vi "main（新）.vi"(8 "停止 2":bool) -> ()   [LabVIEW 2016]
uses:
  <vilib>/Averna/Notify Icon/NotifyIcon.llb/BalloonIcon.ctl
  <vilib>/Utility/miscctls.llb/LVPointTypeDef.ctl
  <vilib>/Utility/config.llb/Read Key (String).vi
  <vilib>/Utility/config.llb/Read Key (I32).vi
  <vilib>/Utility/config.llb/Read Key (Boolean).vi
  <vilib>/Utility/config.llb/Write Key (String).vi
  <vilib>/Utility/config.llb/Write Key (U32).vi
  <vilib>/Utility/config.llb/Write Key (I32).vi
  <vilib>/Utility/config.llb/Write Key (Boolean).vi
  <vilib>/Averna/Notify Icon/NotifyIcon.llb/GetSelectedItemEvent.vi
  <vilib>/Averna/Notify Icon/NotifyIcon.llb/SetVisible.vi
  <vilib>/Averna/Notify Icon/NotifyIcon.llb/SetMenuDefaultItem.vi
  <vilib>/Averna/Notify Icon/NotifyIcon.llb/SetTipText.vi
  <vilib>/Averna/Notify Icon/NotifyIcon.llb/NotifyIcon.lvclass
  <vilib>/Utility/config.llb/NI_LVConfig.lvlib
  data/FreeMem.dll
  <vilib>/ptbypt/NI_PtbyPt.lvlib
panel:
  in  "数据发送协议":enum16{"2005-212协议", "2017-212协议"}(ring)=enum."2017-212协议"
  in  "数据发送通道":enum16{"TCP", "VISA"}(ring)
  in  "baud rate":u32=9600 caption="波特率"
  in  "VISA resource name":refnum<visa-resource-name> caption="VISA资源名称"
  in  "查询质控数据起始时间":bool
  in  "返回主界面":bool
  out "零点核查索引起始时间":string
  out "跨度核查索引起始时间":string
  out "加标回收索引起始时间":string
  out "标样核查索引起始时间":string
  out "数据接收超时指示灯":bool
  in  "重发时间":T1(ring)
  in  "重发日期":T2(ring)
  in  "锁":bool
  in  "开机启动":bool
  in  "确定更改起始时间":bool
  in  "更改起始时间":bool
  in  "数据发送起始时间":timestamp format="%<%.3X\n%Y/%m/%d>T"
  in  "每周自动重发":bool=TRUE
  in  "确定":bool
  in  "返回":bool
  in  "PW":string
  in  "MN":string
  in  "PORT":string
  in  "IP":string
  in  "站点设备":string
  in  "站点名称":string
  out "设置超时时间/min":i32=1
  in  "实时数据发送时间间隔/min":u32=1
  out "空闲时间/s":string
  out "状态信息":T3={"1st Error to Convert "=63, "步骤 "=enum."打开连接", "元素"="实时数据", "TCP服务端掉线计数"=4, "TCP掉线时间节点"="2019/05/08 15:24:17"} {"1st Error to Convert" items=["无错误", "参数错误", "内存已满", "超出区域", "文件结束", "文件已打开", "一般文件IO错误", "未找到文件", "文件权限错误", "磁盘已满", "路径副本", "打开过多文件", "未启用", "未找到资源文件", "无法添加资源", "未找到资源", "未找到图像", "图像内存错误", "画笔不存在", "配置错误类型", "配置未找到解析段", "配置解析错误", "配置内存错误", "错误外部代码格式", "错误外部代码偏移量", "外部代码不存在", "空窗口", "销毁窗口错误", "空菜单", "打印已中止", "错误打印记录", "打印驱动程序错误", "打印时窗口错误", "打印时内存错误", "打印对话框错误", "一般打印错误", "无效设备引用句柄", "设备未找到", "设备参数错误", "设备单位错误", "无法打开设备", "设备调用已中止", "一般错误", "用户已取消", "对象ID过低", "对象ID过高", "对象不在堆中", "未知的堆", "错误DefProc ID", "DefProc不在表格中", "范围外信息", "空方法", "未知信息", "不支持管理器调用", "错误地址", "连接过程中", "连接超时", "连接过程中", "不支持网络属性", "网络错误", "正在使用的地址", "系统缺少内存", "连接已中止", "连接已拒绝", "连接未建立", "连接已建立", "连接已关闭", "初始化错误（交互应用程序管理器）", "错误事件发生", "等待无约束事件发生处理程序", "事件发生队列溢出", "错误路径", "未发出信号量", "未识别类型（交互应用程序管理器）"]}
  out "系统时间":string
  out "实时小时数据上传":bool
  out "系统状态改变":bool
  out "软件版本":string
  out "掉线指示":bool
  out "核查数据上传":bool
  out "通信状态":bool
  out "重发数据":bool
  out "配置信息":T4
  in  "参数配置":bool
  out "查询数据发送":bool
  out "读取报文显示":string
  out "发送报文显示":string
  out "心跳包":bool
  in  "参数数值":T5={"CODMn"=TRUE, "CODCr"=TRUE, "DO"=TRUE, "DOperNULL"=TRUE, "PH"=TRUE, "氨氮"=TRUE, "比电导率"=TRUE, "水温"=TRUE, "盐度(海水)"=TRUE, "浊度"=TRUE, "总氮"=TRUE, "总磷"=TRUE, "叶绿素a"=TRUE, "藻密度"=TRUE, "水位"=TRUE, "流速"=TRUE, "瞬时流量"=TRUE, "累积流量"=TRUE}
  in  "系统编码选择框":string(combo)="地表水质量监测"
  out "主队列输出":refnum<queue>
  in  "TCP掉线时间节点":string
  out "TCP服务端掉线计数":i32
  out "元素":string
  out "步骤":T6(ring)
  out "1st Error to Convert":i32(ring)=56 items=["无错误", "参数错误", "内存已满", "超出区域", "文件结束", "文件已打开", "一般文件IO错误", "未找到文件", "文件权限错误", "磁盘已满", "路径副本", "打开过多文件", "未启用", "未找到资源文件", "无法添加资源", "未找到资源", "未找到图像", "图像内存错误", "画笔不存在", "配置错误类型", "配置未找到解析段", "配置解析错误", "配置内存错误", "错误外部代码格式", "错误外部代码偏移量", "外部代码不存在", "空窗口", "销毁窗口错误", "空菜单", "打印已中止", "错误打印记录", "打印驱动程序错误", "打印时窗口错误", "打印时内存错误", "打印对话框错误", "一般打印错误", "无效设备引用句柄", "设备未找到", "设备参数错误", "设备单位错误", "无法打开设备", "设备调用已中止", "一般错误", "用户已取消", "对象ID过低", "对象ID过高", "对象不在堆中", "未知的堆", "错误DefProc ID", "DefProc不在表格中", "范围外信息", "空方法", "未知信息", "不支持管理器调用", "错误地址", "连接过程中", "连接超时", "连接过程中", "不支持网络属性", "网络错误", "正在使用的地址", "系统缺少内存", "连接已中止", "连接已拒绝", "连接未建立", "连接已建立", "连接已关闭", "初始化错误（交互应用程序管理器）", "错误事件发生", "等待无约束事件发生处理程序", "事件发生队列溢出", "错误路径", "未发出信号量", "未识别类型（交互应用程序管理器）"]
  out "QN":string
  out "时间QN":string
  out "系统编码ST":string
  out "命令编码CN":string
  out "密码PW":string
  out "设备编码MN":string
  out "拆分包及应答Flag":string
  out "数据":string
  in  "实时数据参数选择框":T7={"水样测量数据"=FALSE, "零点核查数据"=TRUE, "跨度核查数据"=TRUE, "加标回收数据"=TRUE, "平行样数据"=FALSE, "标样核查"=TRUE}
  out "数据输出":string
  in  "table元素":string
  out "数组":string[](array[string])
  out "数组 2":string[](array[string])
  out "空闲时间":dbl
  out "错误输出":errorcluster
  out "error out":errorcluster
  # "读取的参数区"
  # "水样测量数据"
  # "零点核查数据"
  # "跨度核查数据"
  # "加标回收数据"
  # "平行样数据"
  # "标样核查"
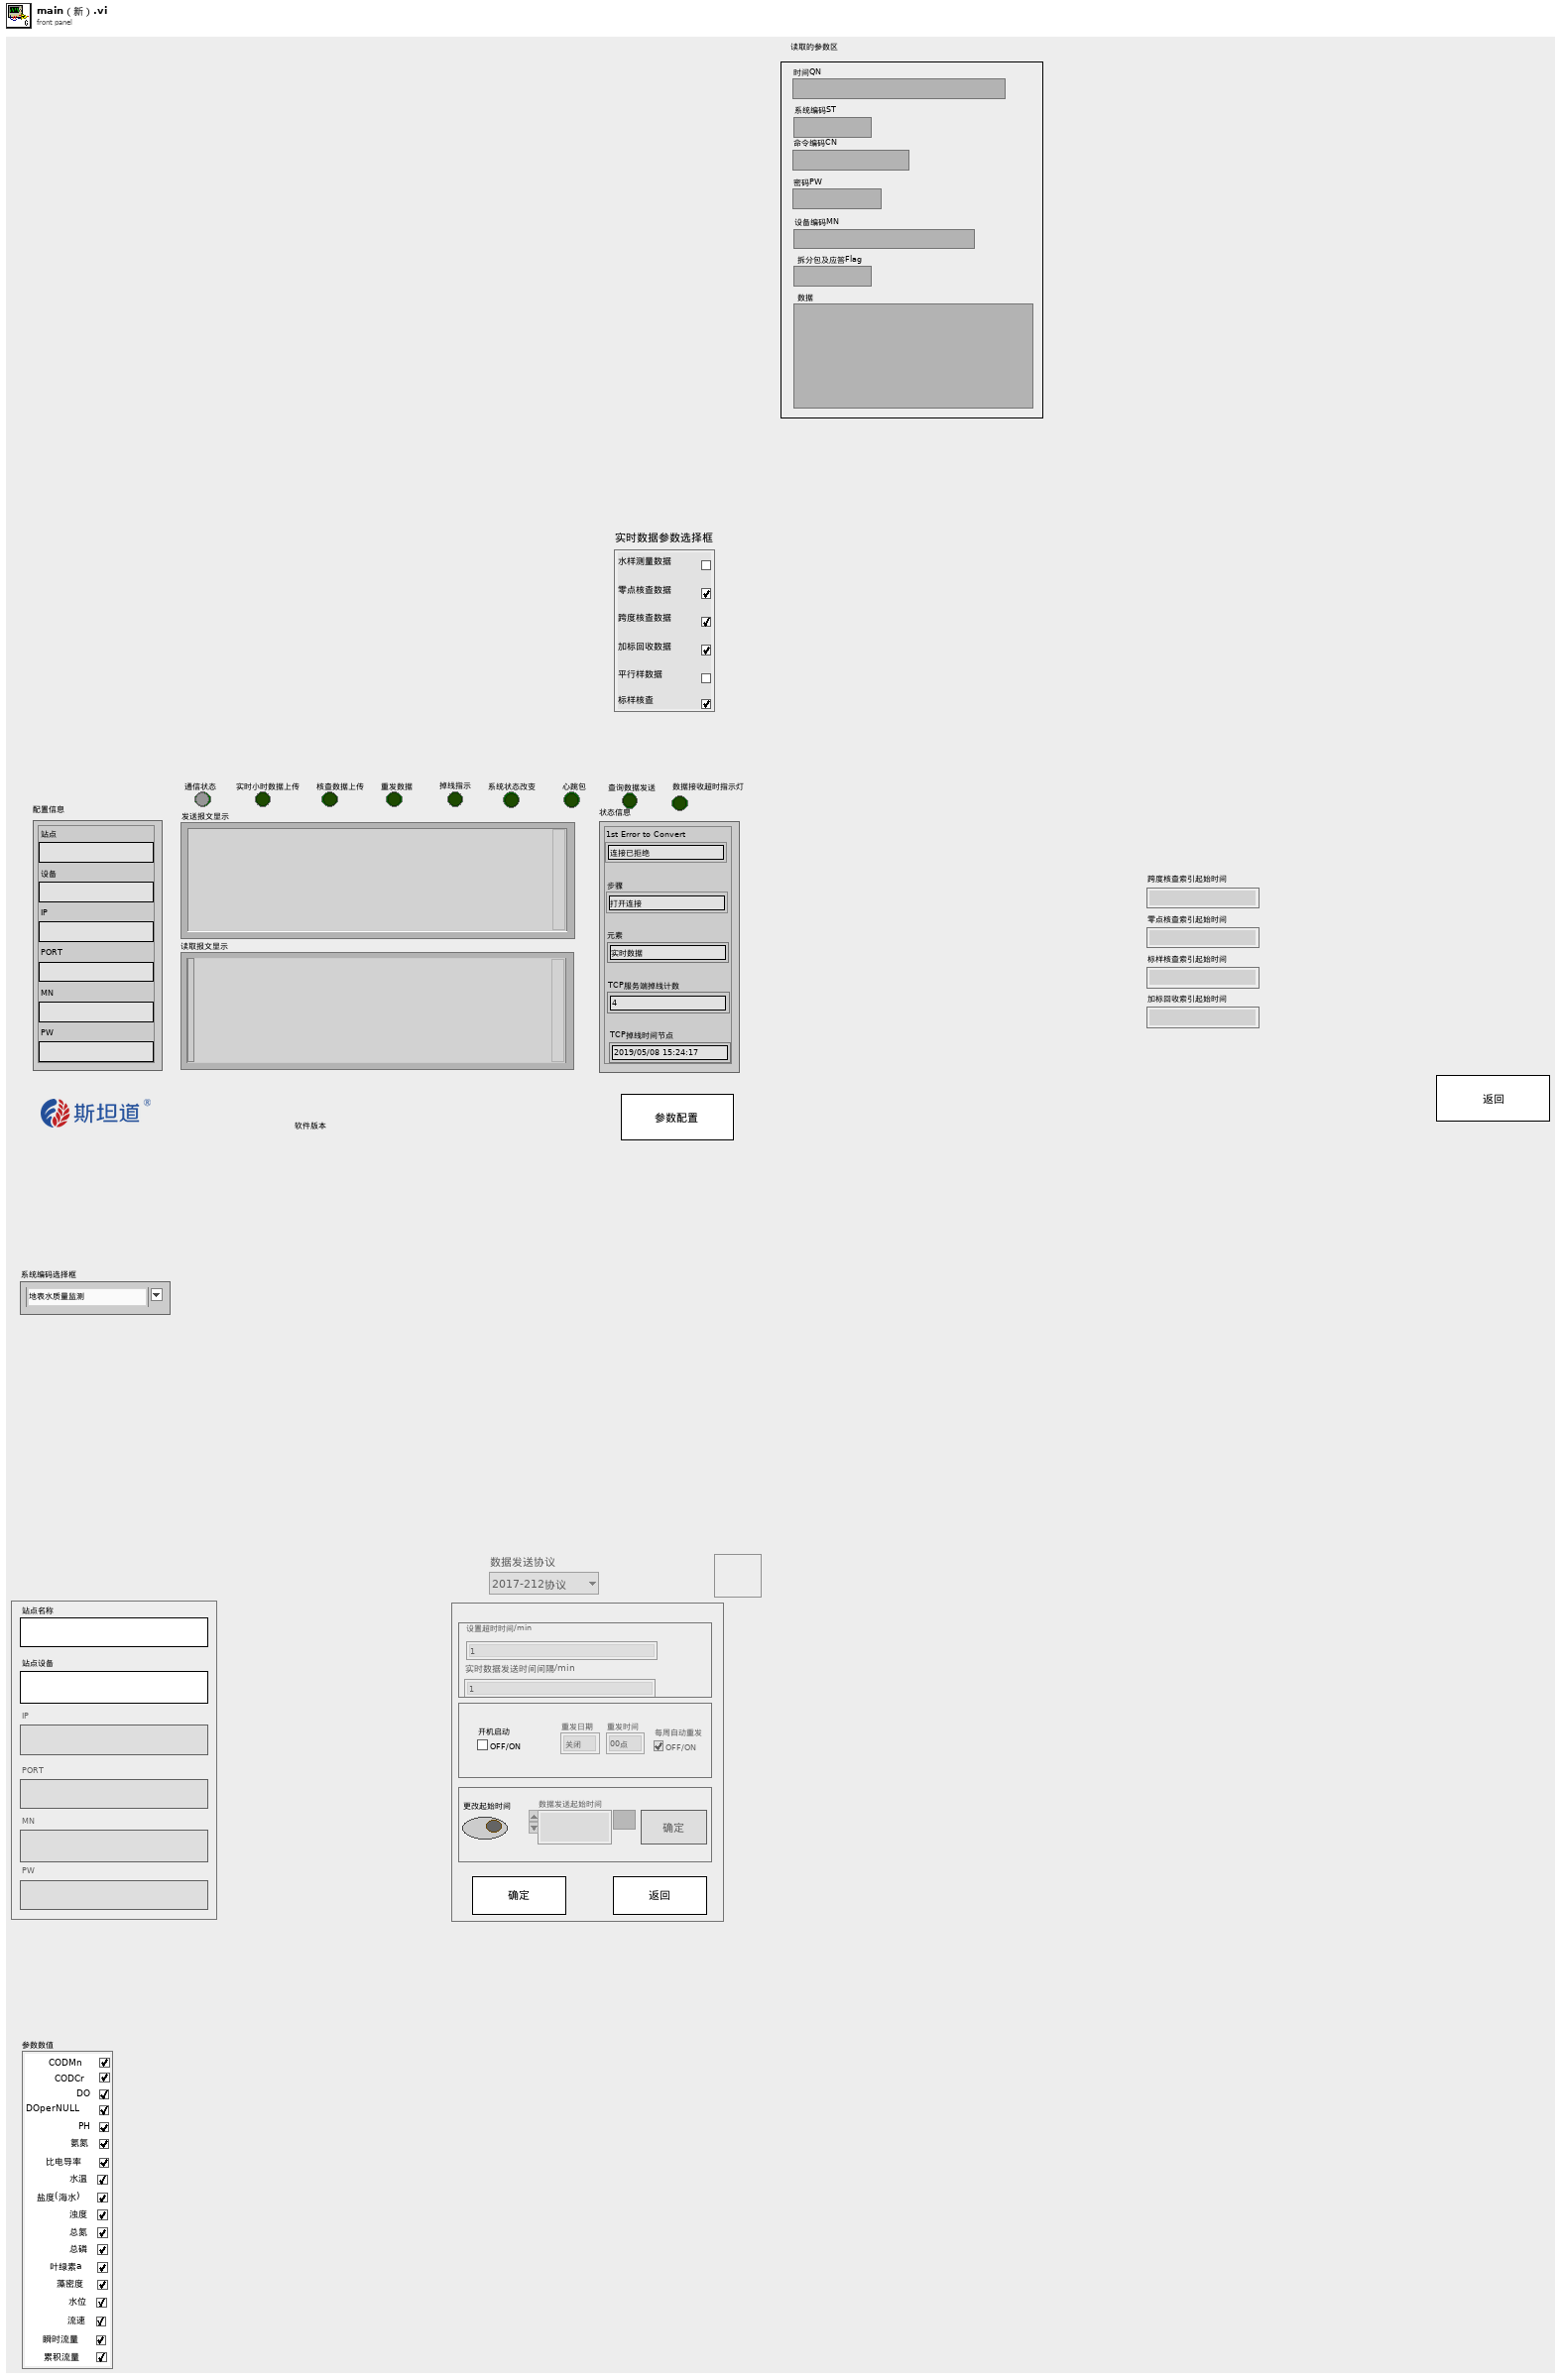
[diagram p1: front panel]
types:
  T1 = enum16{"00点", "01点", "02点", "03点", "04点", "05点", "06点", "07点", "08点", "09点", "10点", "11点", "12点", "13点", "14点", "15点", "16点", "17点", "18点", "19点", "20点", "21点", "22点", "23点"}
  T2 = enum16{"关闭", "星期日", "星期一", "星期二", "星期三", "星期四", "星期五", "星期六"}
  T3 = cluster{"1st Error to Convert ":i32, "步骤 ":enum16{"初始化", "打开连接", "表格比对", "发送数据", "读取数据", "数据处理"}, "元素":string, "TCP服务端掉线计数":i32, "TCP掉线时间节点":string}
  T4 = cluster{"站点":string, "设备":string, "IP":string, "PORT":string, "MN":string, "PW":string}
  T5 = cluster{"CODMn":bool, "CODCr":bool, "DO":bool, "DOperNULL":bool, "PH":bool, "氨氮":bool, "比电导率":bool, "水温":bool, "盐度(海水)":bool, "浊度":bool, "总氮":bool, "总磷":bool, "叶绿素a":bool, "藻密度":bool, "水位":bool, "流速":bool, "瞬时流量":bool, "累积流量":bool}
  T6 = enum16{"初始化", "打开连接", "表格比对", "发送数据", "读取数据", "数据处理"}
  T7 = cluster{"水样测量数据":bool, "零点核查数据":bool, "跨度核查数据":bool, "加标回收数据":bool, "平行样数据":bool, "标样核查":bool}
  T8 = typedef "NI_LVConfig.lvlib/Config Data RefNum.ctl" = refnum<k1>
  T9 = typedef "LVDateTimeRec.ctl" = cluster{"秒数的小数部分":dbl, "秒":i32, "分":i32, "时":i32, "日":i32, "月":i32, "年":i32, "天数（周）":i32, "天数（年）":i32, "DST":i32}
  T10 = cluster{"PH":string[][], "CODCr":string[][], "氨氮":string[][], "CODMn":string[][], "总氮":string[][], "总磷":string[][], "电导率":string[][], "水温":string[][], "DO":string[][], "浊度":string[][], "叶绿素":string[][], "藻密度":string[][], "DOper":string[][], "盐度":string[][], "水位":string[][], "流速":string[][], "瞬时流量":string[][], "累积流量":string[][]}
  T11 = typedef "LVPointTypeDef.ctl" = cluster{"Horizontal":i16, "Vertical":i16}
  T12 = enum8{"Enabled", "Disabled", "Disabled and Grayed Out"}
  T13 = typedef "imagedata.ctl" = cluster{"image type":i32, "image depth":i32, "image":u8[], "mask":u8[], "colors":u32[], "Rectangle":cluster{"left":i16, "top":i16, "right":i16, "bottom":i16}}
  T14 = enum32{"invalid app kind", "Development System", "Run Time System", "Student Edition", "Embedded LabVIEW", "Evaluation", "Custom"}
  T15 = enum32{"Invalid", "Standard", "Closed", "Hidden", "Minimized", "Maximized"}
  T16 = enum16{"水样测试", "小时数据", "日志信息", "报警信息", "零点核查", "标样核查", "平行样", "加标回收"}
  T17 = enum16{"CODMn", "CODCr", "氨氮", "总磷", "总氮", "数采仪"}
  T18 = cluster{"高锰酸盐":string, "化学需氧量":string, "氨氮":string, "总磷":string, "总氮":string, "数采仪":string, "高锰酸盐":bool, "化学需氧量":bool, "氨氮":bool, "总磷":bool, "总氮":bool, "数采仪":bool}
  T19 = typedef "NotifyIcon.lvlib/NotifyIcon.lvclass/BalloonIcon.ctl" = enum32{"None", "Information", "Warning", "Error"}
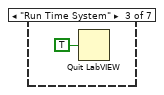
[diagram p5: hidden frame]
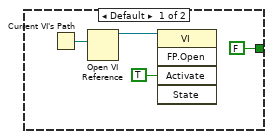
[diagram p10: hidden frame]
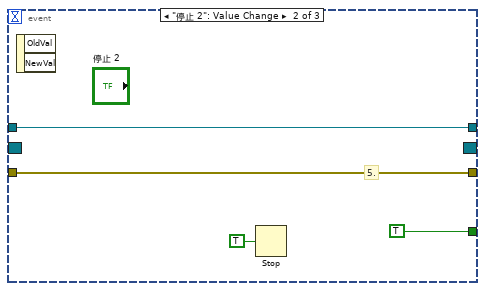
[diagram p11: hidden frame]
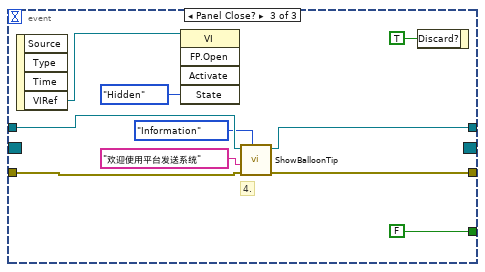
[diagram p12: hidden frame]
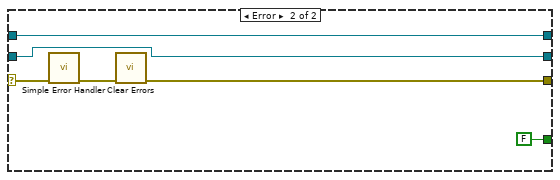
[diagram p13: hidden frame]
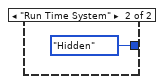
[diagram p14: hidden frame]
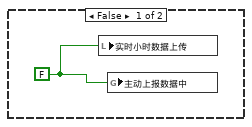
[diagram p15: hidden frame]
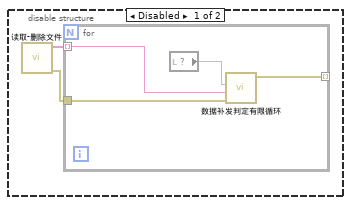
[diagram p16: hidden frame]
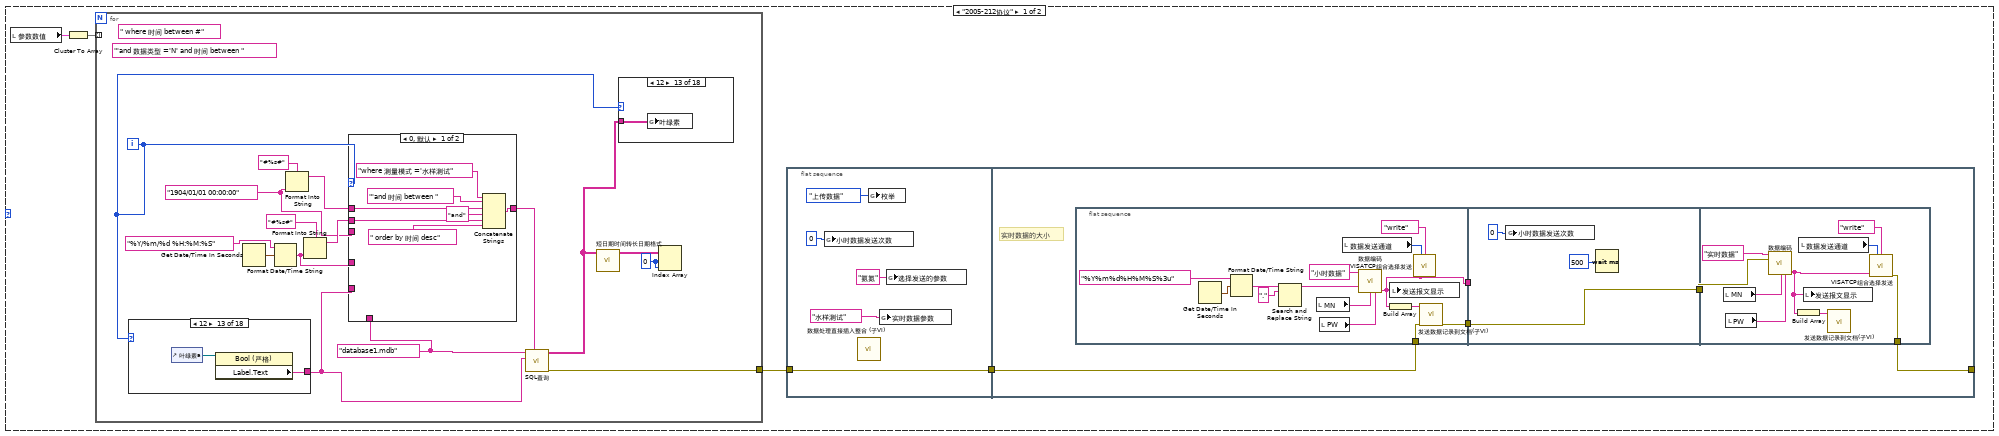
[diagram p17: hidden frame]
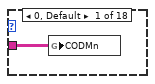
[diagram p18: hidden frame]
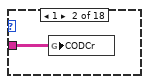
[diagram p19: hidden frame]
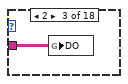
[diagram p20: hidden frame]
diagram:
  w23 = string[] ["OPEN线程一", "APP_SEPARATOR", "EXIT线程一"]
  (unwired) string[] ["CODMn", "CODCr", "DO", "DOper", "PH", "氨氮", "电导率", "水温", "盐度", "浊度", "总氮", "总磷", "叶绿素a", "藻密度", "水位", "流速", "瞬时流量", "累积流量"] ("查询参数数组")
  (unwired) 0 items=["无错误", "参数错误", "内存已满", "超出区域", "文件结束", "文件已打开", "一般文件IO错误", "未找到文件", "文件权限错误", "磁盘已满", "路径副本", "打开过多文件", "未启用", "未找到资源文件", "无法添加资源", "未找到资源", "未找到图像", "图像内存错误", "画笔不存在", "配置错误类型", "配置未找到解析段", "配置解析错误", "配置内存错误", "错误外部代码格式", "错误外部代码偏移量", "外部代码不存在", "空窗口", "销毁窗口错误", "空菜单", "打印已中止", "错误打印记录", "打印驱动程序错误", "打印时窗口错误", "打印时内存错误", "打印对话框错误", "一般打印错误", "无效设备引用句柄", "设备未找到", "设备参数错误", "设备单位错误", "无法打开设备", "设备调用已中止", "一般错误", "用户已取消", "对象ID过低", "对象ID过高", "对象不在堆中", "未知的堆", "错误DefProc ID", "DefProc不在表格中", "范围外信息", "空方法", "未知信息", "不支持管理器调用", "错误地址", "连接过程中", "连接超时", "连接过程中", "不支持网络属性", "网络错误", "正在使用的地址", "系统缺少内存", "连接已中止", "连接已拒绝", "连接未建立", "连接已建立", "连接已关闭", "初始化错误（交互应用程序管理器）", "错误事件发生", "等待无约束事件发生处理程序", "事件发生队列溢出", "错误路径", "未发出信号量", "未识别类型（交互应用程序管理器）"] ("1st Error to Convert")
  # "6."
  # "3."
  # "1."
  # "判定当数据没有传送完毕并掉线，将数据存储入临时表格"
  # "上传本地时间点的实时数据"
  # "目前时间太短，如果掉线了，数据存不了临时表格"
  # "3.表格中数据较多的情况下，数据补发送需要分批发送"
  # "1.发送数据过程中突然掉线（如果是查询之后的服务端掉线，不作处理；如果是整点主动上传时掉线，标记数据接收中断，然后数据存入表格）\n2.在查询过程中到了整点要发数据怎么处理（判定查询数据发送完全再进行出列队读取数据）\n3.一般情况掉线，数据存储入临时表格，上线了重发"
  # "获取需要发送的数据表"
  n1 = Cluster To Array(cluster="参数数值") -> (array=w33:bool[])
  n2 = for {
    tunnel: w33 -> [_] mode=indexing
    tunnel: [w73] -> w32
    i -> [w73]
    w62 = "线程一数据重发功能" ("section")
    n3 = case shown="8" w73 {
      tunnel: [w104 w106 w108 w110 w112 w114 w116 w118 w120 w122 w124 w126 w128 w130 w132 w134 w136 w138] -> w77
      frame 0, Default {
        n4 = control-ref of="CODMn"() -> (w105:refnum<vi>)
        n5 = property class="Bool (严格)"(reference=w105) -> ("Label.Text"=w104:string)  [unwired: 1 in, 2 out]
      }
      frame 1 {
        n6 = control-ref of="CODCr"() -> (w107:refnum<vi>)
        n7 = property class="Bool (严格)"(reference=w107) -> ("Label.Text"=w106:string)  [unwired: 1 in, 2 out]
      }
      frame 2 {
        n8 = control-ref of="DO"() -> (w109:refnum<vi>)
        n9 = property class="Bool (严格)"(reference=w109) -> ("Label.Text"=w108:string)  [unwired: 1 in, 2 out]
      }
      frame 3 {
        n10 = control-ref of="DOperNULL"() -> (w111:refnum<vi>)
        n11 = property class="Bool (严格)"(reference=w111) -> ("Label.Text"=w110:string)  [unwired: 1 in, 2 out]
      }
      frame 4 {
        n12 = control-ref of="PH"() -> (w113:refnum<vi>)
        n13 = property class="Bool (严格)"(reference=w113) -> ("Label.Text"=w112:string)  [unwired: 1 in, 2 out]
      }
      frame 5 {
        n14 = control-ref of="氨氮"() -> (w115:refnum<vi>)
        n15 = property class="Bool (严格)"(reference=w115) -> ("Label.Text"=w114:string)  [unwired: 1 in, 2 out]
      }
      frame 6 {
        n16 = control-ref of="比电导率"() -> (w117:refnum<vi>)
        n17 = property class="Bool (严格)"(reference=w117) -> ("Label.Text"=w116:string)  [unwired: 1 in, 2 out]
      }
      frame 7 {
        n18 = control-ref of="水温"() -> (w119:refnum<vi>)
        n19 = property class="Bool (严格)"(reference=w119) -> ("Label.Text"=w118:string)  [unwired: 1 in, 2 out]
      }
      frame 8 {
        n20 = control-ref of="盐度(海水)"() -> (w121:refnum<vi>)
        n21 = property class="Bool (严格)"(reference=w121) -> ("Label.Text"=w120:string)  [unwired: 1 in, 2 out]
      }
      frame 9 {
        n22 = control-ref of="浊度"() -> (w123:refnum<vi>)
        n23 = property class="Bool (严格)"(reference=w123) -> ("Label.Text"=w122:string)  [unwired: 1 in, 2 out]
      }
      frame 10 {
        n24 = control-ref of="总氮"() -> (w125:refnum<vi>)
        n25 = property class="Bool (严格)"(reference=w125) -> ("Label.Text"=w124:string)  [unwired: 1 in, 2 out]
      }
      frame 11 {
        n26 = control-ref of="总磷"() -> (w127:refnum<vi>)
        n27 = property class="Bool (严格)"(reference=w127) -> ("Label.Text"=w126:string)  [unwired: 1 in, 2 out]
      }
      frame 12 {
        n28 = control-ref of="叶绿素a"() -> (w129:refnum<vi>)
        n29 = property class="Bool (严格)"(reference=w129) -> ("Label.Text"=w128:string)  [unwired: 1 in, 2 out]
      }
      frame 13 {
        n30 = control-ref of="藻密度"() -> (w131:refnum<vi>)
        n31 = property class="Bool (严格)"(reference=w131) -> ("Label.Text"=w130:string)  [unwired: 1 in, 2 out]
      }
      frame 14 {
        n32 = control-ref of="水位"() -> (w133:refnum<vi>)
        n33 = property class="Bool (严格)"(reference=w133) -> ("Label.Text"=w132:string)  [unwired: 1 in, 2 out]
      }
      frame 15 {
        n34 = control-ref of="流速"() -> (w135:refnum<vi>)
        n35 = property class="Bool (严格)"(reference=w135) -> ("Label.Text"=w134:string)  [unwired: 1 in, 2 out]
      }
      frame 16 {
        n36 = control-ref of="瞬时流量"() -> (w137:refnum<vi>)
        n37 = property class="Bool (严格)"(reference=w137) -> ("Label.Text"=w136:string)  [unwired: 1 in, 2 out]
      }
      frame 17 {
        n38 = control-ref of="累积流量"() -> (w139:refnum<vi>)
        n39 = property class="Bool (严格)"(reference=w139) -> ("Label.Text"=w138:string)  [unwired: 1 in, 2 out]
      }
    }
    n40 = call <vilib>:"Application Directory.vi"() -> ("Application Directory"=w83:path)
    n41 = Build Path(base path=w83, name or relative path="data\\Set.ini" ("名称或相对路径")) -> (appended path=w81:path)
    n42 = call <vilib>:"Open Config Data.vi"("configuration file path"=w81) -> ("error out"=w79:errorcluster, "refnum"=w80:T8)  [unwired: 8 in, 1 out]
    n43 = call-poly <vilib>:"Read Key.vi"("section"="线程一数据搜索起始时间", "error in (no error)"=w79, "key"=w77, "refnum"=w80) -> ("error out"=w71:errorcluster, "value"=w74:string, "refnum out"=w72:T8)  [unwired: 4 in, 1 out]
    n44 = Empty String/Path?(string/path=w74) -> (empty?=w76:bool)
    n45 = case shown="真" w76 {
      tunnel: [w84 "1904/01/01 00:00:00"] -> w75
      tunnel: w74 -> [w84 _]
      frame False {
      }
      frame True {
      }
    }
    n46 = call-poly <vilib>:"Read Key.vi"("section"=w62, "error in (no error)"=w71, "key"="重发功能", "refnum"=w72) -> ("error out"=w65:errorcluster, "value"=w69:bool, "refnum out"=w66:T8)  [unwired: 4 in, 1 out]
    n47 = local write "每周自动重发"(w69) -> ()
    n48 = call-poly <vilib>:"Read Key.vi"("section"=w62, "error in (no error)"=w65, "key"="重发日期", "refnum"=w66) -> ("error out"=w63:errorcluster, "value"=w59:i32, "refnum out"=w64:T8)  [unwired: 4 in, 1 out]
    n49 = local write "重发日期"(w59) -> ()
    n50 = case shown="0, 默认" w73 {
      tunnel: w75 -> [w86 w87 w88 w89 w90 w91 w92 w93 w94 w95 w96 w97 w98 w99 w100 w101 w102 w103]
      frame 0, Default {
        n51 = global write "全局 水样时间.vi" "time1"(w86) -> ()
      }
      frame 1 {
        n52 = global write "全局 水样时间.vi" "time2"(w87) -> ()
      }
      frame 2 {
        n53 = global write "全局 水样时间.vi" "time3"(w88) -> ()
      }
      frame 3 {
        n54 = global write "全局 水样时间.vi" "time4"(w89) -> ()
      }
      frame 4 {
        n55 = global write "全局 水样时间.vi" "time5"(w90) -> ()
      }
      frame 5 {
        n56 = global write "全局 水样时间.vi" "time6"(w91) -> ()
      }
      frame 6 {
        n57 = global write "全局 水样时间.vi" "time7"(w92) -> ()
      }
      frame 7 {
        n58 = global write "全局 水样时间.vi" "time8"(w93) -> ()
      }
      frame 8 {
        n59 = global write "全局 水样时间.vi" "time9"(w94) -> ()
      }
      frame 9 {
        n60 = global write "全局 水样时间.vi" "time10"(w95) -> ()
      }
      frame 10 {
        n61 = global write "全局 水样时间.vi" "time11"(w96) -> ()
      }
      frame 11 {
        n62 = global write "全局 水样时间.vi" "time12"(w97) -> ()
      }
      frame 12 {
        n63 = global write "全局 水样时间.vi" "time13"(w98) -> ()
      }
      frame 13 {
        n64 = global write "全局 水样时间.vi" "time14"(w99) -> ()
      }
      frame 14 {
        n65 = global write "全局 水样时间.vi" "time15"(w100) -> ()
      }
      frame 15 {
        n66 = global write "全局 水样时间.vi" "time16"(w101) -> ()
      }
      frame 16 {
        n67 = global write "全局 水样时间.vi" "time17"(w102) -> ()
      }
      frame 17 {
        n68 = global write "全局 水样时间.vi" "time18"(w103) -> ()
      }
    }
    n69 = call-poly <vilib>:"Read Key.vi"("section"=w62, "error in (no error)"=w63, "key"="重发时间", "refnum"=w64) -> ("error out"=w60:errorcluster, "value"=w58:i32, "refnum out"=w61:T8)  [unwired: 4 in, 1 out]
    n70 = local write "重发时间"(w58) -> ()
    n71 = call <vilib>:"Close Config Data.vi"("error in (no error)"=w60, "refnum"=w61) -> ()  [unwired: 8 in, 2 out]
  }
  n72 = Obtain Queue(name (unnamed)="数据发送" ("名称（未命名）"), element data type="") -> (queue out=w38:refnum<queue>, error out=w37:errorcluster)  [unwired: 3 in, 1 out]
  n73 = Obtain Queue(name (unnamed)="实时数据参数选择" ("名称（未命名）"), element data type="") -> (queue out=w39:refnum<queue>, error out=w36:errorcluster)  [unwired: 3 in, 1 out]
  n74 = while {
    tunnel: w38 -> [w142]
    stop <- FALSE stop-if-true
    # "和工控机通讯系统状态改变主动上传"
    # "整点发送小时数据(禁用）"
    n75 = Multiply(x=u32 1, y=u32 1000 ("等待时间（毫秒）")) -> (x*y=w148:u32)
    n76 = case shown="真" "每周自动重发" {
      frame False {
      }
      frame True {
        (unwired) T1."00点"
        (unwired) T2."关闭"
        n77 = Get Date/Time In Seconds() -> (seconds since 1Jan1904=w211:timestamp)
        n78 = Seconds To Date/Time(time stamp (now)=w211) -> (date time rec=w205:T9)  [unwired: 1 in]
        n79 = Unbundle By Name(w205) -> ("天数（周）"=w210:i32, "时"=w200:i32, "分"=w209:i32)
        n80 = Equal To 0?(x=w209) -> (x = 0?=w206:bool)
        n81 = Equal?(x=w210, y="重发日期") -> (x = y?=w208:bool)
        n82 = Equal?(x=w200, y="重发时间") -> (x = y?=w207:bool)
        n83 = Compound Arithmetic op=AND ("复合运算")(w208, w207, w206) -> (w204:bool)
        n84 = call <vilib>:"Boolean Crossing PtByPt.vi"("direction"=enum16{"either", "false-true", "true-false"}."false-true", "input"=w204) -> ("crossing"=w203:bool)  [unwired: 1 in]
        n85 = case shown="真" w203 {
          tunnel: w205 -> [_ w213]
          frame False {
          }
          frame True {
            n86 = local read "参数数值"() -> (w218:T5)
            n87 = Unbundle By Name(w213) -> ("日"=w216:i32)
            n88 = Cluster To Array(cluster=w218) -> (array=w219:bool[])
            n89 = Subtract(x=w216, y=7) -> (x-y=w214:i32)
            n90 = Bundle By Name(cluster=w213, "日"=w214) -> (w217:T9)
            n91 = Date/Time To Seconds(2:w217) -> (0:w212:timestamp)  [unwired: 1 in]
            n92 = for {
              tunnel: w219 -> [_] mode=indexing
              tunnel: w212 -> [w220]
              i -> [w221]
              n93 = Format Date/Time String(time format string (%c)="%Y/%m/%d %H:%M:%S" ("时间格式字符串(%c)"), seconds (now)=w220) -> (date/time string=w222:string)  [unwired: 1 in]
              n94 = case shown="16" w221 {
                tunnel: w222 -> [w224 w225 w226 w227 w228 w229 w230 w231 w232 w233 w234 w235 w236 w237 w238 w239 w240 w241]
                frame 0, Default {
                  n95 = global write "全局 水样时间.vi" "time1"(w224) -> ()
                }
                frame 1 {
                  n96 = global write "全局 水样时间.vi" "time2"(w225) -> ()
                }
                frame 2 {
                  n97 = global write "全局 水样时间.vi" "time3"(w226) -> ()
                }
                frame 3 {
                  n98 = global write "全局 水样时间.vi" "time4"(w227) -> ()
                }
                frame 4 {
                  n99 = global write "全局 水样时间.vi" "time5"(w228) -> ()
                }
                frame 5 {
                  n100 = global write "全局 水样时间.vi" "time6"(w229) -> ()
                }
                frame 6 {
                  n101 = global write "全局 水样时间.vi" "time7"(w230) -> ()
                }
                frame 7 {
                  n102 = global write "全局 水样时间.vi" "time8"(w231) -> ()
                }
                frame 8 {
                  n103 = global write "全局 水样时间.vi" "time9"(w232) -> ()
                }
                frame 9 {
                  n104 = global write "全局 水样时间.vi" "time10"(w233) -> ()
                }
                frame 10 {
                  n105 = global write "全局 水样时间.vi" "time11"(w234) -> ()
                }
                frame 11 {
                  n106 = global write "全局 水样时间.vi" "time12"(w235) -> ()
                }
                frame 12 {
                  n107 = global write "全局 水样时间.vi" "time13"(w236) -> ()
                }
                frame 13 {
                  n108 = global write "全局 水样时间.vi" "time14"(w237) -> ()
                }
                frame 14 {
                  n109 = global write "全局 水样时间.vi" "time15"(w238) -> ()
                }
                frame 15 {
                  n110 = global write "全局 水样时间.vi" "time16"(w239) -> ()
                }
                frame 16 {
                  n111 = global write "全局 水样时间.vi" "time17"(w240) -> ()
                }
                frame 17 {
                  n112 = global write "全局 水样时间.vi" "time18"(w241) -> ()
                }
              }
            }
          }
        }
      }
    }
    n113 = Wait (ms)(milliseconds to wait=w148) -> ()  [unwired: 1 out]
    n114 = call "Modbus Master.vi"("Unit ID"=u8 1, "读取写入选择"="读取") -> ("register values"=w143:u16[], "error out"=w140:errorcluster)  [unwired: 8 in]
    n115 = case shown="无错误" w140 {
      tunnel: w143 -> [w152 _]
      tunnel: w142 -> [w150 _]
      frame No Error {
        # "防止由于MBtcp错误导致状态为0发送至平台"
        n116 = global read "全局1.vi" "register values"() -> (w151:u16[])
        n117 = flat-sequence {
          tunnel: w152 -> [w158]
          tunnel: w151 -> [w178]
          tunnel: w150 -> [w154]
          tunnel: [w158] -> w153
          tunnel: w153 -> [w198]
          frame #0 {
            n118 = Index Array(array=w158) -> (element #1=w165:u16, element #2=w177:u16, element #3=w176:u16, element #4=w175:u16, element #5=w174:u16, element #6=w173:u16, element #7=w163:u16, element #8=w157:u16)  [unwired: 8 in]
            n119 = Index Array(array=w178) -> (element #1=w164:u16, element #2=w172:u16, element #3=w171:u16, element #4=w170:u16, element #5=w169:u16, element #6=w168:u16, element #7=w162:u16, element #8=w156:u16)  [unwired: 8 in]
            n120 = Build Array(w177, w176, w175, w174, w173) -> (w167:u16[])
            n121 = Build Array(w172, w171, w170, w169, w168) -> (w166:u16[])
            n122 = Not Equal?(x=w165, y=w164) -> (x != y?=w160:bool)
            n123 = Not Equal?(x=w163, y=w162) -> (x != y?=w161:bool)
            n124 = Not Equal?(x=w157, y=w156) -> (x != y?=w155:bool)
            n125 = Not Equal?(x=w167, y=w166) -> (x != y?=w159:bool[])
            n126 = while {
              tunnel: w154 -> [w187]
              tunnel: w159 -> [w184] mode=indexing
              i -> [w186]
              stop <- w182 stop-if-true
              n127 = Greater Or Equal?(x=w186, y=4) -> (x >= y?=w183:bool)
              n128 = Or(x=w184, y=w183) -> (x .or. y?=w182:bool)
              n129 = case shown="真" w184 {
                tunnel: w187 -> [_ w189]
                frame False {
                }
                frame True {
                  n130 = local write "系统状态改变"(TRUE ("系统状态改变")) -> ()
                  n131 = Enqueue Element(queue=w189, element="系统状态" ("元素")) -> ()  [unwired: 2 in, 3 out]
                }
              }
            }
            n132 = case shown="真" w160 {
              tunnel: w154 -> [_ w195]
              frame False {
              }
              frame True {
                n133 = Enqueue Element(queue=w195, element="运行模式" ("元素")) -> ()  [unwired: 2 in, 3 out]
                "系统状态改变" <- TRUE
              }
            }
            n134 = case shown="真" w155 {
              tunnel: w154 -> [_ w180]
              frame False {
              }
              frame True {
                n135 = local write "系统状态改变"(TRUE ("系统状态改变")) -> ()
                n136 = Enqueue Element(queue=w180, element="超标留样" ("元素")) -> ()  [unwired: 2 in, 3 out]
              }
            }
            n137 = case shown="真" w161 {
              tunnel: w154 -> [_ w192]
              frame False {
              }
              frame True {
                n138 = local write "系统状态改变"(TRUE ("系统状态改变")) -> ()
                n139 = Enqueue Element(queue=w192, element="测量周期" ("元素")) -> ()  [unwired: 2 in, 3 out]
              }
            }
          }
          frame #1 {
            n140 = global write "全局1.vi" "register values"(w198) -> ()
            n141 = local write "系统状态改变"(FALSE ("系统状态改变")) -> ()
          }
        }
      }
      frame Error {
      }
    }
  }
  n142 = while {
    tunnel: w38 -> [w255]
    stop <- FALSE stop-if-true
    # "核查和质控数据的定期发送在实时数据周期上传"
    # "指定周期发一次核查数据"
    n143 = local read "查询数据发送"() -> (w250:bool)
    n144 = local read "实时小时数据上传"() -> (w254:bool)
    n145 = local read "重发数据"() -> (w251:bool)
    n146 = Multiply(x="实时数据发送时间间隔/min", y=u32 60000 ("等待时间（毫秒）")) -> (x*y=w258:u32)
    n147 = local read "步骤"() -> (w249:T6)
    n148 = Not(x=w250) -> (.not. x?=w246:bool)
    n149 = Wait (ms)(milliseconds to wait=w258) -> ()  [unwired: 1 out]
    n150 = Not(x=w251) -> (.not. x?=w245:bool)
    n151 = Not(x=w254) -> (.not. x?=w252:bool)
    n152 = First Call?() -> (First Call?: T/F=w256:bool)
    n153 = Equal?(x=w249, y=T6."读取数据" ("步骤")) -> (x = y?=w247:bool)
    n154 = case shown="真" w256 {
      tunnel: w255 -> [_ _]
      frame False {
      }
      frame True {
        w274 = "1994/01/01 00:00:00"
        n155 = global write "全局 时间2.vi" "跨度核查索引起始时间"(w274) -> ()
        n156 = global write "全局 时间2.vi" "零点核查索引起始时间"(w274) -> ()
        n157 = global write "全局 时间2.vi" "平行样索引起始时间"(w274) -> ()
        n158 = global write "全局 时间2.vi" "加标回收索引起始时间"(w274) -> ()
        n159 = global write "全局 时间2.vi" "标样核查索引起始时间"(w274) -> ()
      }
    }
    n160 = local read "数据发送协议"() -> (w244:enum16{"2005-212协议", "2017-212协议"})
    n161 = Equal?(x=w244, y=enum16{"2005-212协议", "2017-212协议"}."2017-212协议" ("数据发送协议")) -> (x = y?=w242:bool)
    n162 = Compound Arithmetic op=AND ("复合运算")(w242, w245, w246, w247, w252) -> (w253:bool)
    n163 = case shown="真" w253 {
      tunnel: w255 -> [_ w270]
      frame False {
      }
      frame True {
        n164 = call "实时数据参数入列队.vi"("发送实时数据选择框"="实时数据参数选择框") -> ("错误输出"=w272:errorcluster)  [unwired: 10 in]
        n165 = call <vilib>:"Clear Errors.vi"("error in (no error)"=w272) -> ()  [unwired: 5 in, 2 out]
        n166 = Enqueue Element(queue=w270, element="send" ("元素")) -> (queue out=w267:refnum<queue>, error out=w266:errorcluster)  [unwired: 2 in, 1 out]
        n167 = Enqueue Element(queue=w267, element="操作日志" ("元素"), error in (no error)=w266) -> (queue out=w264:refnum<queue>, error out=w263:errorcluster)  [unwired: 1 in, 1 out]
        n168 = Enqueue Element(queue=w264, element="仪器参数" ("元素"), error in (no error)=w263) -> (queue out=w262:refnum<queue>, error out=w261:errorcluster)  [unwired: 1 in, 1 out]
        n169 = Enqueue Element(queue=w262, element="报警信息" ("元素"), error in (no error)=w261) -> ()  [unwired: 1 in, 3 out]
      }
    }
  }
  n170 = while "While循环" {
    tunnel: w38 -> [w287]
    tunnel: w39 -> [w291]
    tunnel: w37 -> [w290]
    tunnel: w36 -> [w289]
    stop <- FALSE stop-if-true
    # "判定数据发送时要发送实时数据"
    # "所有的主动上传数据都是有数据才会上传"
    n171 = Get Queue Status(queue=w287) -> (# elements in queue=w279:i32)  [unwired: 2 in, 7 out]
    n172 = local read "查询数据发送"() -> (w285:bool)
    n173 = global read "全局 数据发送重叠.vi" "主动上报数据中"() -> (w277:bool)
    n174 = local read "重发数据"() -> (w276:bool)
    n175 = Not Equal To 0?(x=w279) -> (x != 0?=w286:bool)
    n176 = And(x=w286, y=w285) -> (x .and. y?=w278:bool)
    n177 = call <vilib>:"Boolean Crossing PtByPt.vi"("direction"=enum16{"either", "false-true", "true-false"}."false-true", "input"=w278) -> ("crossing"=w284:bool)  [unwired: 1 in]
    n178 = Not(x=w277) -> (.not. x?=w281:bool)
    n179 = Not(x=w276) -> (.not. x?=w275:bool)
    n180 = Not(x=w285) -> (.not. x?=w282:bool)
    n181 = case shown="真" w284 {
      frame False {
      }
      frame True {
        n182 = Get Date/Time In Seconds() -> (seconds since 1Jan1904=w294:timestamp)
        n183 = Format Date/Time String(time format string (%c)="%Y%m%d%H%M%S%3u" ("时间格式字符串(%c)"), seconds (now)=w294) -> (date/time string=w298:string)  [unwired: 1 in]
        n184 = Search and Replace String(input string=w298, search string="." ("搜索字符串")) -> (result string=w297:string)  [unwired: 6 in, 3 out]
        n185 = call "格式时间字符串.vi"("字符串"=w297) -> ("连接的字符串"=w293:string)  [unwired: 10 in]
        n186 = global write "全局 数据发送重叠.vi" "数据发送重叠开始时间戳"(w293) -> ()
      }
    }
    n187 = Compound Arithmetic op=AND ("复合运算")(w282, w281, w275) -> (w280:bool)
    n188 = Wait (ms)(milliseconds to wait=u32 1000 ("等待时间（毫秒）")) -> ()  [unwired: 1 out]
    n189 = case shown="真" w280 {
      tunnel: w287 -> [_ w308]
      tunnel: w291 -> [_ w307]
      tunnel: w290 -> [_ w306]
      tunnel: w289 -> [_ w305]
      tunnel: w279 -> [_ w301]
      tunnel: w278 -> [_ w300]
      frame False {
        n190 = local write "核查数据上传"(FALSE ("数据上传")) -> ()
      }
      frame True {
        n191 = Equal To 0?(x=w301) -> (x = 0?=w302:bool)
        n192 = global write "全局 数据发送重叠.vi" "数据发送重叠"(w300) -> ()
        n193 = Not(x=w302) -> (.not. x?=w303:bool)
        n194 = local write "核查数据上传"(w303) -> ()
        n195 = Dequeue Element(queue=w308, error in (no error)=w306) -> (element=w304:string)  [unwired: 1 in, 3 out]
        n196 = case shown="\"环境参数\"" w304 {
          tunnel: w307 -> [_ w310 _ _ _ _ _ _ _ _ _]
          tunnel: w305 -> [_ w309 _ _ _ _ _ _ _ _ _]
          frame "假", Default {
          }
          frame "send" {
            # "间隔时间上传"
            n197 = while {
              tunnel: w310 -> [w314]
              tunnel: w309 -> [w311]
              stop <- w315 stop-if-true
              n198 = Dequeue Element(queue=w314, error in (no error)=w311) -> (queue out=w313:refnum<queue>, element=w316:string)  [unwired: 1 in, 2 out]
              n199 = case shown="\"平行样\"" w316 {
                tunnel: [_ _ _ w414 _ _ w513] -> w315
                tunnel: w313 -> [_ _ _ _ _ _ w516]
                frame "水样测试" {
                  n200 = flat-sequence {
                    frame #0 {
                      n201 = global write "全局 小时数据发送次数.vi" "小时数据发送次数"(0 ("小时数据发送次数")) -> ()
                      n202 = global write "全局 实时数据参数.vi" "实时数据参数"("水样测试") -> ()
                      n203 = global write "全局1.vi" "枚举"(enum16{"返回请求应答", "上传数据", "返回执行结果"}."上传数据" ("枚举")) -> ()
                    }
                    frame #1 {
                      n204 = call "从数据库获取数据通用可配置(子VI).vi"("table输入"="实时数据" ("新元素/子数组"), "列队名（唯一）"="a") -> ()  [unwired: 8 in, 2 out]
                    }
                    frame #2 {
                      n205 = call "实时小时数据处理整合 (子VI).vi"("枚举"=enum16{"实时数据排序", "小时数据排序"}."实时数据排序") -> ("已排序的数组"=w323:string[])  [unwired: 10 in]
                      n206 = Array Size(array=w323) -> (size(s)=w324:i32)
                      n207 = global write "全局 数据数组大小.vi" "数据数组大小"(w324) -> ()
                    }
                    frame #3 {
                      n208 = while {
                        stop <- w329 stop-if-true
                        n209 = property on="TCP服务端掉线计数" class="DigNum (严格)"() -> ("Value"=w332:i32)  [unwired: 2 in, 2 out]
                        n210 = Greater Or Equal?(x=w332, y=1) -> (x >= y?=w331:bool)
                        n211 = case shown="假" w331 {
                          frame False {
                            n212 = global read "全局 数据数组大小.vi" "数据数组大小"() -> (w334:i32)
                            n213 = Greater Than 0?(x=w334) -> (x > 0?=w335:bool)
                            n214 = case shown="真" w335 {
                              frame False {
                              }
                              frame True {
                                n215 = local read "MN"() -> (w341:string)
                                n216 = local read "PW"() -> (w340:string)
                                n217 = local read "数据发送通道"() -> (w339:enum16{"TCP", "VISA"})
                                n218 = call "数据编码.vi"("table输入"="实时数据" ("新元素/子数组"), "MN"=w341, "PW"=w340) -> ("通讯包字符串"=w336:string)  [unwired: 11 in, 1 out]
                                n219 = local write "发送报文显示"(w336) -> ()
                                n220 = call "VISATCP组合选择发送.vi"("数据发送通道"=w339, "命令"="write", "写入缓冲区"=w336) -> ("错误输出"=→"错误输出":errorcluster)  [unwired: 9 in, 3 out]
                                n221 = Build Array(w336) -> (w343:string[])
                                n222 = call "发送数据记录到文档(子VI).vi"("数组"=w343) -> ()  [unwired: 9 in, 1 out]
                                "核查数据上传" <- TRUE ("主动数据上传")
                              }
                            }
                          }
                          frame True {
                          }
                        }
                        n223 = Wait (ms)(milliseconds to wait=u32 500 ("等待时间（毫秒）")) -> ()  [unwired: 1 out]
                        n224 = global read "全局 数据数组大小.vi" "数据数组大小"() -> (w326:i32)
                        n225 = global read "全局 小时数据发送次数.vi" "小时数据发送次数"() -> (w330:i32)
                        n226 = Decrement(x=w326) -> (x-1=w325:i32)
                        n227 = Greater Or Equal?(x=w330, y=w325) -> (x >= y?=w328:bool)
                        n228 = Compound Arithmetic op=OR ("复合运算")(w328) -> (w329:bool)
                      }
                    }
                  }
                }
                frame "空白测试" {
                  n229 = flat-sequence {
                    frame #0 {
                      n230 = global write "全局 小时数据发送次数.vi" "小时数据发送次数"(0 ("小时数据发送次数")) -> ()
                      n231 = global write "全局 实时数据参数.vi" "实时数据参数"("空白测试") -> ()
                      n232 = global write "全局1.vi" "枚举"(enum16{"返回请求应答", "上传数据", "返回执行结果"}."上传数据" ("枚举")) -> ()
                    }
                    frame #1 {
                      n233 = call "从数据库获取数据通用可配置(子VI).vi"("table输入"="实时数据" ("新元素/子数组"), "列队名（唯一）"="b") -> ()  [unwired: 8 in, 2 out]
                    }
                    frame #2 {
                      n234 = call "数据处理整合 (子VI).vi"("枚举"=enum16{"实时数据排序", "小时数据排序"}."实时数据排序") -> ("已排序的数组"=w352:string[])  [unwired: 10 in]
                      n235 = Array Size(array=w352) -> (size(s)=w351:i32)
                      n236 = global write "全局 数据数组大小.vi" "数据数组大小"(w351) -> ()
                    }
                    frame #3 {
                      n237 = while {
                        stop <- w355 stop-if-true
                        n238 = property on="TCP服务端掉线计数" class="DigNum (严格)"() -> ("Value"=w359:i32)  [unwired: 2 in, 2 out]
                        n239 = Greater Or Equal?(x=w359, y=1) -> (x >= y?=w358:bool)
                        n240 = case shown="假" w358 {
                          frame False {
                            n241 = global read "全局 数据数组大小.vi" "数据数组大小"() -> (w362:i32)
                            n242 = Greater Than 0?(x=w362) -> (x > 0?=w361:bool)
                            n243 = case shown="真" w361 {
                              frame False {
                              }
                              frame True {
                                n244 = global read "插值后的新数组.vi" "插值后的数组元素"() -> (w373:T10)
                                n245 = global read "全局 数据数组大小.vi" "数据数组大小"() -> (w374:i32)
                                n246 = local write "核查数据上传"(TRUE ("数据上传")) -> ()
                                n247 = local read "MN"() -> (w368:string)
                                n248 = local read "PW"() -> (w367:string)
                                n249 = local read "数据发送通道"() -> (w366:enum16{"TCP", "VISA"})
                                n250 = call "数据编码.vi"("table输入"="实时数据" ("新元素/子数组"), "MN"=w368, "PW"=w367) -> ("通讯包字符串"=w364:string)  [unwired: 11 in, 1 out]
                                n251 = Decrement(x=w374) -> (x-1=w375:i32)
                                n252 = Unbundle By Name(w373) -> ("氨氮"=w372:string[][])
                                n253 = local write "发送报文显示"(w364) -> ()
                                n254 = Build Array(w364) -> (w377:string[])
                                n255 = call "VISATCP组合选择发送.vi"("数据发送通道"=w366, "命令"="write", "写入缓冲区"=w364) -> ("错误输出"=w363:errorcluster)  [unwired: 9 in, 3 out]
                                n256 = Index Array(array=w372, index (row)=w375, index (col)=0 ("禁用的索引 (列)")) -> (element=w370:string)
                                n257 = call "发送数据记录到文档(子VI).vi"("数组"=w377) -> ()  [unwired: 9 in, 1 out]
                                n258 = local write "错误输出"(w363) -> ()
                                n259 = call "日期时间字符串转换分钟数加一.vi"("data[0]"=w370) -> ("日期/时间字符串"=w369:string)  [unwired: 10 in]
                                n260 = global write "全局 时间2.vi" "零点核查索引起始时间"(w369) -> ()
                              }
                            }
                          }
                          frame True {
                          }
                        }
                        n261 = Wait (ms)(milliseconds to wait=u32 500 ("等待时间（毫秒）")) -> ()  [unwired: 1 out]
                        n262 = global read "全局 数据数组大小.vi" "数据数组大小"() -> (w353:i32)
                        n263 = global read "全局 小时数据发送次数.vi" "小时数据发送次数"() -> (w357:i32)
                        n264 = Greater Or Equal?(x=w357, y=w353) -> (x >= y?=w356:bool)
                        n265 = Compound Arithmetic op=OR ("复合运算")(w356) -> (w355:bool)
                      }
                    }
                  }
                }
                frame "跨度核查" {
                  n266 = flat-sequence {
                    frame #0 {
                      n267 = global write "全局 小时数据发送次数.vi" "小时数据发送次数"(0 ("小时数据发送次数")) -> ()
                      n268 = global write "全局 实时数据参数.vi" "实时数据参数"("跨度核查") -> ()
                      n269 = global write "全局1.vi" "枚举"(enum16{"返回请求应答", "上传数据", "返回执行结果"}."上传数据" ("枚举")) -> ()
                    }
                    frame #1 {
                      n270 = call "从数据库获取数据通用可配置(子VI).vi"("table输入"="实时数据" ("新元素/子数组"), "列队名（唯一）"="c") -> ()  [unwired: 8 in, 2 out]
                    }
                    frame #2 {
                      n271 = call "数据处理整合 (子VI).vi"("枚举"=enum16{"实时数据排序", "小时数据排序"}."实时数据排序") -> ("已排序的数组"=w386:string[])  [unwired: 10 in]
                      n272 = Array Size(array=w386) -> (size(s)=w385:i32)
                      n273 = global write "全局 数据数组大小.vi" "数据数组大小"(w385) -> ()
                    }
                    frame #3 {
                      n274 = while {
                        stop <- w389 stop-if-true
                        n275 = property on="TCP服务端掉线计数" class="DigNum (严格)"() -> ("Value"=w393:i32)  [unwired: 2 in, 2 out]
                        n276 = property on="TCP服务端掉线计数" class="DigNum (严格)" props=["Value"]() -> ()  [unwired: 2 in, 3 out]
                        n277 = Greater Or Equal?(x=w393, y=1) -> (x >= y?=w392:bool)
                        n278 = case shown="假" w392 {
                          frame False {
                            n279 = global read "全局 数据数组大小.vi" "数据数组大小"() -> (w396:i32)
                            n280 = Greater Than 0?(x=w396) -> (x > 0?=w395:bool)
                            n281 = case shown="真" w395 {
                              frame False {
                              }
                              frame True {
                                n282 = global read "插值后的新数组.vi" "插值后的数组元素"() -> (w409:T10)
                                n283 = global read "全局 数据数组大小.vi" "数据数组大小"() -> (w406:i32)
                                n284 = local read "QN"() -> (w412:string)
                                n285 = local read "MN"() -> (w402:string)
                                n286 = local read "PW"() -> (w401:string)
                                n287 = local read "数据发送通道"() -> (w400:enum16{"TCP", "VISA"})
                                n288 = Decrement(x=w406) -> (x-1=w405:i32)
                                n289 = Unbundle By Name(w409) -> ("氨氮"=w408:string[][])
                                n290 = call "数据编码.vi"("table输入"="实时数据" ("新元素/子数组"), "QN"=w412, "MN"=w402, "PW"=w401) -> ("通讯包字符串"=w398:string)  [unwired: 10 in, 1 out]
                                n291 = local write "发送报文显示"(w398) -> ()
                                n292 = Index Array(array=w408, index (row)=w405, index (col)=0 ("禁用的索引 (列)")) -> (element=w404:string)
                                n293 = call "VISATCP组合选择发送.vi"("数据发送通道"=w400, "命令"="write", "写入缓冲区"=w398) -> ("错误输出"=w397:errorcluster)  [unwired: 9 in, 3 out]
                                n294 = Build Array(w398) -> (w411:string[])
                                n295 = local write "核查数据上传"(TRUE ("数据上传")) -> ()
                                n296 = call "日期时间字符串转换分钟数加一.vi"("data[0]"=w404) -> ("日期/时间字符串"=w403:string)  [unwired: 10 in]
                                n297 = local write "错误输出"(w397) -> ()
                                n298 = call "发送数据记录到文档(子VI).vi"("数组"=w411) -> ()  [unwired: 9 in, 1 out]
                                n299 = global write "全局 时间2.vi" "跨度核查索引起始时间"(w403) -> ()
                              }
                            }
                          }
                          frame True {
                          }
                        }
                        n300 = Wait (ms)(milliseconds to wait=u32 500 ("等待时间（毫秒）")) -> ()  [unwired: 1 out]
                        n301 = global read "全局 数据数组大小.vi" "数据数组大小"() -> (w387:i32)
                        n302 = global read "全局 小时数据发送次数.vi" "小时数据发送次数"() -> (w391:i32)
                        n303 = Greater Or Equal?(x=w391, y=w387) -> (x >= y?=w390:bool)
                        n304 = Compound Arithmetic op=OR ("复合运算")(w390) -> (w389:bool)
                      }
                    }
                  }
                }
                frame "标样核查" {
                  n305 = flat-sequence {
                    tunnel: [w423] -> w414
                    frame #0 {
                      n306 = global write "全局 小时数据发送次数.vi" "小时数据发送次数"(0 ("小时数据发送次数")) -> ()
                      n307 = global write "全局 实时数据参数.vi" "实时数据参数"("核查数据") -> ()
                      n308 = global write "全局1.vi" "枚举"(enum16{"返回请求应答", "上传数据", "返回执行结果"}."上传数据" ("枚举")) -> ()
                    }
                    frame #1 {
                      n309 = call "从数据库获取数据通用可配置(子VI).vi"("table输入"="实时数据" ("新元素/子数组"), "列队名（唯一）"="n") -> ()  [unwired: 8 in, 2 out]
                    }
                    frame #2 {
                      n310 = call "数据处理整合 (子VI).vi"("枚举"=enum16{"实时数据排序", "小时数据排序"}."实时数据排序") -> ("已排序的数组"=w422:string[])  [unwired: 10 in]
                      n311 = Array Size(array=w422) -> (size(s)=w421:i32)
                      n312 = global write "全局 数据数组大小.vi" "数据数组大小"(w421) -> ()
                    }
                    frame #3 {
                      n313 = while {
                        tunnel: [w424] -> w423
                        stop <- w424 stop-if-true
                        n314 = property on="TCP服务端掉线计数" class="DigNum (严格)"() -> ("Value"=w430:i32)  [unwired: 2 in, 2 out]
                        n315 = property on="TCP服务端掉线计数" class="DigNum (严格)" props=["Value"]() -> ()  [unwired: 2 in, 3 out]
                        n316 = Greater Or Equal?(x=w430, y=1) -> (x >= y?=w429:bool)
                        n317 = case shown="假" w429 {
                          frame False {
                            n318 = global read "全局 数据数组大小.vi" "数据数组大小"() -> (w433:i32)
                            n319 = Greater Than 0?(x=w433) -> (x > 0?=w432:bool)
                            n320 = case shown="真" w432 {
                              frame False {
                              }
                              frame True {
                                n321 = global read "插值后的新数组.vi" "插值后的数组元素"() -> (w446:T10)
                                n322 = global read "全局 数据数组大小.vi" "数据数组大小"() -> (w443:i32)
                                n323 = local read "QN"() -> (w449:string)
                                n324 = local read "MN"() -> (w439:string)
                                n325 = local read "PW"() -> (w438:string)
                                n326 = local read "数据发送通道"() -> (w437:enum16{"TCP", "VISA"})
                                n327 = Decrement(x=w443) -> (x-1=w442:i32)
                                n328 = Unbundle By Name(w446) -> ("氨氮"=w445:string[][])
                                n329 = call "数据编码.vi"("table输入"="实时数据" ("新元素/子数组"), "QN"=w449, "MN"=w439, "PW"=w438) -> ("通讯包字符串"=w435:string)  [unwired: 10 in, 1 out]
                                n330 = local write "发送报文显示"(w435) -> ()
                                n331 = call "VISATCP组合选择发送.vi"("数据发送通道"=w437, "命令"="write", "写入缓冲区"=w435) -> ("错误输出"=w434:errorcluster)  [unwired: 9 in, 3 out]
                                n332 = Index Array(array=w445, index (row)=w442, index (col)=0 ("禁用的索引 (列)")) -> (element=w441:string)
                                n333 = Build Array(w435) -> (w448:string[])
                                n334 = local write "核查数据上传"(TRUE ("数据上传")) -> ()
                                n335 = call "日期时间字符串转换分钟数加一.vi"("data[0]"=w441) -> ("日期/时间字符串"=w440:string)  [unwired: 10 in]
                                n336 = local write "错误输出"(w434) -> ()
                                n337 = call "发送数据记录到文档(子VI).vi"("数组"=w448) -> ()  [unwired: 9 in, 1 out]
                                n338 = global write "全局 时间2.vi" "标样核查索引起始时间"(w440) -> ()
                              }
                            }
                          }
                          frame True {
                          }
                        }
                        n339 = Wait (ms)(milliseconds to wait=u32 500 ("等待时间（毫秒）")) -> ()  [unwired: 1 out]
                        n340 = global read "全局 数据数组大小.vi" "数据数组大小"() -> (w425:i32)
                        n341 = global read "全局 小时数据发送次数.vi" "小时数据发送次数"() -> (w428:i32)
                        n342 = Greater Or Equal?(x=w428, y=w425) -> (x >= y?=w427:bool)
                        n343 = Compound Arithmetic op=OR ("复合运算")(w427) -> (w424:bool)
                      }
                    }
                  }
                }
                frame "加标回收" {
                  n344 = flat-sequence {
                    frame #0 {
                      n345 = global write "全局 小时数据发送次数.vi" "小时数据发送次数"(0 ("小时数据发送次数")) -> ()
                      n346 = global write "全局 实时数据参数.vi" "实时数据参数"("加标回收测试") -> ()
                      n347 = global write "全局1.vi" "枚举"(enum16{"返回请求应答", "上传数据", "返回执行结果"}."上传数据" ("枚举")) -> ()
                    }
                    frame #1 {
                      n348 = call "从数据库获取数据通用可配置(子VI).vi"("table输入"="加标回收" ("新元素/子数组"), "列队名（唯一）"="d") -> ()  [unwired: 8 in, 2 out]
                    }
                    frame #2 {
                      n349 = call "加标回收数据处理整合 (子VI).vi"("枚举"=enum16{"实时数据排序", "小时数据排序"}."实时数据排序") -> ("已排序的数组"=w457:string[])  [unwired: 10 in]
                      n350 = Array Size(array=w457) -> (size(s)=w458:i32)
                      n351 = global write "全局 数据数组大小.vi" "数据数组大小"(w458) -> ()
                    }
                    frame #3 {
                      n352 = while {
                        stop <- w461 stop-if-true
                        n353 = property on="TCP服务端掉线计数" class="DigNum (严格)"() -> ("Value"=w466:i32)  [unwired: 2 in, 2 out]
                        n354 = Greater Or Equal?(x=w466, y=1) -> (x >= y?=w464:bool)
                        n355 = case shown="假" w464 {
                          frame False {
                            n356 = global read "全局 数据数组大小.vi" "数据数组大小"() -> (w468:i32)
                            n357 = Greater Than 0?(x=w468) -> (x > 0?=w467:bool)
                            n358 = case shown="真" w467 {
                              frame False {
                              }
                              frame True {
                                n359 = global read "全局 数据数组大小.vi" "数据数组大小"() -> (w478:i32)
                                n360 = global read "插值后的新数组.vi" "插值后的数组元素"() -> (w481:T10)
                                n361 = local read "MN"() -> (w474:string)
                                n362 = local read "PW"() -> (w473:string)
                                n363 = local read "数据发送通道"() -> (w472:enum16{"TCP", "VISA"})
                                n364 = Decrement(x=w478) -> (x-1=w477:i32)
                                n365 = call "数据编码.vi"("table输入"="实时数据" ("新元素/子数组"), "MN"=w474, "PW"=w473) -> ("通讯包字符串"=w470:string)  [unwired: 11 in, 1 out]
                                n366 = Unbundle By Name(w481) -> ("氨氮"=w480:string[][])
                                n367 = local write "发送报文显示"(w470) -> ()
                                n368 = call "VISATCP组合选择发送.vi"("数据发送通道"=w472, "命令"="write", "写入缓冲区"=w470) -> ("错误输出"=w469:errorcluster)  [unwired: 9 in, 3 out]
                                n369 = Index Array(array=w480, index (row)=w477, index (col)=0 ("禁用的索引 (列)")) -> (element=w476:string)
                                n370 = local write "核查数据上传"(TRUE ("数据上传")) -> ()
                                n371 = Build Array(w470) -> (w483:string[])
                                n372 = call "日期时间字符串转换分钟数加一.vi"("data[0]"=w476) -> ("日期/时间字符串"=w475:string)  [unwired: 10 in]
                                n373 = local write "错误输出"(w469) -> ()
                                n374 = call "发送数据记录到文档(子VI).vi"("数组"=w483) -> ()  [unwired: 9 in, 1 out]
                                n375 = global write "全局 时间2.vi" "加标回收索引起始时间"(w475) -> ()
                              }
                            }
                          }
                          frame True {
                          }
                        }
                        n376 = Wait (ms)(milliseconds to wait=u32 500 ("等待时间（毫秒）")) -> ()  [unwired: 1 out]
                        n377 = global read "全局 数据数组大小.vi" "数据数组大小"() -> (w459:i32)
                        n378 = global read "全局 小时数据发送次数.vi" "小时数据发送次数"() -> (w463:i32)
                        n379 = Greater Or Equal?(x=w463, y=w459) -> (x >= y?=w462:bool)
                        n380 = Compound Arithmetic op=OR ("复合运算")(w462) -> (w461:bool)
                      }
                    }
                  }
                }
                frame "平行样" {
                  n381 = flat-sequence {
                    frame #0 {
                      n382 = global write "全局 小时数据发送次数.vi" "小时数据发送次数"(0 ("小时数据发送次数")) -> ()
                      n383 = global write "全局 实时数据参数.vi" "实时数据参数"("平行样测试") -> ()
                      n384 = global write "全局1.vi" "枚举"(enum16{"返回请求应答", "上传数据", "返回执行结果"}."上传数据" ("枚举")) -> ()
                    }
                    frame #1 {
                      n385 = call "从数据库获取数据通用可配置(子VI).vi"("table输入"="实时数据" ("新元素/子数组"), "列队名（唯一）"="e") -> ()  [unwired: 8 in, 2 out]
                    }
                    frame #2 {
                      n386 = call "数据处理整合 (子VI).vi"("枚举"=enum16{"实时数据排序", "小时数据排序"}."实时数据排序") -> ("已排序的数组"=w492:string[])  [unwired: 10 in]
                      n387 = Array Size(array=w492) -> (size(s)=w491:i32)
                      n388 = global write "全局 数据数组大小.vi" "数据数组大小"(w491) -> ()
                    }
                    frame #3 {
                      n389 = while {
                        stop <- w495 stop-if-true
                        n390 = property on="TCP服务端掉线计数" class="DigNum (严格)"() -> ("Value"=w501:i32)  [unwired: 2 in, 2 out]
                        n391 = property on="TCP服务端掉线计数" class="DigNum (严格)" props=["Value"]() -> ()  [unwired: 2 in, 3 out]
                        n392 = Greater Or Equal?(x=w501, y=1) -> (x >= y?=w499:bool)
                        n393 = case shown="假" w499 {
                          frame False {
                            n394 = global read "全局 数据数组大小.vi" "数据数组大小"() -> (w503:i32)
                            n395 = Greater Than 0?(x=w503) -> (x > 0?=w502:bool)
                            n396 = case shown="真" w502 {
                              frame False {
                              }
                              frame True {
                                n397 = local read "MN"() -> (w509:string)
                                n398 = local read "PW"() -> (w508:string)
                                n399 = local read "数据发送通道"() -> (w507:enum16{"TCP", "VISA"})
                                n400 = local write "核查数据上传"(TRUE ("数据上传")) -> ()
                                n401 = call "数据编码.vi"("table输入"="实时数据" ("新元素/子数组"), "MN"=w509, "PW"=w508) -> ("通讯包字符串"=w505:string)  [unwired: 11 in, 1 out]
                                n402 = local write "发送报文显示"(w505) -> ()
                                n403 = call "VISATCP组合选择发送.vi"("数据发送通道"=w507, "命令"="write", "写入缓冲区"=w505) -> ("错误输出"=w504:errorcluster)  [unwired: 9 in, 3 out]
                                n404 = Build Array(w505) -> (w511:string[])
                                n405 = call "发送数据记录到文档(子VI).vi"("数组"=w511) -> ()  [unwired: 9 in, 1 out]
                                n406 = local write "错误输出"(w504) -> ()
                              }
                            }
                          }
                          frame True {
                          }
                        }
                        n407 = Wait (ms)(milliseconds to wait=u32 500 ("等待时间（毫秒）")) -> ()  [unwired: 1 out]
                        n408 = global read "全局 数据数组大小.vi" "数据数组大小"() -> (w498:i32)
                        n409 = global read "全局 小时数据发送次数.vi" "小时数据发送次数"() -> (w497:i32)
                        n410 = Decrement(x=w498) -> (x-1=w494:i32)
                        n411 = Greater Or Equal?(x=w497, y=w494) -> (x >= y?=w496:bool)
                        n412 = Compound Arithmetic op=OR ("复合运算")(w496) -> (w495:bool)
                      }
                    }
                  }
                }
                frame "", Default {
                  n413 = Get Queue Status(queue=w516) -> (# elements in queue=w515:i32)  [unwired: 2 in, 7 out]
                  n414 = Equal To 0?(x=w515) -> (x = 0?=w514:bool)
                  n415 = case shown="真" w514 {
                    tunnel: [_ TRUE] -> w513
                    frame False {
                    }
                    frame True {
                    }
                  }
                }
              }
              n416 = Wait (ms)(milliseconds to wait=u32 3000 ("等待时间（毫秒）")) -> ()  [unwired: 1 out]
            }
          }
          frame "小时数据" {
            # "间隔时间上传"
            n417 = flat-sequence {
              frame #0 {
                # "发送前2小时的数据"
                n418 = global write "全局 小时数据发送次数.vi" "小时数据发送次数"(1 ("小时数据发送次数")) -> ()
                n419 = global write "全局1.vi" "枚举"(enum16{"返回请求应答", "上传数据", "返回执行结果"}."上传数据" ("枚举")) -> ()
              }
              frame #1 {
                n420 = call "从数据库获取数据通用可配置(子VI).vi"("table输入"="小时数据" ("新元素/子数组"), "列队名（唯一）"="XS" ("名称（未命名）")) -> ()  [unwired: 8 in, 2 out]
              }
              frame #2 {
                n421 = property on="TCP服务端掉线计数" class="DigNum (严格)"() -> ("Value"=w523:i32)  [unwired: 2 in, 2 out]
                n422 = Greater Or Equal?(x=w523, y=1) -> (x >= y?=w522:bool)
                n423 = case shown="假" w522 {
                  frame False {
                    # "数据处理整合"
                    n424 = call "实时小时数据处理整合 (子VI).vi"("枚举"=enum16{"实时数据排序", "小时数据排序"}."小时数据排序") -> ("已排序的数组"=w525:string[])  [unwired: 10 in]
                    n425 = Array Size(array=w525) -> (size(s)=w528:i32)
                    n426 = global write "全局 数据数组大小.vi" "数据数组大小"(1 ("数据数组大小")) -> ()
                    n427 = Greater Than 0?(x=w528) -> (x > 0?=w529:bool)
                    n428 = case shown="真" w529 {
                      frame False {
                      }
                      frame True {
                        n429 = local write "核查数据上传"(TRUE ("数据上传")) -> ()
                        n430 = Get Date/Time In Seconds() -> (seconds since 1Jan1904=w540:timestamp)
                        n431 = Format Date/Time String(time format string (%c)="%Y%m%d%H%M%S%3u" ("时间格式字符串(%c)"), seconds (now)=w540) -> (date/time string=w541:string)  [unwired: 1 in]
                        n432 = local read "MN"() -> (w535:string)
                        n433 = local read "PW"() -> (w534:string)
                        n434 = Search and Replace String(input string=w541, search string="." ("搜索字符串")) -> (result string=w543:string)  [unwired: 6 in, 3 out]
                        n435 = local read "数据发送通道"() -> (w533:enum16{"TCP", "VISA"})
                        n436 = call "数据编码.vi"("table输入"="小时数据" ("新元素/子数组"), "QN"=w543, "MN"=w535, "PW"=w534) -> ("通讯包字符串"=w531:string)  [unwired: 10 in, 1 out]
                        n437 = local write "发送报文显示"(w531) -> ()
                        n438 = call "VISATCP组合选择发送.vi"("数据发送通道"=w533, "命令"="write", "写入缓冲区"=w531) -> ("错误输出"=w530:errorcluster)  [unwired: 9 in, 3 out]
                        n439 = Build Array(w531) -> (w537:string[])
                        n440 = local write "错误输出"(w530) -> ()
                        n441 = call "发送数据记录到文档(子VI).vi"("数组"=w537) -> ()  [unwired: 9 in, 1 out]
                      }
                    }
                  }
                  frame True {
                  }
                }
              }
            }
          }
          frame "操作日志" {
            # "间隔时间上传"
            # "直接1分钟查询 一次,有数据就按数据上传,没数据就不上传,在数据发送那边有做处理"
            n442 = flat-sequence {
              frame #0 {
                # "时间"
                n443 = global read "全局 数据发送重叠.vi" "数据发送重叠开始时间戳"() -> (w545:string)
                n444 = global read "全局 数据发送重叠.vi" "数据发送重叠"() -> (w544:bool)
                n445 = global write "全局 小时数据发送次数.vi" "小时数据发送次数"(0 ("小时数据发送次数")) -> ()
                n446 = global write "全局1.vi" "枚举"(enum16{"返回请求应答", "上传数据", "返回执行结果"}."上传数据" ("枚举")) -> ()
                n447 = call "日志信息主动发送(子VI).vi"("是否正在查询数据"=w544, "查询数据发送时间节点"=w545) -> ()  [unwired: 10 in]
              }
              frame #1 {
                n448 = call "获取操作日志 (子VI).vi"("table输入"="操作日志") -> ()  [unwired: 11 in]
              }
              frame #2 {
                n449 = call "数据处理整合 (子VI).vi"("枚举"=enum16{"实时数据排序", "小时数据排序"}."实时数据排序") -> ("已排序的数组"=w551:string[])  [unwired: 10 in]
                n450 = Array Size(array=w551) -> (size(s)=w550:i32)
                n451 = global write "全局 数据数组大小.vi" "数据数组大小"(w550) -> ()
              }
              frame #3 {
                n452 = while {
                  stop <- w552 stop-if-true
                  # "判定是否存表"
                  n453 = property on="TCP服务端掉线计数" class="DigNum (严格)"() -> ("Value"=w558:i32)  [unwired: 2 in, 2 out]
                  n454 = Greater Or Equal?(x=w558, y=1) -> (x >= y?=w557:bool)
                  n455 = case shown="假" w557 {
                    frame False {
                      n456 = global read "全局 数据数组大小.vi" "数据数组大小"() -> (w560:i32)
                      n457 = Greater Than 0?(x=w560) -> (x > 0?=w561:bool)
                      n458 = case shown="真" w561 {
                        frame False {
                        }
                        frame True {
                          n459 = global read "全局 小时数据发送次数.vi" "小时数据发送次数"() -> (w570:i32)
                          n460 = local write "核查数据上传"(TRUE ("数据上传")) -> ()
                          n461 = Get Date/Time In Seconds() -> (seconds since 1Jan1904=w575:timestamp)
                          n462 = Increment(x=w570) -> (x+1=w569:i32)
                          n463 = Format Date/Time String(time format string (%c)="%Y%m%d%H%M%S%3u" ("时间格式字符串(%c)"), seconds (now)=w575) -> (date/time string=w574:string)  [unwired: 1 in]
                          n464 = global write "全局 小时数据发送次数.vi" "小时数据发送次数"(w569) -> ()
                          n465 = Search and Replace String(input string=w574, search string="." ("搜索字符串")) -> (result string=w572:string)  [unwired: 6 in, 3 out]
                          n466 = local read "MN"() -> (w567:string)
                          n467 = local read "PW"() -> (w566:string)
                          n468 = call "数据编码.vi"("table输入"="操作日志" ("新元素/子数组"), "QN"=w572, "MN"=w567, "PW"=w566) -> ("通讯包字符串"=w563:string)  [unwired: 10 in, 1 out]
                          n469 = local read "数据发送通道"() -> (w565:enum16{"TCP", "VISA"})
                          n470 = local write "发送报文显示"(w563) -> ()
                          n471 = call "VISATCP组合选择发送.vi"("数据发送通道"=w565, "命令"="write", "写入缓冲区"=w563) -> ("错误输出"=w562:errorcluster)  [unwired: 9 in, 3 out]
                          n472 = Build Array(w563) -> (w571:string[])
                          n473 = local write "错误输出"(w562) -> ()
                          n474 = call "发送数据记录到文档(子VI).vi"("数组"=w571) -> ()  [unwired: 9 in, 1 out]
                        }
                      }
                    }
                    frame True {
                    }
                  }
                  n475 = Wait (ms)(milliseconds to wait=u32 500 ("等待时间（毫秒）")) -> ()  [unwired: 1 out]
                  n476 = global read "全局 数据数组大小.vi" "数据数组大小"() -> (w554:i32)
                  n477 = global read "全局 小时数据发送次数.vi" "小时数据发送次数"() -> (w556:i32)
                  n478 = Decrement(x=w554) -> (x-1=w553:i32)
                  n479 = Greater Or Equal?(x=w556, y=w553) -> (x >= y?=w552:bool)
                }
              }
            }
          }
          frame "仪器参数" {
            # "间隔时间上传"
            # "直接1分钟查询 一次,有数据就按数据上传,没数据就不上传,在数据发送那边有做处理"
            n480 = flat-sequence {
              frame #0 {
                # "时间"
                n481 = global read "全局 数据发送重叠.vi" "数据发送重叠开始时间戳"() -> (w579:string)
                n482 = global read "全局 数据发送重叠.vi" "数据发送重叠"() -> (w578:bool)
                n483 = global write "全局 小时数据发送次数.vi" "小时数据发送次数"(0 ("小时数据发送次数")) -> ()
                n484 = global write "全局1.vi" "枚举"(enum16{"返回请求应答", "上传数据", "返回执行结果"}."上传数据" ("枚举")) -> ()
                n485 = call "日志信息主动发送(子VI).vi"("是否正在查询数据"=w578, "查询数据发送时间节点"=w579) -> ()  [unwired: 10 in]
              }
              frame #1 {
                n486 = call "获取操作日志 (子VI).vi"("table输入"="仪器参数") -> ()  [unwired: 11 in]
              }
              frame #2 {
                n487 = call "数据处理整合 (子VI).vi"("枚举"=enum16{"实时数据排序", "小时数据排序"}."实时数据排序") -> ("已排序的数组"=w585:string[])  [unwired: 10 in]
                n488 = Array Size(array=w585) -> (size(s)=w584:i32)
                n489 = global write "全局 数据数组大小.vi" "数据数组大小"(w584) -> ()
              }
              frame #3 {
                n490 = while {
                  stop <- w586 stop-if-true
                  # "判定是否存表"
                  n491 = property on="TCP服务端掉线计数" class="DigNum (严格)"() -> ("Value"=w592:i32)  [unwired: 2 in, 2 out]
                  n492 = Greater Or Equal?(x=w592, y=1) -> (x >= y?=w591:bool)
                  n493 = case shown="假" w591 {
                    frame False {
                      n494 = global read "全局 数据数组大小.vi" "数据数组大小"() -> (w594:i32)
                      n495 = Greater Than 0?(x=w594) -> (x > 0?=w595:bool)
                      n496 = case shown="真" w595 {
                        frame False {
                        }
                        frame True {
                          n497 = global read "全局 小时数据发送次数.vi" "小时数据发送次数"() -> (w604:i32)
                          n498 = local write "核查数据上传"(TRUE ("数据上传")) -> ()
                          n499 = Get Date/Time In Seconds() -> (seconds since 1Jan1904=w609:timestamp)
                          n500 = Increment(x=w604) -> (x+1=w603:i32)
                          n501 = Format Date/Time String(time format string (%c)="%Y%m%d%H%M%S%3u" ("时间格式字符串(%c)"), seconds (now)=w609) -> (date/time string=w608:string)  [unwired: 1 in]
                          n502 = global write "全局 小时数据发送次数.vi" "小时数据发送次数"(w603) -> ()
                          n503 = Search and Replace String(input string=w608, search string="." ("搜索字符串")) -> (result string=w606:string)  [unwired: 6 in, 3 out]
                          n504 = local read "MN"() -> (w601:string)
                          n505 = local read "PW"() -> (w600:string)
                          n506 = call "数据编码.vi"("table输入"="仪器参数" ("新元素/子数组"), "QN"=w606, "MN"=w601, "PW"=w600) -> ("通讯包字符串"=w597:string)  [unwired: 10 in, 1 out]
                          n507 = local read "数据发送通道"() -> (w599:enum16{"TCP", "VISA"})
                          n508 = local write "发送报文显示"(w597) -> ()
                          n509 = call "VISATCP组合选择发送.vi"("数据发送通道"=w599, "命令"="write", "写入缓冲区"=w597) -> ("错误输出"=w596:errorcluster)  [unwired: 9 in, 3 out]
                          n510 = Build Array(w597) -> (w605:string[])
                          n511 = local write "错误输出"(w596) -> ()
                          n512 = call "发送数据记录到文档(子VI).vi"("数组"=w605) -> ()  [unwired: 9 in, 1 out]
                        }
                      }
                    }
                    frame True {
                    }
                  }
                  n513 = Wait (ms)(milliseconds to wait=u32 500 ("等待时间（毫秒）")) -> ()  [unwired: 1 out]
                  n514 = global read "全局 数据数组大小.vi" "数据数组大小"() -> (w588:i32)
                  n515 = global read "全局 小时数据发送次数.vi" "小时数据发送次数"() -> (w590:i32)
                  n516 = Decrement(x=w588) -> (x-1=w587:i32)
                  n517 = Greater Or Equal?(x=w590, y=w587) -> (x >= y?=w586:bool)
                }
              }
            }
          }
          frame "系统状态" {
            # "直接1分钟查询 一次,有变化就按上传,没变化就不上传"
            n518 = flat-sequence {
              frame #0 {
                # "时间"
                n519 = global write "全局 小时数据发送次数.vi" "小时数据发送次数"(0 ("小时数据发送次数")) -> ()
                n520 = global write "全局 数据数组大小.vi" "数据数组大小"(1 ("数据数组大小")) -> ()
                n521 = global write "全局1.vi" "枚举"(enum16{"返回请求应答", "上传数据", "返回执行结果"}."上传数据" ("枚举")) -> ()
              }
              frame #1 {
                # "判定是否存表"
                n522 = property on="TCP服务端掉线计数" class="DigNum (严格)"() -> ("Value"=w616:i32)  [unwired: 2 in, 2 out]
                n523 = Greater Or Equal?(x=w616, y=1) -> (x >= y?=w615:bool)
                n524 = case shown="假" w615 {
                  frame False {
                    n525 = global read "全局 数据数组大小.vi" "数据数组大小"() -> (w618:i32)
                    n526 = Greater Than 0?(x=w618) -> (x > 0?=w619:bool)
                    n527 = case shown="真" w619 {
                      frame False {
                      }
                      frame True {
                        n528 = global read "全局 小时数据发送次数.vi" "小时数据发送次数"() -> (w628:i32)
                        n529 = local write "核查数据上传"(TRUE ("数据上传")) -> ()
                        n530 = Get Date/Time In Seconds() -> (seconds since 1Jan1904=w633:timestamp)
                        n531 = Increment(x=w628) -> (x+1=w627:i32)
                        n532 = Format Date/Time String(time format string (%c)="%Y%m%d%H%M%S%3u" ("时间格式字符串(%c)"), seconds (now)=w633) -> (date/time string=w632:string)  [unwired: 1 in]
                        n533 = global write "全局 小时数据发送次数.vi" "小时数据发送次数"(w627) -> ()
                        n534 = Search and Replace String(input string=w632, search string="." ("搜索字符串")) -> (result string=w630:string)  [unwired: 6 in, 3 out]
                        n535 = local read "MN"() -> (w625:string)
                        n536 = local read "PW"() -> (w624:string)
                        n537 = call "数据编码.vi"("table输入"="系统状态" ("新元素/子数组"), "QN"=w630, "MN"=w625, "PW"=w624) -> ("通讯包字符串"=w621:string)  [unwired: 10 in, 1 out]
                        n538 = local read "数据发送通道"() -> (w623:enum16{"TCP", "VISA"})
                        n539 = local write "发送报文显示"(w621) -> ()
                        n540 = call "VISATCP组合选择发送.vi"("数据发送通道"=w623, "命令"="write", "写入缓冲区"=w621) -> ("错误输出"=w620:errorcluster)  [unwired: 9 in, 3 out]
                        n541 = Build Array(w621) -> (w629:string[])
                        n542 = local write "错误输出"(w620) -> ()
                        n543 = call "发送数据记录到文档(子VI).vi"("数组"=w629) -> ()  [unwired: 9 in, 1 out]
                      }
                    }
                  }
                  frame True {
                  }
                }
              }
            }
          }
          frame "运行模式" {
            # "直接1分钟查询 一次,有变化就按上传,没变化就不上传"
            n544 = flat-sequence {
              frame #0 {
                # "时间"
                n545 = global write "全局 小时数据发送次数.vi" "小时数据发送次数"(0 ("小时数据发送次数")) -> ()
                n546 = global write "全局 数据数组大小.vi" "数据数组大小"(1 ("数据数组大小")) -> ()
                n547 = global write "全局1.vi" "枚举"(enum16{"返回请求应答", "上传数据", "返回执行结果"}."上传数据" ("枚举")) -> ()
              }
              frame #1 {
                # "判定是否存表"
                n548 = property on="TCP服务端掉线计数" class="DigNum (严格)"() -> ("Value"=w640:i32)  [unwired: 2 in, 2 out]
                n549 = Greater Or Equal?(x=w640, y=1) -> (x >= y?=w639:bool)
                n550 = case shown="假" w639 {
                  frame False {
                    n551 = global read "全局 数据数组大小.vi" "数据数组大小"() -> (w642:i32)
                    n552 = Greater Than 0?(x=w642) -> (x > 0?=w643:bool)
                    n553 = case shown="真" w643 {
                      frame False {
                      }
                      frame True {
                        n554 = global read "全局 小时数据发送次数.vi" "小时数据发送次数"() -> (w652:i32)
                        n555 = local write "核查数据上传"(TRUE ("数据上传")) -> ()
                        n556 = Get Date/Time In Seconds() -> (seconds since 1Jan1904=w657:timestamp)
                        n557 = Increment(x=w652) -> (x+1=w651:i32)
                        n558 = Format Date/Time String(time format string (%c)="%Y%m%d%H%M%S%3u" ("时间格式字符串(%c)"), seconds (now)=w657) -> (date/time string=w656:string)  [unwired: 1 in]
                        n559 = global write "全局 小时数据发送次数.vi" "小时数据发送次数"(w651) -> ()
                        n560 = Search and Replace String(input string=w656, search string="." ("搜索字符串")) -> (result string=w654:string)  [unwired: 6 in, 3 out]
                        n561 = local read "MN"() -> (w648:string)
                        n562 = local read "PW"() -> (w649:string)
                        n563 = local read "数据发送通道"() -> (w647:enum16{"TCP", "VISA"})
                        n564 = call "数据编码.vi"("table输入"="运行模式" ("新元素/子数组"), "QN"=w654, "MN"=w648, "PW"=w649) -> ("通讯包字符串"=w644:string)  [unwired: 10 in, 1 out]
                        n565 = local write "发送报文显示"(w644) -> ()
                        n566 = call "VISATCP组合选择发送.vi"("数据发送通道"=w647, "命令"="write", "写入缓冲区"=w644) -> ("错误输出"=w645:errorcluster)  [unwired: 9 in, 3 out]
                        n567 = Build Array(w644) -> (w653:string[])
                        n568 = local write "错误输出"(w645) -> ()
                        n569 = call "发送数据记录到文档(子VI).vi"("数组"=w653) -> ()  [unwired: 9 in, 1 out]
                      }
                    }
                  }
                  frame True {
                  }
                }
              }
            }
          }
          frame "测量周期" {
            # "直接1分钟查询 一次,有变化就按上传,没变化就不上传"
            n570 = flat-sequence {
              frame #0 {
                # "时间"
                n571 = global write "全局 小时数据发送次数.vi" "小时数据发送次数"(0 ("小时数据发送次数")) -> ()
                n572 = global write "全局 数据数组大小.vi" "数据数组大小"(1 ("数据数组大小")) -> ()
                n573 = global write "全局1.vi" "枚举"(enum16{"返回请求应答", "上传数据", "返回执行结果"}."上传数据" ("枚举")) -> ()
              }
              frame #1 {
                # "判定是否存表"
                n574 = property on="TCP服务端掉线计数" class="DigNum (严格)"() -> ("Value"=w664:i32)  [unwired: 2 in, 2 out]
                n575 = Greater Or Equal?(x=w664, y=1) -> (x >= y?=w663:bool)
                n576 = case shown="假" w663 {
                  frame False {
                    n577 = global read "全局 数据数组大小.vi" "数据数组大小"() -> (w666:i32)
                    n578 = Greater Than 0?(x=w666) -> (x > 0?=w667:bool)
                    n579 = case shown="真" w667 {
                      frame False {
                      }
                      frame True {
                        n580 = global read "全局 小时数据发送次数.vi" "小时数据发送次数"() -> (w676:i32)
                        n581 = local write "核查数据上传"(TRUE ("数据上传")) -> ()
                        n582 = Get Date/Time In Seconds() -> (seconds since 1Jan1904=w681:timestamp)
                        n583 = Increment(x=w676) -> (x+1=w675:i32)
                        n584 = Format Date/Time String(time format string (%c)="%Y%m%d%H%M%S%3u" ("时间格式字符串(%c)"), seconds (now)=w681) -> (date/time string=w680:string)  [unwired: 1 in]
                        n585 = global write "全局 小时数据发送次数.vi" "小时数据发送次数"(w675) -> ()
                        n586 = Search and Replace String(input string=w680, search string="." ("搜索字符串")) -> (result string=w678:string)  [unwired: 6 in, 3 out]
                        n587 = local read "MN"() -> (w673:string)
                        n588 = local read "PW"() -> (w672:string)
                        n589 = call "数据编码.vi"("table输入"="测量周期" ("新元素/子数组"), "QN"=w678, "MN"=w673, "PW"=w672) -> ("通讯包字符串"=w669:string)  [unwired: 10 in, 1 out]
                        n590 = local read "数据发送通道"() -> (w671:enum16{"TCP", "VISA"})
                        n591 = local write "发送报文显示"(w669) -> ()
                        n592 = call "VISATCP组合选择发送.vi"("数据发送通道"=w671, "命令"="write", "写入缓冲区"=w669) -> ("错误输出"=w668:errorcluster)  [unwired: 9 in, 3 out]
                        n593 = Build Array(w669) -> (w677:string[])
                        n594 = local write "错误输出"(w668) -> ()
                        n595 = call "发送数据记录到文档(子VI).vi"("数组"=w677) -> ()  [unwired: 9 in, 1 out]
                      }
                    }
                  }
                  frame True {
                  }
                }
              }
            }
          }
          frame "超标留样" {
            # "直接1分钟查询 一次,有变化就按上传,没变化就不上传"
            n596 = flat-sequence {
              frame #0 {
                # "时间"
                n597 = global write "全局 小时数据发送次数.vi" "小时数据发送次数"(0 ("小时数据发送次数")) -> ()
                n598 = global write "全局 数据数组大小.vi" "数据数组大小"(1 ("数据数组大小")) -> ()
                n599 = global write "全局1.vi" "枚举"(enum16{"返回请求应答", "上传数据", "返回执行结果"}."上传数据" ("枚举")) -> ()
              }
              frame #1 {
                # "判定是否存表"
                n600 = property on="TCP服务端掉线计数" class="DigNum (严格)"() -> ("Value"=w688:i32)  [unwired: 2 in, 2 out]
                n601 = Greater Or Equal?(x=w688, y=1) -> (x >= y?=w687:bool)
                n602 = case shown="假" w687 {
                  frame False {
                    n603 = global read "全局 数据数组大小.vi" "数据数组大小"() -> (w690:i32)
                    n604 = Greater Than 0?(x=w690) -> (x > 0?=w691:bool)
                    n605 = case shown="真" w691 {
                      frame False {
                      }
                      frame True {
                        n606 = global read "全局 小时数据发送次数.vi" "小时数据发送次数"() -> (w700:i32)
                        n607 = local write "核查数据上传"(TRUE ("数据上传")) -> ()
                        n608 = Get Date/Time In Seconds() -> (seconds since 1Jan1904=w705:timestamp)
                        n609 = Increment(x=w700) -> (x+1=w699:i32)
                        n610 = Format Date/Time String(time format string (%c)="%Y%m%d%H%M%S%3u" ("时间格式字符串(%c)"), seconds (now)=w705) -> (date/time string=w704:string)  [unwired: 1 in]
                        n611 = global write "全局 小时数据发送次数.vi" "小时数据发送次数"(w699) -> ()
                        n612 = Search and Replace String(input string=w704, search string="." ("搜索字符串")) -> (result string=w702:string)  [unwired: 6 in, 3 out]
                        n613 = local read "MN"() -> (w697:string)
                        n614 = local read "PW"() -> (w696:string)
                        n615 = call "数据编码.vi"("table输入"="超标留样" ("新元素/子数组"), "QN"=w702, "MN"=w697, "PW"=w696) -> ("通讯包字符串"=w693:string)  [unwired: 10 in, 1 out]
                        n616 = local read "数据发送通道"() -> (w695:enum16{"TCP", "VISA"})
                        n617 = local write "发送报文显示"(w693) -> ()
                        n618 = call "VISATCP组合选择发送.vi"("数据发送通道"=w695, "命令"="write", "写入缓冲区"=w693) -> ("错误输出"=w692:errorcluster)  [unwired: 9 in, 3 out]
                        n619 = Build Array(w693) -> (w701:string[])
                        n620 = local write "错误输出"(w692) -> ()
                        n621 = call "发送数据记录到文档(子VI).vi"("数组"=w701) -> ()  [unwired: 9 in, 1 out]
                      }
                    }
                  }
                  frame True {
                  }
                }
              }
            }
          }
          frame "报警信息" {
            # "间隔时间上传"
            # "直接1分钟查询 一次,有数据就按数据上传,没数据为空的不传,在数据发送那边有做处理"
            n622 = flat-sequence {
              frame #0 {
                # "分钟时间间隔"
                n623 = global read "全局 数据发送重叠.vi" "数据发送重叠开始时间戳"() -> (w709:string)
                n624 = global read "全局 数据发送重叠.vi" "数据发送重叠"() -> (w708:bool)
                n625 = global write "全局 小时数据发送次数.vi" "小时数据发送次数"(0 ("小时数据发送次数")) -> ()
                n626 = global write "全局1.vi" "枚举"(enum16{"返回请求应答", "上传数据", "返回执行结果"}."上传数据" ("枚举")) -> ()
                n627 = call "日志信息主动发送(子VI).vi"("是否正在查询数据"=w708, "查询数据发送时间节点"=w709) -> ()  [unwired: 10 in]
              }
              frame #1 {
                n628 = call "获取报警信息 (子VI).vi"() -> ()  [unwired: 12 in]
              }
              frame #2 {
                n629 = call "数据处理整合 (子VI).vi"("枚举"=enum16{"实时数据排序", "小时数据排序"}."实时数据排序") -> ("已排序的数组"=w714:string[])  [unwired: 10 in]
                n630 = Array Size(array=w714) -> (size(s)=w713:i32)
                n631 = global write "全局 数据数组大小.vi" "数据数组大小"(w713) -> ()
              }
              frame #3 {
                n632 = while {
                  stop <- w715 stop-if-true
                  # "判定是否存表"
                  n633 = property on="TCP服务端掉线计数" class="DigNum (严格)"() -> ("Value"=w721:i32)  [unwired: 2 in, 2 out]
                  n634 = Greater Or Equal?(x=w721, y=1) -> (x >= y?=w720:bool)
                  n635 = case shown="假" w720 {
                    frame False {
                      # "判定数据不为空才发"
                      n636 = global read "全局 数据数组大小.vi" "数据数组大小"() -> (w723:i32)
                      n637 = Greater Than 0?(x=w723) -> (x > 0?=w724:bool)
                      n638 = case shown="真" w724 {
                        frame False {
                          n639 = local write "核查数据上传"(FALSE ("数据上传")) -> ()
                        }
                        frame True {
                          n640 = global read "全局 小时数据发送次数.vi" "小时数据发送次数"() -> (w733:i32)
                          n641 = Get Date/Time In Seconds() -> (seconds since 1Jan1904=w738:timestamp)
                          n642 = Increment(x=w733) -> (x+1=w732:i32)
                          n643 = Format Date/Time String(time format string (%c)="%Y%m%d%H%M%S%3u" ("时间格式字符串(%c)"), seconds (now)=w738) -> (date/time string=w737:string)  [unwired: 1 in]
                          n644 = global write "全局 小时数据发送次数.vi" "小时数据发送次数"(w732) -> ()
                          n645 = Search and Replace String(input string=w737, search string="." ("搜索字符串")) -> (result string=w735:string)  [unwired: 6 in, 3 out]
                          n646 = local read "MN"() -> (w731:string)
                          n647 = local read "PW"() -> (w730:string)
                          n648 = local read "数据发送通道"() -> (w729:enum16{"TCP", "VISA"})
                          n649 = call "数据编码.vi"("table输入"="报警信息" ("新元素/子数组"), "QN"=w735, "MN"=w731, "PW"=w730) -> ("通讯包字符串"=w727:string)  [unwired: 10 in, 1 out]
                          n650 = local write "发送报文显示"(w727) -> ()
                          n651 = Build Array(w727) -> (w734:string[])
                          n652 = call "VISATCP组合选择发送.vi"("数据发送通道"=w729, "命令"="write", "写入缓冲区"=w727) -> ("错误输出"=w726:errorcluster)  [unwired: 9 in, 3 out]
                          n653 = local write "错误输出"(w726) -> ()
                          n654 = call "发送数据记录到文档(子VI).vi"("数组"=w734) -> ()  [unwired: 9 in, 1 out]
                        }
                      }
                    }
                    frame True {
                    }
                  }
                  n655 = Wait (ms)(milliseconds to wait=u32 500 ("等待时间（毫秒）")) -> ()  [unwired: 1 out]
                  n656 = global read "全局 数据数组大小.vi" "数据数组大小"() -> (w717:i32)
                  n657 = global read "全局 小时数据发送次数.vi" "小时数据发送次数"() -> (w719:i32)
                  n658 = Decrement(x=w717) -> (x-1=w716:i32)
                  n659 = Greater Or Equal?(x=w719, y=w716) -> (x >= y?=w715:bool)
                }
              }
            }
          }
          frame "环境参数" {
            # "间隔时间上传"
            # "直接1分钟查询 一次,有数据就按数据上传,没数据为空的不传,在数据发送那边有做处理"
            n660 = disable-structure shown="禁用" {
              frame Disabled {
                n661 = flat-sequence {
                  frame #0 {
                    # "分钟时间间隔"
                    n662 = global read "全局 数据发送重叠.vi" "数据发送重叠开始时间戳"() -> (w742:string)
                    n663 = global read "全局 数据发送重叠.vi" "数据发送重叠"() -> (w741:bool)
                    n664 = global write "全局 小时数据发送次数.vi" "小时数据发送次数"(0 ("小时数据发送次数")) -> ()
                    n665 = global write "全局1.vi" "枚举"(enum16{"返回请求应答", "上传数据", "返回执行结果"}."上传数据" ("枚举")) -> ()
                    n666 = call "日志信息主动发送(子VI).vi"("是否正在查询数据"=w741, "查询数据发送时间节点"=w742) -> ()  [unwired: 10 in]
                  }
                  frame #1 {
                    n667 = call "获取环境参数 (子VI).vi"() -> ()  [unwired: 12 in]
                  }
                  frame #2 {
                    n668 = call "数据处理整合 (子VI).vi"("枚举"=enum16{"实时数据排序", "小时数据排序"}."实时数据排序") -> ("已排序的数组"=w747:string[])  [unwired: 10 in]
                    n669 = Array Size(array=w747) -> (size(s)=w746:i32)
                    n670 = global write "全局 数据数组大小.vi" "数据数组大小"(w746) -> ()
                  }
                  frame #3 {
                    n671 = while {
                      stop <- w748 stop-if-true
                      # "判定是否存表"
                      n672 = property on="TCP服务端掉线计数" class="DigNum (严格)"() -> ("Value"=w754:i32)  [unwired: 2 in, 2 out]
                      n673 = Greater Or Equal?(x=w754, y=1) -> (x >= y?=w753:bool)
                      n674 = case shown="假" w753 {
                        frame False {
                          # "判定数据不为空才发"
                          n675 = global read "全局 数据数组大小.vi" "数据数组大小"() -> (w756:i32)
                          n676 = Greater Than 0?(x=w756) -> (x > 0?=w757:bool)
                          n677 = case shown="真" w757 {
                            frame False {
                            }
                            frame True {
                              n678 = global read "全局 小时数据发送次数.vi" "小时数据发送次数"() -> (w764:i32)
                              n679 = local write "核查数据上传"(TRUE ("数据上传")) -> ()
                              n680 = Get Date/Time In Seconds() -> (seconds since 1Jan1904=w769:timestamp)
                              n681 = Increment(x=w764) -> (x+1=w763:i32)
                              n682 = Format Date/Time String(time format string (%c)="%Y%m%d%H%M%S%3u" ("时间格式字符串(%c)"), seconds (now)=w769) -> (date/time string=w768:string)  [unwired: 1 in]
                              n683 = global write "全局 小时数据发送次数.vi" "小时数据发送次数"(w763) -> ()
                              n684 = Search and Replace String(input string=w768, search string="." ("搜索字符串")) -> (result string=w766:string)  [unwired: 6 in, 3 out]
                              n685 = local read "MN"() -> (w772:string)
                              n686 = local read "PW"() -> (w771:string)
                              n687 = local read "数据发送通道"() -> (w760:enum16{"TCP", "VISA"})
                              n688 = call "数据编码.vi"("table输入"="报警信息" ("新元素/子数组"), "QN"=w766, "MN"=w772, "PW"=w771) -> ("通讯包字符串"=w759:string)  [unwired: 10 in, 1 out]
                              n689 = local write "发送报文显示"(w759) -> ()
                              n690 = call "VISATCP组合选择发送.vi"("数据发送通道"=w760, "命令"="write", "写入缓冲区"=w759) -> ("错误输出"=w758:errorcluster)  [unwired: 9 in, 3 out]
                              n691 = Build Array(w759) -> (w765:string[])
                              n692 = local write "错误输出"(w758) -> ()
                              n693 = call "发送数据记录到文档(子VI).vi"("数组"=w765) -> ()  [unwired: 9 in, 1 out]
                            }
                          }
                        }
                        frame True {
                        }
                      }
                      n694 = Wait (ms)(milliseconds to wait=u32 500 ("等待时间（毫秒）")) -> ()  [unwired: 1 out]
                      n695 = global read "全局 数据数组大小.vi" "数据数组大小"() -> (w750:i32)
                      n696 = global read "全局 小时数据发送次数.vi" "小时数据发送次数"() -> (w752:i32)
                      n697 = Decrement(x=w750) -> (x-1=w749:i32)
                      n698 = Greater Or Equal?(x=w752, y=w749) -> (x >= y?=w748:bool)
                    }
                  }
                }
              }
              frame Enabled {
              }
            }
          }
        }
      }
    }
  }
  n699 = while "While循环" {
    tunnel: [w790] -> _
    tunnel: w32 -> [w784]
    stop <- FALSE stop-if-true
    w774 = FALSE ("小时数据上传")
    # "实时、小时数据出数据就上传"
    n700 = property on="TCP服务端掉线计数" class="DigNum (严格)"() -> ("Value"=w787:i32)  [unwired: 2 in, 2 out]
    n701 = local read "查询数据发送"() -> (w779:bool)
    n702 = local read "核查数据上传"() -> (w778:bool)
    n703 = local read "重发数据"() -> (w780:bool)
    n704 = local read "步骤"() -> (w789:T6)
    n705 = local write "实时小时数据上传"(w774) -> ()
    n706 = global write "全局 数据发送重叠.vi" "主动上报数据中"(w774) -> ()
    n707 = Greater Or Equal?(x=w784, y=17) -> (x >= y?=w783:bool)
    n708 = Equal To 0?(x=w787) -> (x = 0?=w785:bool)
    n709 = Not(x=w780) -> (.not. x?=w777:bool)
    n710 = Not(x=w779) -> (.not. x?=w776:bool)
    n711 = Not(x=w778) -> (.not. x?=w775:bool)
    n712 = Equal?(x=w789, y=T6."读取数据" ("步骤")) -> (x = y?=w786:bool)
    n713 = Wait (ms)(milliseconds to wait=u32 75430 ("等待时间（毫秒）")) -> ()  [unwired: 1 out]
    n714 = Compound Arithmetic op=AND ("复合运算")(w786, w785, w783, w777, w776, w775) -> (w781:bool)
    n715 = case shown="真" w781 {
      tunnel: [_ w795] -> w790
      frame False {
        w793 = FALSE ("小时数据上传")
        n716 = local write "实时小时数据上传"(w793) -> ()
        n717 = global write "全局 数据发送重叠.vi" "主动上报数据中"(w793) -> ()
      }
      frame True {
        n718 = flat-sequence {
          tunnel: [w804] -> w794
          tunnel: [w1179] -> w795
          tunnel: w794 -> [w1179]
          frame #0 {
            w796 = TRUE ("小时数据上传")
            n719 = disable-structure shown="启用" {
              frame Disabled {
                n720 = call "读取-删除文件.vi"() -> ("error out"=w797:errorcluster, "文本"=w798:string[])  [unwired: 10 in]
                n721 = for {
                  tunnel: w798 -> [w801] mode=indexing
                  tunnel: [w800] -> _ mode=indexing
                  tunnel: w797 -> [w799]
                  n722 = local read item#-1() -> (w802)
                  n723 = call "数据补发判定有限循环.vi"("错误输入（无错误）"=w799, "数据输入"=w801, 10:w802) -> ("error out"=w800:errorcluster)  [unwired: 8 in]
                }
              }
              frame Enabled {
              }
            }
            n724 = global write "全局 数据发送重叠.vi" "主动上报数据中"(w796) -> ()
            "实时小时数据上传" <- w796
          }
          frame #1 {
            n725 = local read "数据发送协议"() -> (w803:enum16{"2005-212协议", "2017-212协议"})
            n726 = case shown="\"2017-212协议\", 默认" w803 {
              tunnel: [_ w940] -> w804
              frame "2005-212协议" {
                n727 = local read "参数数值"() -> (w808:T5)
                n728 = Cluster To Array(cluster=w808) -> (array=w807:bool[])
                n729 = for {
                  tunnel: w807 -> [_] mode=indexing
                  tunnel: [w852] -> w806
                  i -> [w846]
                  w847 = "1904/01/01 00:00:00"
                  (unwired) " where 时间 between #"
                  w850 = "database1.mdb" ("database")
                  (unwired) "'and 数据类型 ='N' and 时间 between "
                  w854 = 0 ("索引 (行)")
                  n730 = case shown="12" w846 {
                    tunnel: [w904 w906 w908 w910 w912 w914 w916 w918 w920 w922 w924 w926 w928 w930 w932 w934 w936 w938] -> w849
                    frame 0, Default {
                      n731 = control-ref of="CODMn"() -> (w905:refnum<vi>)
                      n732 = property class="Bool (严格)"(reference=w905) -> ("Label.Text"=w904:string)  [unwired: 1 in, 2 out]
                    }
                    frame 1 {
                      n733 = control-ref of="CODCr"() -> (w907:refnum<vi>)
                      n734 = property class="Bool (严格)"(reference=w907) -> ("Label.Text"=w906:string)  [unwired: 1 in, 2 out]
                    }
                    frame 2 {
                      n735 = control-ref of="DO"() -> (w909:refnum<vi>)
                      n736 = property class="Bool (严格)"(reference=w909) -> ("Label.Text"=w908:string)  [unwired: 1 in, 2 out]
                    }
                    frame 3 {
                      n737 = control-ref of="DOperNULL"() -> (w911:refnum<vi>)
                      n738 = property class="Bool (严格)"(reference=w911) -> ("Label.Text"=w910:string)  [unwired: 1 in, 2 out]
                    }
                    frame 4 {
                      n739 = control-ref of="PH"() -> (w913:refnum<vi>)
                      n740 = property class="Bool (严格)"(reference=w913) -> ("Label.Text"=w912:string)  [unwired: 1 in, 2 out]
                    }
                    frame 5 {
                      n741 = control-ref of="氨氮"() -> (w915:refnum<vi>)
                      n742 = property class="Bool (严格)"(reference=w915) -> ("Label.Text"=w914:string)  [unwired: 1 in, 2 out]
                    }
                    frame 6 {
                      n743 = control-ref of="比电导率"() -> (w917:refnum<vi>)
                      n744 = property class="Bool (严格)"(reference=w917) -> ("Label.Text"=w916:string)  [unwired: 1 in, 2 out]
                    }
                    frame 7 {
                      n745 = control-ref of="水温"() -> (w919:refnum<vi>)
                      n746 = property class="Bool (严格)"(reference=w919) -> ("Label.Text"=w918:string)  [unwired: 1 in, 2 out]
                    }
                    frame 8 {
                      n747 = control-ref of="盐度(海水)"() -> (w921:refnum<vi>)
                      n748 = property class="Bool (严格)"(reference=w921) -> ("Label.Text"=w920:string)  [unwired: 1 in, 2 out]
                    }
                    frame 9 {
                      n749 = control-ref of="浊度"() -> (w923:refnum<vi>)
                      n750 = property class="Bool (严格)"(reference=w923) -> ("Label.Text"=w922:string)  [unwired: 1 in, 2 out]
                    }
                    frame 10 {
                      n751 = control-ref of="总氮"() -> (w925:refnum<vi>)
                      n752 = property class="Bool (严格)"(reference=w925) -> ("Label.Text"=w924:string)  [unwired: 1 in, 2 out]
                    }
                    frame 11 {
                      n753 = control-ref of="总磷"() -> (w927:refnum<vi>)
                      n754 = property class="Bool (严格)"(reference=w927) -> ("Label.Text"=w926:string)  [unwired: 1 in, 2 out]
                    }
                    frame 12 {
                      n755 = control-ref of="叶绿素a"() -> (w929:refnum<vi>)
                      n756 = property class="Bool (严格)"(reference=w929) -> ("Label.Text"=w928:string)  [unwired: 1 in, 2 out]
                    }
                    frame 13 {
                      n757 = control-ref of="藻密度"() -> (w931:refnum<vi>)
                      n758 = property class="Bool (严格)"(reference=w931) -> ("Label.Text"=w930:string)  [unwired: 1 in, 2 out]
                    }
                    frame 14 {
                      n759 = control-ref of="水位"() -> (w933:refnum<vi>)
                      n760 = property class="Bool (严格)"(reference=w933) -> ("Label.Text"=w932:string)  [unwired: 1 in, 2 out]
                    }
                    frame 15 {
                      n761 = control-ref of="流速"() -> (w935:refnum<vi>)
                      n762 = property class="Bool (严格)"(reference=w935) -> ("Label.Text"=w934:string)  [unwired: 1 in, 2 out]
                    }
                    frame 16 {
                      n763 = control-ref of="瞬时流量"() -> (w937:refnum<vi>)
                      n764 = property class="Bool (严格)"(reference=w937) -> ("Label.Text"=w936:string)  [unwired: 1 in, 2 out]
                    }
                    frame 17 {
                      n765 = control-ref of="累积流量"() -> (w939:refnum<vi>)
                      n766 = property class="Bool (严格)"(reference=w939) -> ("Label.Text"=w938:string)  [unwired: 1 in, 2 out]
                    }
                  }
                  n767 = Get Date/Time In Seconds() -> (seconds since 1Jan1904=w858:timestamp)
                  n768 = Format Date/Time String(time format string (%c)="%Y/%m/%d %H:%M:%S" ("时间格式字符串(%c)"), seconds (now)=w858) -> (date/time string=w848:string)  [unwired: 1 in]
                  n769 = Format Into String(format string="#%s#" ("初始字符串"), w847) -> (resulting string=w856:string)  [unwired: 2 in, 1 out]
                  n770 = Format Into String(format string="#%s#" ("初始字符串"), w848) -> (resulting string=w851:string)  [unwired: 2 in, 1 out]
                  n771 = case shown="0, 默认" w846 {
                    selector: w846 -> [_ w890]
                    tunnel: w856 -> [w885 w895]
                    tunnel: [w884 w896] -> w855
                    tunnel: w851 -> [w881 w894]
                    tunnel: w850 -> [_ w893]
                    tunnel: w849 -> [_ w892]
                    tunnel: w847 -> [_ w887]
                    tunnel: w848 -> [_ w889]
                    frame 0, Default {
                      n772 = Concatenate Strings("where 测量模式 ='水样测试" ("condition"), "'and 时间 between ", w885, "and" ("字符串"), w881, " order by 时间 desc" ("字符串")) -> (w884:string)
                    }
                    frame 14..17 {
                      n773 = call "流量数据规范小时时间戳.vi"("字符串"=w887) -> ("result string"=w886:string)  [unwired: 10 in]
                      n774 = call "database1查询.vi"("时间2"=w889, "table"=w892, "时间1"=w886, "database"=w893) -> ("error out"=w888:errorcluster, "data"=w891:string[][])  [unwired: 4 in, 1 out]
                      n775 = call <vilib>:"Clear Errors.vi"("error in (no error)"=w888) -> ()  [unwired: 5 in, 2 out]
                      n776 = case shown="14" w890 {
                        tunnel: w891 -> [_ w900 w901 w902 w903]
                        frame 0, Default {
                        }
                        frame 14 {
                          n777 = global write "全局流量数据小时.vi" "水位"(w900) -> ()
                        }
                        frame 15 {
                          n778 = global write "全局流量数据小时.vi" "流速"(w901) -> ()
                        }
                        frame 16 {
                          n779 = global write "全局流量数据小时.vi" "瞬时流量"(w902) -> ()
                        }
                        frame 17 {
                          n780 = global write "全局流量数据小时.vi" "累积流量"(w903) -> ()
                        }
                      }
                      n781 = Concatenate Strings(" where 时间 between ", w895, "and" ("字符串"), w894, " order by 时间 desc" ("字符串")) -> (w896:string)
                    }
                  }
                  n782 = call "SQL查询.vi"("condition"=w855, "table输入"=w849, "database"=w850) -> ("error out"=w852:errorcluster, "data"=w845:string[][])  [unwired: 7 in]
                  n783 = call "短日期时间转长日期格式.vi"("data"=w845) -> ("输出数组"=w853:string[][])  [unwired: 10 in]
                  n784 = case shown="12" w846 {
                    tunnel: w845 -> [w861 w862 w863 w864 w865 w866 w867 w868 w869 w870 w871 w872 w873 w874 w875 w876 w877 w878]
                    frame 0, Default {
                      n785 = global write "全局 所有参数.vi" "CODMn"(w861) -> ()
                    }
                    frame 1 {
                      n786 = global write "全局 所有参数.vi" "CODCr"(w862) -> ()
                    }
                    frame 2 {
                      n787 = global write "全局 所有参数.vi" "DO"(w863) -> ()
                    }
                    frame 3 {
                      n788 = global write "全局 所有参数.vi" "DOper"(w864) -> ()
                    }
                    frame 4 {
                      n789 = global write "全局 所有参数.vi" "PH"(w865) -> ()
                    }
                    frame 5 {
                      n790 = global write "全局 所有参数.vi" "氨氮"(w866) -> ()
                    }
                    frame 6 {
                      n791 = global write "全局 所有参数.vi" "电导率"(w867) -> ()
                    }
                    frame 7 {
                      n792 = global write "全局 所有参数.vi" "水温"(w868) -> ()
                    }
                    frame 8 {
                      n793 = global write "全局 所有参数.vi" "盐度"(w869) -> ()
                    }
                    frame 9 {
                      n794 = global write "全局 所有参数.vi" "浊度"(w870) -> ()
                    }
                    frame 10 {
                      n795 = global write "全局 所有参数.vi" "总氮"(w871) -> ()
                    }
                    frame 11 {
                      n796 = global write "全局 所有参数.vi" "总磷"(w872) -> ()
                    }
                    frame 12 {
                      n797 = global write "全局 所有参数.vi" "叶绿素"(w873) -> ()
                    }
                    frame 13 {
                      n798 = global write "全局 所有参数.vi" "藻密度"(w874) -> ()
                    }
                    frame 14 {
                      n799 = global write "全局 所有参数.vi" "水位"(w875) -> ()
                    }
                    frame 15 {
                      n800 = global write "全局 所有参数.vi" "流速"(w876) -> ()
                    }
                    frame 16 {
                      n801 = global write "全局 所有参数.vi" "瞬时流量"(w877) -> ()
                    }
                    frame 17 {
                      n802 = global write "全局 所有参数.vi" "累积流量"(w878) -> ()
                    }
                  }
                  n803 = Index Array(array=w853, index (row)=w854, index (col)=w854) -> ()  [unwired: 1 out]
                }
                n804 = flat-sequence {
                  tunnel: w806 -> [w809]
                  tunnel: [w809] -> w805
                  tunnel: w805 -> [w815]
                  tunnel: [w814] -> _
                  frame #0 {
                    n805 = global write "全局 小时数据发送次数.vi" "小时数据发送次数"(0 ("小时数据发送次数")) -> ()
                    n806 = call "数据处理直接插入整合 (子VI).vi"() -> ()  [unwired: 12 in]
                    n807 = global write "全局1.vi" "枚举"(enum16{"返回请求应答", "上传数据", "返回执行结果"}."上传数据" ("枚举")) -> ()
                    n808 = global write "全局 实时数据参数.vi" "实时数据参数"("水样测试" ("实时数据参数")) -> ()
                    n809 = global write "全局 水样时间.vi" "选择发送的参数"("氨氮" ("选择发送的参数")) -> ()
                  }
                  frame #1 {
                    # "实时数据的大小"
                    n810 = flat-sequence {
                      tunnel: [w821] -> w818
                      tunnel: [w820] -> w816
                      tunnel: w815 -> [w819]
                      tunnel: w818 -> [_]
                      tunnel: [w834] -> w817
                      tunnel: w816 -> [w834]
                      tunnel: w817 -> [w842]
                      tunnel: [w836] -> w814
                      frame #0 {
                        n811 = Get Date/Time In Seconds() -> (seconds since 1Jan1904=w829:timestamp)
                        n812 = Format Date/Time String(time format string (%c)="%Y%m%d%H%M%S%3u" ("时间格式字符串(%c)"), seconds (now)=w829) -> (date/time string=w830:string)  [unwired: 1 in]
                        n813 = Search and Replace String(input string=w830, search string="." ("搜索字符串")) -> (result string=w832:string)  [unwired: 6 in, 3 out]
                        n814 = local read "MN"() -> (w825:string)
                        n815 = local read "PW"() -> (w824:string)
                        n816 = local read "数据发送通道"() -> (w823:enum16{"TCP", "VISA"})
                        n817 = call "数据编码.vi"("table输入"="小时数据" ("新元素/子数组"), "QN"=w832, "MN"=w825, "PW"=w824) -> ("通讯包字符串"=w821:string)  [unwired: 10 in, 1 out]
                        n818 = Build Array(w821) -> (w826:string[])
                        n819 = local write "发送报文显示"(w821) -> ()
                        n820 = call "VISATCP组合选择发送.vi"("数据发送通道"=w823, "命令"="write", "写入缓冲区"=w821) -> ()  [unwired: 9 in, 4 out]
                        n821 = call "发送数据记录到文档(子VI).vi"("错误输入"=w819, "数组"=w826) -> ("错误输出"=w820:errorcluster)  [unwired: 8 in]
                      }
                      frame #1 {
                        n822 = global write "全局 小时数据发送次数.vi" "小时数据发送次数"(0 ("小时数据发送次数")) -> ()
                        n823 = Wait (ms)(milliseconds to wait=u32 500 ("等待时间（毫秒）")) -> ()  [unwired: 1 out]
                      }
                      frame #2 {
                        n824 = local read "MN"() -> (w841:string)
                        n825 = local read "PW"() -> (w840:string)
                        n826 = call "数据编码.vi"("table输入"="实时数据" ("新元素/子数组"), "错误常量 2"=w842, "MN"=w841, "PW"=w840) -> ("通讯包字符串"=w837:string)  [unwired: 10 in, 1 out]
                        n827 = Build Array(w837) -> (w844:string[])
                        n828 = local read "数据发送通道"() -> (w839:enum16{"TCP", "VISA"})
                        n829 = local write "发送报文显示"(w837) -> ()
                        n830 = call "发送数据记录到文档(子VI).vi"("数组"=w844) -> ()  [unwired: 9 in, 1 out]
                        n831 = call "VISATCP组合选择发送.vi"("数据发送通道"=w839, "命令"="write", "写入缓冲区"=w837) -> ("错误输出"=w836:errorcluster)  [unwired: 9 in, 3 out]
                      }
                    }
                  }
                }
              }
              frame "2017-212协议", Default {
                n832 = local read "参数数值"() -> (w942:T5)
                n833 = Cluster To Array(cluster=w942) -> (array=w941:bool[])
                n834 = for {
                  tunnel: w941 -> [_] mode=indexing
                  tunnel: [w949] -> w940 mode=indexing
                  tunnel: [w949] -> _
                  i -> [w947]
                  (unwired) " where 时间 between #"
                  w946 = "database1.mdb" ("database")
                  (unwired) "'and 数据类型 ='N' and 时间 between "
                  w963 = 0 ("索引 (行)")
                  n835 = case shown="8" w947 {
                    tunnel: [w1142 w1144 w1146 w1148 w1150 w1152 w1154 w1156 w1158 w1160 w1162 w1164 w1166 w1168 w1170 w1172 w1174 w1176] -> w945
                    frame 0, Default {
                      n836 = control-ref of="CODMn"() -> (w1143:refnum<vi>)
                      n837 = property class="Bool (严格)"(reference=w1143) -> ("Label.Text"=w1142:string)  [unwired: 1 in, 2 out]
                    }
                    frame 1 {
                      n838 = control-ref of="CODCr"() -> (w1145:refnum<vi>)
                      n839 = property class="Bool (严格)"(reference=w1145) -> ("Label.Text"=w1144:string)  [unwired: 1 in, 2 out]
                    }
                    frame 2 {
                      n840 = control-ref of="DO"() -> (w1147:refnum<vi>)
                      n841 = property class="Bool (严格)"(reference=w1147) -> ("Label.Text"=w1146:string)  [unwired: 1 in, 2 out]
                    }
                    frame 3 {
                      n842 = control-ref of="DOperNULL"() -> (w1149:refnum<vi>)
                      n843 = property class="Bool (严格)"(reference=w1149) -> ("Label.Text"=w1148:string)  [unwired: 1 in, 2 out]
                    }
                    frame 4 {
                      n844 = control-ref of="PH"() -> (w1151:refnum<vi>)
                      n845 = property class="Bool (严格)"(reference=w1151) -> ("Label.Text"=w1150:string)  [unwired: 1 in, 2 out]
                    }
                    frame 5 {
                      n846 = control-ref of="氨氮"() -> (w1153:refnum<vi>)
                      n847 = property class="Bool (严格)"(reference=w1153) -> ("Label.Text"=w1152:string)  [unwired: 1 in, 2 out]
                    }
                    frame 6 {
                      n848 = control-ref of="比电导率"() -> (w1155:refnum<vi>)
                      n849 = property class="Bool (严格)"(reference=w1155) -> ("Label.Text"=w1154:string)  [unwired: 1 in, 2 out]
                    }
                    frame 7 {
                      n850 = control-ref of="水温"() -> (w1157:refnum<vi>)
                      n851 = property class="Bool (严格)"(reference=w1157) -> ("Label.Text"=w1156:string)  [unwired: 1 in, 2 out]
                    }
                    frame 8 {
                      n852 = control-ref of="盐度(海水)"() -> (w1159:refnum<vi>)
                      n853 = property class="Bool (严格)"(reference=w1159) -> ("Label.Text"=w1158:string)  [unwired: 1 in, 2 out]
                    }
                    frame 9 {
                      n854 = control-ref of="浊度"() -> (w1161:refnum<vi>)
                      n855 = property class="Bool (严格)"(reference=w1161) -> ("Label.Text"=w1160:string)  [unwired: 1 in, 2 out]
                    }
                    frame 10 {
                      n856 = control-ref of="总氮"() -> (w1163:refnum<vi>)
                      n857 = property class="Bool (严格)"(reference=w1163) -> ("Label.Text"=w1162:string)  [unwired: 1 in, 2 out]
                    }
                    frame 11 {
                      n858 = control-ref of="总磷"() -> (w1165:refnum<vi>)
                      n859 = property class="Bool (严格)"(reference=w1165) -> ("Label.Text"=w1164:string)  [unwired: 1 in, 2 out]
                    }
                    frame 12 {
                      n860 = control-ref of="叶绿素a"() -> (w1167:refnum<vi>)
                      n861 = property class="Bool (严格)"(reference=w1167) -> ("Label.Text"=w1166:string)  [unwired: 1 in, 2 out]
                    }
                    frame 13 {
                      n862 = control-ref of="藻密度"() -> (w1169:refnum<vi>)
                      n863 = property class="Bool (严格)"(reference=w1169) -> ("Label.Text"=w1168:string)  [unwired: 1 in, 2 out]
                    }
                    frame 14 {
                      n864 = control-ref of="水位"() -> (w1171:refnum<vi>)
                      n865 = property class="Bool (严格)"(reference=w1171) -> ("Label.Text"=w1170:string)  [unwired: 1 in, 2 out]
                    }
                    frame 15 {
                      n866 = control-ref of="流速"() -> (w1173:refnum<vi>)
                      n867 = property class="Bool (严格)"(reference=w1173) -> ("Label.Text"=w1172:string)  [unwired: 1 in, 2 out]
                    }
                    frame 16 {
                      n868 = control-ref of="瞬时流量"() -> (w1175:refnum<vi>)
                      n869 = property class="Bool (严格)"(reference=w1175) -> ("Label.Text"=w1174:string)  [unwired: 1 in, 2 out]
                    }
                    frame 17 {
                      n870 = control-ref of="累积流量"() -> (w1177:refnum<vi>)
                      n871 = property class="Bool (严格)"(reference=w1177) -> ("Label.Text"=w1176:string)  [unwired: 1 in, 2 out]
                    }
                  }
                  n872 = case shown="12" w947 {
                    tunnel: [w1124 w1125 w1126 w1127 w1128 w1129 w1130 w1131 w1132 w1133 w1134 w1135 w1136 w1137 w1138 w1139 w1140 w1141] -> w944
                    frame 0, Default {
                      n873 = global read "全局 水样时间.vi" "time1"() -> (w1124:string)
                    }
                    frame 1 {
                      n874 = global read "全局 水样时间.vi" "time2"() -> (w1125:string)
                    }
                    frame 2 {
                      n875 = global read "全局 水样时间.vi" "time3"() -> (w1126:string)
                    }
                    frame 3 {
                      n876 = global read "全局 水样时间.vi" "time4"() -> (w1127:string)
                    }
                    frame 4 {
                      n877 = global read "全局 水样时间.vi" "time5"() -> (w1128:string)
                    }
                    frame 5 {
                      n878 = global read "全局 水样时间.vi" "time6"() -> (w1129:string)
                    }
                    frame 6 {
                      n879 = global read "全局 水样时间.vi" "time7"() -> (w1130:string)
                    }
                    frame 7 {
                      n880 = global read "全局 水样时间.vi" "time8"() -> (w1131:string)
                    }
                    frame 8 {
                      n881 = global read "全局 水样时间.vi" "time9"() -> (w1132:string)
                    }
                    frame 9 {
                      n882 = global read "全局 水样时间.vi" "time10"() -> (w1133:string)
                    }
                    frame 10 {
                      n883 = global read "全局 水样时间.vi" "time11"() -> (w1134:string)
                    }
                    frame 11 {
                      n884 = global read "全局 水样时间.vi" "time12"() -> (w1135:string)
                    }
                    frame 12 {
                      n885 = global read "全局 水样时间.vi" "time13"() -> (w1136:string)
                    }
                    frame 13 {
                      n886 = global read "全局 水样时间.vi" "time14"() -> (w1137:string)
                    }
                    frame 14 {
                      n887 = global read "全局 水样时间.vi" "time15"() -> (w1138:string)
                    }
                    frame 15 {
                      n888 = global read "全局 水样时间.vi" "time16"() -> (w1139:string)
                    }
                    frame 16 {
                      n889 = global read "全局 水样时间.vi" "time17"() -> (w1140:string)
                    }
                    frame 17 {
                      n890 = global read "全局 水样时间.vi" "time18"() -> (w1141:string)
                    }
                  }
                  n891 = Get Date/Time In Seconds() -> (seconds since 1Jan1904=w968:timestamp)
                  n892 = Format Date/Time String(time format string (%c)="%Y/%m/%d %H:%M:%S" ("时间格式字符串(%c)"), seconds (now)=w968) -> (date/time string=w943:string)  [unwired: 1 in]
                  n893 = Format Into String(format string="#%s#" ("初始字符串"), w944) -> (resulting string=w966:string)  [unwired: 2 in, 1 out]
                  n894 = Format Into String(format string="#%s#" ("初始字符串"), w943) -> (resulting string=w948:string)  [unwired: 2 in, 1 out]
                  n895 = case shown="0, 默认" w947 {
                    selector: w947 -> [_ w982]
                    tunnel: w966 -> [w977 w987]
                    tunnel: [w976 w988] -> w965
                    tunnel: w948 -> [w973 w986]
                    tunnel: w946 -> [_ w985]
                    tunnel: w945 -> [_ w984]
                    tunnel: w944 -> [_ w979]
                    tunnel: w943 -> [_ w981]
                    frame 0, Default {
                      n896 = Concatenate Strings("where 测量模式 ='水样测试" ("condition"), "'and 时间 between ", w977, "and" ("字符串"), w973, " order by 时间 desc" ("字符串")) -> (w976:string)
                    }
                    frame 14..17 {
                      n897 = call "流量数据规范小时时间戳.vi"("字符串"=w979) -> ("result string"=w978:string)  [unwired: 10 in]
                      n898 = call "database1查询.vi"("时间2"=w981, "table"=w984, "时间1"=w978, "database"=w985) -> ("error out"=w980:errorcluster, "data"=w983:string[][])  [unwired: 4 in, 1 out]
                      n899 = call <vilib>:"Clear Errors.vi"("error in (no error)"=w980) -> ()  [unwired: 5 in, 2 out]
                      n900 = case shown="14" w982 {
                        tunnel: w983 -> [_ w992 w993 w994 w995]
                        frame 0, Default {
                        }
                        frame 14 {
                          n901 = global write "全局流量数据小时.vi" "水位"(w992) -> ()
                        }
                        frame 15 {
                          n902 = global write "全局流量数据小时.vi" "流速"(w993) -> ()
                        }
                        frame 16 {
                          n903 = global write "全局流量数据小时.vi" "瞬时流量"(w994) -> ()
                        }
                        frame 17 {
                          n904 = global write "全局流量数据小时.vi" "累积流量"(w995) -> ()
                        }
                      }
                      n905 = Concatenate Strings(" where 时间 between ", w987, "and" ("字符串"), w986, " order by 时间 desc" ("字符串")) -> (w988:string)
                    }
                  }
                  n906 = call "SQL查询.vi"("condition"=w965, "table输入"=w945, "database"=w946) -> ("error out"=w949:errorcluster, "data"=w961:string[][])  [unwired: 7 in]
                  n907 = Empty Array?(array=w961) -> (empty?=w964:bool)
                  n908 = call "短日期时间转长日期格式.vi"("data"=w961) -> ("输出数组"=w962:string[][])  [unwired: 10 in]
                  n909 = Not(x=w964) -> (.not. x?=w958:bool)
                  n910 = Index Array(array=w962, index (row)=w963, index (col)=w963) -> (element=w955:string)
                  n911 = global write "全局 水样时间.vi" "选择发送的参数"(w945) -> ()
                  n912 = flat-sequence {
                    tunnel: [w1003] -> w960
                    tunnel: [w1002] -> w959
                    tunnel: w958 -> [w1003]
                    tunnel: w961 -> [w1002]
                    tunnel: w947 -> [w997]
                    tunnel: w945 -> [w999]
                    tunnel: [w999] -> w956
                    tunnel: w955 -> [w998]
                    tunnel: [w998] -> w953
                    tunnel: [w997] -> w950
                    tunnel: w960 -> [w1023]
                    tunnel: w959 -> [w1026]
                    tunnel: [w1025] -> w957
                    tunnel: w956 -> [w1025]
                    tunnel: [w1024] -> w954
                    tunnel: w953 -> [w1024]
                    tunnel: [w1023] -> w952
                    tunnel: [w1022] -> w951
                    tunnel: w950 -> [w1022]
                    tunnel: w957 -> [w1092]
                    tunnel: w954 -> [w1091]
                    tunnel: w952 -> [w1089]
                    tunnel: w951 -> [w1090]
                    frame #0 {
                      n913 = case shown="12" w997 {
                        tunnel: w1002 -> [w1004 w1005 w1006 w1007 w1008 w1009 w1010 w1011 w1012 w1013 w1014 w1015 w1016 w1017 w1018 w1019 w1020 w1021]
                        frame 0, Default {
                          n914 = global write "全局 所有参数.vi" "CODMn"(w1004) -> ()
                        }
                        frame 1 {
                          n915 = global write "全局 所有参数.vi" "CODCr"(w1005) -> ()
                        }
                        frame 2 {
                          n916 = global write "全局 所有参数.vi" "DO"(w1006) -> ()
                        }
                        frame 3 {
                          n917 = global write "全局 所有参数.vi" "DOper"(w1007) -> ()
                        }
                        frame 4 {
                          n918 = global write "全局 所有参数.vi" "PH"(w1008) -> ()
                        }
                        frame 5 {
                          n919 = global write "全局 所有参数.vi" "氨氮"(w1009) -> ()
                        }
                        frame 6 {
                          n920 = global write "全局 所有参数.vi" "电导率"(w1010) -> ()
                        }
                        frame 7 {
                          n921 = global write "全局 所有参数.vi" "水温"(w1011) -> ()
                        }
                        frame 8 {
                          n922 = global write "全局 所有参数.vi" "盐度"(w1012) -> ()
                        }
                        frame 9 {
                          n923 = global write "全局 所有参数.vi" "浊度"(w1013) -> ()
                        }
                        frame 10 {
                          n924 = global write "全局 所有参数.vi" "总氮"(w1014) -> ()
                        }
                        frame 11 {
                          n925 = global write "全局 所有参数.vi" "总磷"(w1015) -> ()
                        }
                        frame 12 {
                          n926 = global write "全局 所有参数.vi" "叶绿素"(w1016) -> ()
                        }
                        frame 13 {
                          n927 = global write "全局 所有参数.vi" "藻密度"(w1017) -> ()
                        }
                        frame 14 {
                          n928 = global write "全局 所有参数.vi" "水位"(w1018) -> ()
                        }
                        frame 15 {
                          n929 = global write "全局 所有参数.vi" "流速"(w1019) -> ()
                        }
                        frame 16 {
                          n930 = global write "全局 所有参数.vi" "瞬时流量"(w1020) -> ()
                        }
                        frame 17 {
                          n931 = global write "全局 所有参数.vi" "累积流量"(w1021) -> ()
                        }
                      }
                      n932 = global write "全局 小时数据发送次数.vi" "小时数据发送次数"(0 ("小时数据发送次数")) -> ()
                      n933 = global write "全局 数据发送重叠.vi" "数据接收超时指示灯"(FALSE ("数据接收超时指示灯")) -> ()
                      n934 = global write "全局1.vi" "枚举"(enum16{"返回请求应答", "上传数据", "返回执行结果"}."上传数据" ("枚举")) -> ()
                    }
                    frame #1 {
                      n935 = case shown="真" w1023 {
                        tunnel: w1026 -> [_ w1029]
                        tunnel: w1022 -> [_ w1028]
                        tunnel: w1022 -> [_ w1027]
                        frame False {
                        }
                        frame True {
                          n936 = for {
                            tunnel: w1029 -> [_] mode=indexing
                            tunnel: w1028 -> [w1031]
                            tunnel: w1027 -> [w1030]
                            # "实时数据的大小"
                            n937 = Wait (ms)(milliseconds to wait=u32 500 ("等待时间（毫秒）")) -> ()  [unwired: 1 out]
                            n938 = flat-sequence {
                              tunnel: [w1037] -> w1033
                              tunnel: w1033 -> [w1052]
                              tunnel: [w1053] -> w1032
                              tunnel: w1031 -> [w1051]
                              tunnel: [w1064] -> w1035
                              tunnel: [w1063] -> w1034
                              tunnel: w1032 -> [w1069]
                              tunnel: w1035 -> [w1075]
                              tunnel: w1034 -> [w1074]
                              tunnel: w1030 -> [w1073]
                              frame #0 {
                                n939 = global write "全局 实时数据参数.vi" "实时数据参数"("水样测试" ("实时数据参数")) -> ()
                                n940 = Get Date/Time In Seconds() -> (seconds since 1Jan1904=w1046:timestamp)
                                n941 = Format Date/Time String(time format string (%c)="%Y%m%d%H%M%S%3u" ("时间格式字符串(%c)"), seconds (now)=w1046) -> (date/time string=w1047:string)  [unwired: 1 in]
                                n942 = Search and Replace String(input string=w1047, search string="." ("搜索字符串")) -> (result string=w1049:string)  [unwired: 6 in, 3 out]
                                n943 = local read "MN"() -> (w1041:string)
                                n944 = local read "PW"() -> (w1040:string)
                                n945 = local read "数据发送通道"() -> (w1039:enum16{"TCP", "VISA"})
                                n946 = call "数据编码.vi"("table输入"="小时数据" ("新元素/子数组"), "QN"=w1049, "MN"=w1041, "PW"=w1040) -> ("通讯包字符串"=w1037:string)  [unwired: 10 in, 1 out]
                                n947 = Build Array(w1037) -> (w1043:string[])
                                n948 = local write "发送报文显示"(w1037) -> ()
                                n949 = call "VISATCP组合选择发送.vi"("数据发送通道"=w1039, "命令"="write", "写入缓冲区"=w1037) -> ()  [unwired: 9 in, 4 out]
                                n950 = call "发送数据记录到文档(子VI).vi"("数组"=w1043) -> ()  [unwired: 9 in, 1 out]
                              }
                              frame #1 {
                                n951 = local read "数据发送协议"() -> (w1050:enum16{"2005-212协议", "2017-212协议"})
                                n952 = case shown="\"2017-212协议\", 默认" w1050 {
                                tunnel: [_ w1056] -> w1053
                                tunnel: w1052 -> [_ w1055]
                                tunnel: w1051 -> [_ w1054]
                                frame "2005-212协议" {
                                }
                                frame "2017-212协议", Default {
                                n953 = case shown="0, 默认" w1054 {
                                tunnel: [w1058 _] -> w1056
                                tunnel: w1055 -> [w1057 _]
                                frame 0, Default {
                                n954 = Empty String/Path?(string/path=w1057) -> (empty?=w1059:bool)
                                n955 = case shown="假" w1059 {
                                tunnel: [w1062 _] -> w1058
                                tunnel: w1057 -> [w1061 _]
                                frame False {
                                n956 = local read "数据发送通道"() -> (w1060:enum16{"TCP", "VISA"})
                                n957 = call "数据补发判定有限循环.vi"("数据输入"=w1061, "数据发送通道"=w1060) -> ("error out"=w1062:errorcluster)  [unwired: 9 in]
                                }
                                frame True {
                                }
                                }
                                }
                                frame 14..17 {
                                }
                                }
                                }
                                }
                              }
                              frame #2 {
                                n958 = local read "MN"() -> (w1068:string)
                                n959 = local read "PW"() -> (w1067:string)
                                n960 = call "数据编码.vi"("table输入"="实时数据" ("新元素/子数组"), "错误常量 2"=w1069, "MN"=w1068, "PW"=w1067) -> ("通讯包字符串"=w1064:string)  [unwired: 10 in, 1 out]
                                n961 = Build Array(w1064) -> (w1071:string[])
                                n962 = local read "数据发送通道"() -> (w1066:enum16{"TCP", "VISA"})
                                n963 = local write "发送报文显示"(w1064) -> ()
                                n964 = call "发送数据记录到文档(子VI).vi"("数组"=w1071) -> ()  [unwired: 9 in, 1 out]
                                n965 = call "VISATCP组合选择发送.vi"("数据发送通道"=w1066, "命令"="write", "写入缓冲区"=w1064) -> ("错误输出"=w1063:errorcluster)  [unwired: 9 in, 3 out]
                              }
                              frame #3 {
                                n966 = local read "数据发送协议"() -> (w1072:enum16{"2005-212协议", "2017-212协议"})
                                n967 = case shown="\"2005-212协议\"" w1072 {
                                tunnel: w1075 -> [_ w1078]
                                tunnel: w1074 -> [_ w1077]
                                tunnel: w1073 -> [_ w1076]
                                frame "2005-212协议" {
                                }
                                frame "2017-212协议", Default {
                                n968 = case shown="0, 默认" w1076 {
                                tunnel: w1078 -> [w1082 _]
                                tunnel: w1077 -> [w1081 _]
                                frame 0, Default {
                                n969 = local read "数据发送通道"() -> (w1079:enum16{"TCP", "VISA"})
                                n970 = call "数据补发判定有限循环.vi"("错误输入（无错误）"=w1081, "数据输入"=w1082, "数据发送通道"=w1079) -> ("error out"=w1080:errorcluster)  [unwired: 8 in]
                                n971 = local write "错误输出"(w1080) -> ()
                                }
                                frame 14..17 {
                                }
                                }
                                }
                                }
                              }
                            }
                          }
                        }
                      }
                    }
                    frame #2 {
                      n972 = global read "全局 数据发送重叠.vi" "数据接收超时指示灯"() -> (w1086:bool)
                      n973 = Not(x=w1086) -> (.not. x?=w1087:bool)
                      n974 = local read "数据发送协议"() -> (w1085:enum16{"2005-212协议", "2017-212协议"})
                      n975 = Equal?(x=w1085, y=enum16{"2005-212协议", "2017-212协议"}."2017-212协议" ("数据发送协议")) -> (x = y?=w1083:bool)
                      n976 = Compound Arithmetic op=AND ("复合运算")(w1083, w1087, w1089) -> (w1088:bool)
                      n977 = case shown="真" w1088 {
                        tunnel: w1091 -> [_ w1095]
                        tunnel: w1090 -> [_ w1105]
                        tunnel: w1092 -> [_ w1096]
                        frame False {
                        }
                        frame True {
                          n978 = call "日期时间字符串转换分钟数加一.vi"("data[0]"=w1095) -> ("日期/时间字符串"=w1093:string)  [unwired: 10 in]
                          n979 = call "时间日期字符串至时间标识转换.vi"("时间日期字符串"=w1093) -> ("时间标识"=w1094:timestamp)  [unwired: 10 in]
                          n980 = call <vilib>:"Application Directory.vi"() -> ("Application Directory"=w1097:path)
                          n981 = case shown="12" w1105 {
                            tunnel: w1093 -> [w1106 w1107 w1108 w1109 w1110 w1111 w1112 w1113 w1114 w1115 w1116 w1117 w1118 w1119 w1120 w1121 w1122 w1123]
                            frame 0, Default {
                              n982 = global write "全局 水样时间.vi" "time1"(w1106) -> ()
                            }
                            frame 1 {
                              n983 = global write "全局 水样时间.vi" "time2"(w1107) -> ()
                            }
                            frame 2 {
                              n984 = global write "全局 水样时间.vi" "time3"(w1108) -> ()
                            }
                            frame 3 {
                              n985 = global write "全局 水样时间.vi" "time4"(w1109) -> ()
                            }
                            frame 4 {
                              n986 = global write "全局 水样时间.vi" "time5"(w1110) -> ()
                            }
                            frame 5 {
                              n987 = global write "全局 水样时间.vi" "time6"(w1111) -> ()
                            }
                            frame 6 {
                              n988 = global write "全局 水样时间.vi" "time7"(w1112) -> ()
                            }
                            frame 7 {
                              n989 = global write "全局 水样时间.vi" "time8"(w1113) -> ()
                            }
                            frame 8 {
                              n990 = global write "全局 水样时间.vi" "time9"(w1114) -> ()
                            }
                            frame 9 {
                              n991 = global write "全局 水样时间.vi" "time10"(w1115) -> ()
                            }
                            frame 10 {
                              n992 = global write "全局 水样时间.vi" "time11"(w1116) -> ()
                            }
                            frame 11 {
                              n993 = global write "全局 水样时间.vi" "time12"(w1117) -> ()
                            }
                            frame 12 {
                              n994 = global write "全局 水样时间.vi" "time13"(w1118) -> ()
                            }
                            frame 13 {
                              n995 = global write "全局 水样时间.vi" "time14"(w1119) -> ()
                            }
                            frame 14 {
                              n996 = global write "全局 水样时间.vi" "time15"(w1120) -> ()
                            }
                            frame 15 {
                              n997 = global write "全局 水样时间.vi" "time16"(w1121) -> ()
                            }
                            frame 16 {
                              n998 = global write "全局 水样时间.vi" "time17"(w1122) -> ()
                            }
                            frame 17 {
                              n999 = global write "全局 水样时间.vi" "time18"(w1123) -> ()
                            }
                          }
                          n1000 = Build Path(base path=w1097, name or relative path="data\\Set.ini" ("名称或相对路径")) -> (appended path=w1099:path)
                          n1001 = call <vilib>:"Open Config Data.vi"("configuration file path"=w1099) -> ("error out"=w1101:errorcluster, "refnum"=w1100:T8)  [unwired: 8 in, 1 out]
                          n1002 = local write "数据发送起始时间"(w1094) -> ()
                          n1003 = call-poly <vilib>:"Write Key.vi"("section"="线程一数据搜索起始时间", "error in (no error)"=w1101, "value"=w1093, "key"=w1096, "refnum"=w1100) -> ("error out"=w1103:errorcluster, "refnum out"=w1102:T8)  [unwired: 4 in, 1 out]
                          n1004 = call <vilib>:"Close Config Data.vi"("error in (no error)"=w1103, "refnum"=w1102) -> ()  [unwired: 8 in, 2 out]
                        }
                      }
                    }
                  }
                }
              }
            }
          }
          frame #2 {
            w1178 = FALSE ("小时数据上传")
            n1005 = local write "实时小时数据上传"(w1178) -> ()
            n1006 = global write "全局 数据发送重叠.vi" "主动上报数据中"(w1178) -> ()
          }
        }
      }
    }
  }
  n1007 = while {
    stop <- FALSE stop-if-true
    # "定期释放缓存"
    n1008 = Wait (ms)(milliseconds to wait=u32 600000 ("等待时间（毫秒）")) -> ()  [unwired: 1 out]
    n1009 = dll-call lib="PTH2`abs F程序<平台数采程序 - 通用（小时数据单参数传）XINdataFreeMem.dll" fn="FreeMem"() -> ()  [unwired: 4 in, 2 out]
  }
  n1010 = while {
    stop <- FALSE stop-if-true
    n1011 = event shown="[7] \"数据发送协议\": 值改变" {
      selector: _ -> [_ _ _ _ _ _ _ _ _ _ _ _ _ _ _ _ _]
      dyn-events: _ -> [_ _ _ _ _ _ _ _ _ _ _ _ _ _ _ _ _]
      timeout: _ -> [_ _ _ _ _ _ _ _ _ _ _ _ _ _ _ _ _]
      event Timeout {
        n1012 = event-data() -> ()  [unwired: 1 in, 2 out]
      }
      event "站点名称", "站点设备", "IP", "PORT", "MN", "PW", "VISA resource name", "baud rate": Value Change {
        w1185 = "线程一自主部署站点保存"
        # "TCP服务器端口掉线"
        n1013 = event-data() -> ()  [unwired: 1 in, 6 out]
        n1014 = call <vilib>:"Application Directory.vi"() -> ("Application Directory"=w1227:path)
        n1015 = local read "站点名称"() -> (w1206:string)
        n1016 = Build Path(base path=w1227, name or relative path="data\\Set.ini" ("名称或相对路径")) -> (appended path=w1225:path)
        n1017 = call <vilib>:"Open Config Data.vi"("configuration file path"=w1225) -> ("error out"=w1223:errorcluster, "refnum"=w1224:T8)  [unwired: 8 in, 1 out]
        n1018 = local read "站点设备"() -> (w1205:string)
        n1019 = call-poly <vilib>:"Write Key.vi"("section"=w1185, "error in (no error)"=w1223, "value"=w1206, "key"="站点名称", "refnum"=w1224) -> ("error out"=w1220:errorcluster, "refnum out"=w1221:T8)  [unwired: 4 in, 1 out]
        n1020 = call-poly <vilib>:"Write Key.vi"("section"=w1185, "error in (no error)"=w1220, "value"=w1205, "key"="站点设备", "refnum"=w1221) -> ("error out"=w1217:errorcluster, "refnum out"=w1218:T8)  [unwired: 4 in, 1 out]
        n1021 = local read "IP"() -> (w1204:string)
        n1022 = call-poly <vilib>:"Write Key.vi"("section"=w1185, "error in (no error)"=w1217, "value"=w1204, "key"="IP", "refnum"=w1218) -> ("error out"=w1215:errorcluster, "refnum out"=w1216:T8)  [unwired: 4 in, 1 out]
        n1023 = local read "PORT"() -> (w1203:string)
        n1024 = call-poly <vilib>:"Write Key.vi"("section"=w1185, "error in (no error)"=w1215, "value"=w1203, "key"="PORT", "refnum"=w1216) -> ("error out"=w1213:errorcluster, "refnum out"=w1214:T8)  [unwired: 4 in, 1 out]
        n1025 = local read "MN"() -> (w1197:string)
        n1026 = call-poly <vilib>:"Write Key.vi"("section"=w1185, "error in (no error)"=w1213, "value"=w1197, "key"="MN", "refnum"=w1214) -> ("error out"=w1198:errorcluster, "refnum out"=w1201:T8)  [unwired: 4 in, 1 out]
        n1027 = local read "PW"() -> (w1199:string)
        n1028 = call-poly <vilib>:"Write Key.vi"("section"=w1185, "error in (no error)"=w1198, "value"=w1199, "key"="PW", "refnum"=w1201) -> ("error out"=w1186:errorcluster, "refnum out"=w1187:T8)  [unwired: 4 in, 1 out]
        n1029 = local read "VISA resource name"() -> (w1193:refnum<visa-resource-name>)
        n1030 = local read "主队列输出"() -> (w1212:refnum<queue>)
        n1031 = call-poly <vilib>:"Write Key.vi"("section"=w1185, "error in (no error)"=w1186, "value"=w1193, "key"="VISA", "refnum"=w1187) -> ("error out"=w1192:errorcluster, "refnum out"=w1189:T8)  [unwired: 4 in, 1 out]
        n1032 = local read "baud rate"() -> (w1191:u32)
        n1033 = Flush Queue(queue=w1212) -> (queue out=w1211:refnum<queue>)  [unwired: 1 in, 2 out]
        n1034 = call-poly <vilib>:"Write Key.vi"("section"=w1185, "error in (no error)"=w1192, "value"=w1191, "key"="BAUDRATE", "refnum"=w1189) -> ("error out"=w1183:errorcluster, "refnum out"=w1184:T8)  [unwired: 4 in, 1 out]
        n1035 = local read "数据发送通道"() -> (w1196:enum16{"TCP", "VISA"})
        n1036 = call <vilib>:"Close Config Data.vi"("error in (no error)"=w1183, "refnum"=w1184) -> ()  [unwired: 8 in, 2 out]
        n1037 = call "VISATCP组合选择发送.vi"("数据发送通道"=w1196, "命令"="close") -> ("错误输出"=w1194:errorcluster)  [unwired: 10 in, 3 out]
        n1038 = Enqueue Element(queue=w1211, element=T6."初始化" ("元素"), timeout in ms (-1)=1000 ("超时毫秒(-1)")) -> ()  [unwired: 1 in, 3 out]
        n1039 = call <vilib>:"Clear Errors.vi"("error in (no error)"=w1194) -> ()  [unwired: 5 in, 2 out]
      }
      event "确定": Value Change {
        w1232 = "线程一自主部署站点保存"
        # "TCP服务器端口掉线"
        n1040 = event-data() -> ()  [unwired: 1 in, 6 out]
        n1041 = call <vilib>:"Application Directory.vi"() -> ("Application Directory"=w1265:path)
        n1042 = local read "站点名称"() -> (w1260:string)
        n1043 = Build Path(base path=w1265, name or relative path="data\\Set.ini" ("名称或相对路径")) -> (appended path=w1263:path)
        n1044 = call <vilib>:"Open Config Data.vi"("configuration file path"=w1263) -> ("error out"=w1261:errorcluster, "refnum"=w1262:T8)  [unwired: 8 in, 1 out]
        n1045 = local read "站点设备"() -> (w1255:string)
        n1046 = call-poly <vilib>:"Write Key.vi"("section"=w1232, "error in (no error)"=w1261, "value"=w1260, "key"="站点名称", "refnum"=w1262) -> ("error out"=w1257:errorcluster, "refnum out"=w1258:T8)  [unwired: 4 in, 1 out]
        n1047 = call-poly <vilib>:"Write Key.vi"("section"=w1232, "error in (no error)"=w1257, "value"=w1255, "key"="站点设备", "refnum"=w1258) -> ("error out"=w1253:errorcluster, "refnum out"=w1254:T8)  [unwired: 4 in, 1 out]
        n1048 = local read "IP"() -> (w1248:string)
        n1049 = local read "PORT"() -> (w1247:string)
        n1050 = call-poly <vilib>:"Write Key.vi"("section"=w1232, "error in (no error)"=w1253, "value"=w1248, "key"="IP", "refnum"=w1254) -> ("error out"=w1251:errorcluster, "refnum out"=w1252:T8)  [unwired: 4 in, 1 out]
        n1051 = call-poly <vilib>:"Write Key.vi"("section"=w1232, "error in (no error)"=w1251, "value"=w1247, "key"="PORT", "refnum"=w1252) -> ("error out"=w1243:errorcluster, "refnum out"=w1244:T8)  [unwired: 4 in, 1 out]
        n1052 = local read "MN"() -> (w1240:string)
        n1053 = call-poly <vilib>:"Write Key.vi"("section"=w1232, "error in (no error)"=w1243, "value"=w1240, "key"="MN", "refnum"=w1244) -> ("error out"=w1241:errorcluster, "refnum out"=w1242:T8)  [unwired: 4 in, 1 out]
        n1054 = local read "PW"() -> (w1239:string)
        n1055 = call-poly <vilib>:"Write Key.vi"("section"=w1232, "error in (no error)"=w1241, "value"=w1239, "key"="PW", "refnum"=w1242) -> ("error out"=w1237:errorcluster, "refnum out"=w1238:T8)  [unwired: 4 in, 1 out]
        n1056 = call <vilib>:"Close Config Data.vi"("error in (no error)"=w1237, "refnum"=w1238) -> ("error out"=w1231:errorcluster)  [unwired: 8 in, 1 out]
        n1057 = local read "主队列输出"() -> (w1236:refnum<queue>)
        n1058 = local read "数据发送通道"() -> (w1230:enum16{"TCP", "VISA"})
        n1059 = call "VISATCP组合选择发送.vi"("数据发送通道"=w1230, "命令"="close") -> ("错误输出"=w1228:errorcluster)  [unwired: 10 in, 3 out]
        n1060 = Flush Queue(queue=w1236) -> (queue out=w1235:refnum<queue>)  [unwired: 1 in, 2 out]
        n1061 = case shown="错误" w1231 {
          frame No Error {
            n1062 = One Button Dialog(message="保存成功" ("消息"), button name ("OK")="确定" ("按钮名称（“确定”）")) -> ()  [unwired: 1 out]
          }
          frame Error {
            n1063 = One Button Dialog(message="保存失败" ("消息"), button name ("OK")="确定" ("按钮名称（“确定”）")) -> ()  [unwired: 1 out]
          }
        }
        n1064 = call <vilib>:"Clear Errors.vi"("error in (no error)"=w1228) -> ()  [unwired: 5 in, 2 out]
        n1065 = Enqueue Element(queue=w1235, element=T6."初始化" ("元素"), timeout in ms (-1)=1000 ("超时毫秒(-1)")) -> ()  [unwired: 1 in, 3 out]
      }
      event "参数配置": Value Change {
        n1066 = event-data() -> ()  [unwired: 1 in, 6 out]
        n1067 = property on="窗格" class="Pane"("Origin"=T11 {"Horizontal"=0, "Vertical"=1000} ("原点")) -> ()  [unwired: 2 in, 2 out]
      }
      event "返回": Value Change {
        n1068 = event-data() -> ()  [unwired: 1 in, 6 out]
        n1069 = property on="窗格" class="Pane"("Origin"=T11 {"Horizontal"=0, "Vertical"=0} ("原点")) -> ()  [unwired: 2 in, 2 out]
      }
      event "系统编码选择框": Value Change {
        n1070 = event-data() -> ()  [unwired: 1 in, 6 out]
        n1071 = call <vilib>:"Application Directory.vi"() -> ("Application Directory"=w1280:path)
        n1072 = Build Path(base path=w1280, name or relative path="data\\Set.ini" ("名称或相对路径")) -> (appended path=w1281:path)
        n1073 = call <vilib>:"Open Config Data.vi"("configuration file path"=w1281) -> ("error out"=w1277:errorcluster, "refnum"=w1278:T8)  [unwired: 8 in, 1 out]
        n1074 = call-poly <vilib>:"Write Key.vi"("section"="系统编码选择", "error in (no error)"=w1277, "value"="系统编码选择框", "key"="系统编码", "refnum"=w1278) -> ("error out"=w1275:errorcluster, "refnum out"=w1276:T8)  [unwired: 4 in, 1 out]
        n1075 = call <vilib>:"Close Config Data.vi"("error in (no error)"=w1275, "refnum"=w1276) -> ()  [unwired: 8 in, 2 out]
      }
      event "数据发送通道": Value Change {
        w1282 = "数据发送通道"
        n1076 = event-data() -> ()  [unwired: 1 in, 6 out]
        n1077 = local read "数据发送通道"() -> (w1283:enum16{"TCP", "VISA"})
        n1078 = call <vilib>:"Application Directory.vi"() -> ("Application Directory"=w1289:path)
        n1079 = Build Path(base path=w1289, name or relative path="data\\Set.ini" ("名称或相对路径")) -> (appended path=w1290:path)
        n1080 = call <vilib>:"Open Config Data.vi"("configuration file path"=w1290) -> ("error out"=w1286:errorcluster, "refnum"=w1287:T8)  [unwired: 8 in, 1 out]
        n1081 = call-poly <vilib>:"Write Key.vi"("section"=w1282, "error in (no error)"=w1286, "value"=w1283, "key"=w1282, "refnum"=w1287) -> ("error out"=w1284:errorcluster, "refnum out"=w1285:T8)  [unwired: 4 in, 1 out]
        n1082 = call <vilib>:"Close Config Data.vi"("error in (no error)"=w1284, "refnum"=w1285) -> ()  [unwired: 8 in, 2 out]
      }
      event "数据发送协议": Value Change {
        w1292 = "数据发送协议"
        n1083 = event-data() -> ()  [unwired: 1 in, 6 out]
        n1084 = call <vilib>:"Application Directory.vi"() -> ("Application Directory"=w1298:path)
        n1085 = Build Path(base path=w1298, name or relative path="data\\Set.ini" ("名称或相对路径")) -> (appended path=w1299:path)
        n1086 = call <vilib>:"Open Config Data.vi"("configuration file path"=w1299) -> ("error out"=w1295:errorcluster, "refnum"=w1296:T8)  [unwired: 8 in, 1 out]
        n1087 = call-poly <vilib>:"Write Key.vi"("section"=w1292, "error in (no error)"=w1295, "value"="数据发送协议", "key"=w1292, "refnum"=w1296) -> ("error out"=w1293:errorcluster, "refnum out"=w1294:T8)  [unwired: 4 in, 1 out]
        n1088 = call <vilib>:"Close Config Data.vi"("error in (no error)"=w1293, "refnum"=w1294) -> ()  [unwired: 8 in, 2 out]
      }
      event "每周自动重发": Value Change {
        n1089 = event-data() -> ()  [unwired: 1 in, 6 out]
        n1090 = call <vilib>:"Application Directory.vi"() -> ("Application Directory"=w1308:path)
        n1091 = Build Path(base path=w1308, name or relative path="data\\Set.ini" ("名称或相对路径")) -> (appended path=w1309:path)
        n1092 = local read "每周自动重发"() -> (w1300:bool)
        n1093 = call <vilib>:"Open Config Data.vi"("configuration file path"=w1309) -> ("error out"=w1305:errorcluster, "refnum"=w1306:T8)  [unwired: 8 in, 1 out]
        n1094 = call-poly <vilib>:"Write Key.vi"("section"="线程一数据重发功能", "error in (no error)"=w1305, "value"=w1300, "key"="重发功能", "refnum"=w1306) -> ("error out"=w1303:errorcluster, "refnum out"=w1304:T8)  [unwired: 4 in, 1 out]
        n1095 = call <vilib>:"Close Config Data.vi"("error in (no error)"=w1303, "refnum"=w1304) -> ()  [unwired: 8 in, 2 out]
      }
      event "重发日期": Value Change {
        n1096 = event-data() -> ()  [unwired: 1 in, 6 out]
        n1097 = call <vilib>:"Application Directory.vi"() -> ("Application Directory"=w1318:path)
        n1098 = Build Path(base path=w1318, name or relative path="data\\Set.ini" ("名称或相对路径")) -> (appended path=w1319:path)
        n1099 = local read "重发日期"() -> (w1310:T2)
        n1100 = call <vilib>:"Open Config Data.vi"("configuration file path"=w1319) -> ("error out"=w1315:errorcluster, "refnum"=w1316:T8)  [unwired: 8 in, 1 out]
        n1101 = call-poly <vilib>:"Write Key.vi"("section"="线程一数据重发功能", "error in (no error)"=w1315, "value"=w1310, "key"="重发日期", "refnum"=w1316) -> ("error out"=w1313:errorcluster, "refnum out"=w1314:T8)  [unwired: 4 in, 1 out]
        n1102 = call <vilib>:"Close Config Data.vi"("error in (no error)"=w1313, "refnum"=w1314) -> ()  [unwired: 8 in, 2 out]
      }
      event "重发时间": Value Change {
        n1103 = event-data() -> ()  [unwired: 1 in, 6 out]
        n1104 = call <vilib>:"Application Directory.vi"() -> ("Application Directory"=w1328:path)
        n1105 = Build Path(base path=w1328, name or relative path="data\\Set.ini" ("名称或相对路径")) -> (appended path=w1329:path)
        n1106 = local read "重发时间"() -> (w1320:T1)
        n1107 = call <vilib>:"Open Config Data.vi"("configuration file path"=w1329) -> ("error out"=w1325:errorcluster, "refnum"=w1326:T8)  [unwired: 8 in, 1 out]
        n1108 = call-poly <vilib>:"Write Key.vi"("section"="线程一数据重发功能", "error in (no error)"=w1325, "value"=w1320, "key"="重发时间", "refnum"=w1326) -> ("error out"=w1323:errorcluster, "refnum out"=w1324:T8)  [unwired: 4 in, 1 out]
        n1109 = call <vilib>:"Close Config Data.vi"("error in (no error)"=w1323, "refnum"=w1324) -> ()  [unwired: 8 in, 2 out]
      }
      event "确定更改起始时间": Value Change {
        n1110 = event-data() -> ()  [unwired: 1 in, 6 out]
        n1111 = local write "更改起始时间"(FALSE ("更改起始时间")) -> ()
        n1112 = Two Button Dialog(message="确定以当前设置时间作为数据索引起始时间？" ("消息")) -> (T button?=w1331:bool)  [unwired: 2 in]
        n1113 = case shown="真" w1331 {
          frame False {
          }
          frame True {
            n1114 = local read "参数数值"() -> (w1333:T5)
            n1115 = Cluster To Array(cluster=w1333) -> (array=w1334:bool[])
            n1116 = for {
              tunnel: w1334 -> [_] mode=indexing
              i -> [w1335]
              n1117 = Format Date/Time String(time format string (%c)="%Y/%m/%d %H:%M:%S" ("时间格式字符串(%c)"), seconds (now)="数据发送起始时间") -> (date/time string=w1336:string)  [unwired: 1 in]
              n1118 = case shown="0, 默认" w1335 {
                tunnel: w1336 -> [w1339 w1340 w1341 w1342 w1343 w1344 w1345 w1346 w1347 w1348 w1349 w1350 w1351 w1352 w1353 w1354 w1355 w1356]
                frame 0, Default {
                  n1119 = global write "全局 水样时间.vi" "time1"(w1339) -> ()
                }
                frame 1 {
                  n1120 = global write "全局 水样时间.vi" "time2"(w1340) -> ()
                }
                frame 2 {
                  n1121 = global write "全局 水样时间.vi" "time3"(w1341) -> ()
                }
                frame 3 {
                  n1122 = global write "全局 水样时间.vi" "time4"(w1342) -> ()
                }
                frame 4 {
                  n1123 = global write "全局 水样时间.vi" "time5"(w1343) -> ()
                }
                frame 5 {
                  n1124 = global write "全局 水样时间.vi" "time6"(w1344) -> ()
                }
                frame 6 {
                  n1125 = global write "全局 水样时间.vi" "time7"(w1345) -> ()
                }
                frame 7 {
                  n1126 = global write "全局 水样时间.vi" "time8"(w1346) -> ()
                }
                frame 8 {
                  n1127 = global write "全局 水样时间.vi" "time9"(w1347) -> ()
                }
                frame 9 {
                  n1128 = global write "全局 水样时间.vi" "time10"(w1348) -> ()
                }
                frame 10 {
                  n1129 = global write "全局 水样时间.vi" "time11"(w1349) -> ()
                }
                frame 11 {
                  n1130 = global write "全局 水样时间.vi" "time12"(w1350) -> ()
                }
                frame 12 {
                  n1131 = global write "全局 水样时间.vi" "time13"(w1351) -> ()
                }
                frame 13 {
                  n1132 = global write "全局 水样时间.vi" "time14"(w1352) -> ()
                }
                frame 14 {
                  n1133 = global write "全局 水样时间.vi" "time15"(w1353) -> ()
                }
                frame 15 {
                  n1134 = global write "全局 水样时间.vi" "time16"(w1354) -> ()
                }
                frame 16 {
                  n1135 = global write "全局 水样时间.vi" "time17"(w1355) -> ()
                }
                frame 17 {
                  n1136 = global write "全局 水样时间.vi" "time18"(w1356) -> ()
                }
              }
            }
          }
        }
      }
      event "开机启动": Value Change {
        n1137 = event-data() -> ("NewVal"=w1357:bool)  [unwired: 1 in, 5 out]
        n1138 = case shown="假" w1357 {
          frame False {
            n1139 = Two Button Dialog(message="是否删除开机启动" ("消息"), 1:"否" ("F按钮名称（“取消”）"), 2:"是" ("T按钮名称（“确定”）")) -> (T button?=w1358:bool)
            n1140 = case shown="真" w1358 {
              frame False {
              }
              frame True {
                n1141 = call <vilib>:"Application Directory.vi"() -> ("Application Directory"=w1363:path)
                n1142 = call "删除启动项.vi"("启动文件路径"=w1363) -> ("删除标记"=w1362:bool)  [unwired: 9 in, 1 out]
                n1143 = case shown="假" w1362 {
                  tunnel: ["删除开机启动失败" ("T按钮名称（“确定”）") "删除开机启动成功" ("T按钮名称（“确定”）")] -> w1364
                  frame False {
                  }
                  frame True {
                  }
                }
                n1144 = One Button Dialog(message=w1364) -> ()  [unwired: 1 in, 1 out]
              }
            }
          }
          frame True {
            n1145 = Two Button Dialog(message="是否添加开机启动" ("消息"), 1:"否" ("F按钮名称（“取消”）"), 2:"是" ("T按钮名称（“确定”）")) -> (T button?=w1367:bool)
            n1146 = case shown="真" w1367 {
              frame False {
              }
              frame True {
                n1147 = call <vilib>:"Application Directory.vi"() -> ("Application Directory"=w1373:path)
                n1148 = call "添加启动项.vi"("启动文件路径"=w1373) -> ("添加成功标记"=w1372:bool)  [unwired: 9 in, 1 out]
                n1149 = case shown="真" w1372 {
                  tunnel: ["添加开机启动失败" ("T按钮名称（“确定”）") "添加开机启动成功" ("T按钮名称（“确定”）")] -> w1371
                  frame False {
                  }
                  frame True {
                  }
                }
                n1150 = One Button Dialog(message=w1371) -> ()  [unwired: 1 in, 1 out]
              }
            }
          }
        }
      }
      event "IP": Mouse Down {
        n1151 = event-data() -> ("CtlRef"=w1376:refnum<vi>)  [unwired: 1 in, 5 out]
        n1152 = property class="Str" props=["Value"](reference=w1376) -> ()  [unwired: 1 in, 3 out]
        n1153 = local read "IP"() -> (w1378:string)
        n1154 = call "IP键盘.vi"("OldNumber"=w1378) -> ("NewNumber"=w1377:string)
        n1155 = local write "IP"(w1377) -> ()
      }
      event "PORT": Mouse Down {
        n1156 = event-data() -> ()  [unwired: 1 in, 6 out]
        n1157 = local read "PORT"() -> (w1380:string)
        n1158 = call "IP键盘.vi"("OldNumber"=w1380) -> ("NewNumber"=w1379:string)
        n1159 = local write "PORT"(w1379) -> ()
      }
      event "查询质控数据起始时间": Value Change {
        n1160 = event-data() -> ()  [unwired: 1 in, 6 out]
        n1161 = property on="窗格" class="Pane"("Origin"=T11 {"Horizontal"=1000, "Vertical"=0} ("原点")) -> ()  [unwired: 2 in, 2 out]
      }
      event "返回主界面": Value Change {
        n1162 = event-data() -> ()  [unwired: 1 in, 6 out]
        n1163 = property on="窗格" class="Pane"("Origin"=T11 {"Horizontal"=0, "Vertical"=0} ("原点")) -> ()  [unwired: 2 in, 2 out]
      }
    }
  }
  n1164 = while {
    stop <- FALSE stop-if-true
    # "心跳包"
    n1165 = local read "实时小时数据上传"() -> (w1426:bool)
    n1166 = global read "全局 数据发送重叠.vi" "掉线指示灯"() -> (→"掉线指示":bool)
    n1167 = Get Date/Time In Seconds() -> (seconds since 1Jan1904=w1417:timestamp)
    n1168 = local read "数据发送通道"() -> (w1391:enum16{"TCP", "VISA"})
    n1169 = local read "空闲时间"() -> (w1409:dbl)
    n1170 = case shown="\"VISA\"" "数据发送通道" {
      tunnel: [w1449 w1452] -> w1395
      tunnel: [w1448 w1450] -> w1394
      frame "TCP", Default {
        n1171 = local read "PORT"() -> (w1448:string)
        n1172 = local read "IP"() -> (w1449:string)
      }
      frame "VISA" {
        n1173 = local read "baud rate"() -> (w1451:u32)
        n1174 = local read "VISA resource name"() -> (w1452:refnum<visa-resource-name>)
        n1175 = Number To Decimal String(number=w1451) -> (decimal integer string=w1450:string)  [unwired: 1 in]
      }
    }
    n1176 = Wait (ms)(milliseconds to wait=u32 1000 ("等待时间（毫秒）")) -> ()  [unwired: 1 out]
    n1177 = local read "实时小时数据上传"() -> (w1406:bool)
    n1178 = local read "核查数据上传"() -> (w1403:bool)
    n1179 = local read "空闲时间"() -> (w1441:dbl)
    n1180 = local read "查询数据发送"() -> (w1407:bool)
    n1181 = Number To Decimal String(number=w1409) -> (decimal integer string=→"空闲时间/s":string)  [unwired: 1 in]
    n1182 = local read "站点设备"() -> (w1396:string)
    n1183 = local read "站点名称"() -> (w1397:string)
    n1184 = global read "全局 数据发送重叠.vi" "数据接收超时指示灯"() -> (→"数据接收超时指示灯":bool)
    n1185 = global write "全局 数据发送重叠.vi" "主动上报数据中"(w1426) -> ()
    n1186 = local read "MN"() -> (w1393:string)
    n1187 = Format Date/Time String(time format string (%c)="%Y/%m/%d %H:%M:%S" ("时间格式字符串(%c)"), seconds (now)=w1417) -> (date/time string=→"系统时间":string)  [unwired: 1 in]
    n1188 = local read "PW"() -> (w1392:string)
    n1189 = local read "步骤"() -> (w1435:T6)
    n1190 = case shown="\"TCP\", 默认" w1391 {
      frame "TCP", Default {
        w1453 = TRUE ("可见")
        w1454 = FALSE ("可见")
        n1191 = property on="VISA resource name" class="VISAName"("Visible"=w1454) -> ()  [unwired: 2 in, 2 out]
        n1192 = property on="baud rate" class="DigNum (严格)"("Visible"=w1454) -> ()  [unwired: 2 in, 2 out]
        n1193 = property on="IP" class="Str"("Visible"=w1453) -> ()  [unwired: 2 in, 2 out]
        n1194 = property on="PORT" class="Str"("Visible"=w1453) -> ()  [unwired: 2 in, 2 out]
      }
      frame "VISA" {
        w1455 = TRUE ("可见")
        w1456 = FALSE ("可见")
        n1195 = property on="baud rate" class="DigNum (严格)"("Visible"=w1455) -> ()  [unwired: 2 in, 2 out]
        n1196 = property on="VISA resource name" class="VISAName"("Visible"=w1455) -> ()  [unwired: 2 in, 2 out]
        n1197 = property on="IP" class="Str"("Visible"=w1456) -> ()  [unwired: 2 in, 2 out]
        n1198 = property on="PORT" class="Str"("Visible"=w1456) -> ()  [unwired: 2 in, 2 out]
      }
    }
    n1199 = local read "数据发送协议"() -> (w1387:enum16{"2005-212协议", "2017-212协议"})
    n1200 = Not(x=w1403) -> (.not. x?=w1404:bool)
    n1201 = Greater?(x=w1441, y=30.0) -> (0:w1439:bool)
    n1202 = Not(x=w1406) -> (.not. x?=w1405:bool)
    n1203 = property on="数据发送通道" class="Enum (严格)"("Visible"="锁") -> ()  [unwired: 2 in, 2 out]
    n1204 = Not(x=w1407) -> (.not. x?=w1429:bool)
    n1205 = Equal?(x=w1435, y=T6."读取数据" ("步骤")) -> (x = y?=w1433:bool)
    n1206 = Bundle By Name(cluster=T4 {"站点"="", "设备"="", "IP"="", "PORT"="", "MN"="", "PW"=""} ("配置信息"), "站点"=w1397, "设备"=w1396, "IP"=w1395, "PORT"=w1394, "MN"=w1393, "PW"=w1392) -> (→"配置信息":T4)
    n1207 = Select(t=T12."Enabled" ("禁用"), s="更改起始时间", f=T12."Disabled and Grayed Out" ("禁用")) -> (s? t:f=w1420:T12)
    n1208 = case shown="真" w1439 {
      tunnel: w1439 -> [_ w1466]
      tunnel: [FALSE w1466] -> w1436
      frame False {
      }
      frame True {
        n1209 = local read "QN"() -> (w1464:string)
        n1210 = local write "空闲时间"(0.0 ("空闲时间")) -> ()
        n1211 = local read "MN"() -> (w1463:string)
        n1212 = local read "PW"() -> (w1462:string)
        n1213 = local read "数据发送通道"() -> (w1461:enum16{"TCP", "VISA"})
        n1214 = call "数据编码.vi"("table输入"="心跳包", "QN"=w1464, "MN"=w1463, "PW"=w1462) -> ("通讯包字符串"=w1459:string)  [unwired: 10 in, 1 out]
        n1215 = local write "发送报文显示"(w1459) -> ()
        n1216 = call "VISATCP组合选择发送.vi"("数据发送通道"=w1461, "命令"="write", "写入缓冲区"=w1459) -> ("错误输出"=w1458:errorcluster)  [unwired: 9 in, 3 out]
        n1217 = call <vilib>:"Clear Errors.vi"("error in (no error)"=w1458) -> ()  [unwired: 5 in, 2 out]
      }
    }
    "心跳包" <- w1436
    n1218 = Select(t=T12."Enabled" ("禁用"), s="锁", f=T12."Disabled and Grayed Out" ("禁用")) -> (s? t:f=w1388:T12)
    n1219 = property on="数据发送起始时间" class="AbsTime (严格)"("DisabledEnum"=w1420) -> ()  [unwired: 2 in, 2 out]
    n1220 = global read "全局 时间2.vi" "跨度核查索引起始时间"() -> (→"跨度核查索引起始时间":string)
    n1221 = case shown="\"2005-212协议\"" w1387 {
      tunnel: ["32" ("设备编码MN") w1443] -> w1427
      frame "2005-212协议" {
      }
      frame "2017-212协议", Default {
        n1222 = local read "系统编码选择框"() -> (w1444:string)
        n1223 = case shown="\"地表水体污染源\"" w1444 {
          tunnel: ["52" ("设备编码MN") "32" ("设备编码MN") "21" ("设备编码MN")] -> w1443
          frame "污水排放过程监测" {
          }
          frame "地表水体污染源" {
          }
          frame "地表水质量监测", Default {
          }
        }
      }
    }
    n1224 = global read "全局 时间2.vi" "标样核查索引起始时间"() -> (→"标样核查索引起始时间":string)
    n1225 = global read "全局 时间2.vi" "零点核查索引起始时间"() -> (→"零点核查索引起始时间":string)
    n1226 = global read "全局 时间2.vi" "加标回收索引起始时间"() -> (→"加标回收索引起始时间":string)
    n1227 = property on="设置超时时间/min" class="DigNum (严格)"("DisabledEnum"=w1388) -> ()  [unwired: 2 in, 2 out]
    n1228 = property on="IP" class="Str"("DisabledEnum"=w1388) -> ()  [unwired: 2 in, 2 out]
    n1229 = property on="每周自动重发" class="Bool (严格)"("DisabledEnum"=w1388) -> ()  [unwired: 2 in, 2 out]
    n1230 = property on="PORT" class="Str"("DisabledEnum"=w1388) -> ()  [unwired: 2 in, 2 out]
    n1231 = local read "数据发送协议"() -> (w1386:enum16{"2005-212协议", "2017-212协议"})
    n1232 = local read "TCP服务端掉线计数"() -> (w1412:i32)
    n1233 = local read "1st Error to Convert"() -> (w1415:i32)
    n1234 = local read "TCP掉线时间节点"() -> (w1411:string)
    n1235 = property on="确定更改起始时间" class="Bool"("DisabledEnum"=w1420) -> ()  [unwired: 2 in, 2 out]
    n1236 = property on="MN" class="Str"("DisabledEnum"=w1388) -> ()  [unwired: 2 in, 2 out]
    n1237 = property on="PW" class="Str"("DisabledEnum"=w1388) -> ()  [unwired: 2 in, 2 out]
    n1238 = property on="实时数据发送时间间隔/min" class="DigNum (严格)"("DisabledEnum"=w1388) -> ()  [unwired: 2 in, 2 out]
    n1239 = local read "元素"() -> (w1413:string)
    n1240 = local read "步骤"() -> (w1414:T6)
    n1241 = Equal?(x=w1386, y=enum16{"2005-212协议", "2017-212协议"}."2017-212协议" ("数据发送协议")) -> (x = y?=w1384:bool)
    n1242 = Compound Arithmetic op=AND ("复合运算")(w1384, w1433, w1429, w1405, w1404) -> (w1430:bool)
    n1243 = case shown="真" w1430 {
      frame False {
        n1244 = local write "空闲时间"(0.0 ("空闲时间")) -> ()
      }
      frame True {
        n1245 = local read "空闲时间"() -> (w1470:dbl)
        n1246 = Increment(x=w1470) -> (x+1=→"空闲时间":dbl)
      }
    }
    n1247 = property on="数据发送通道" class="Enum (严格)"("DisabledEnum"=w1388) -> ()  [unwired: 2 in, 2 out]
    n1248 = Bundle By Name(cluster=T3 {"1st Error to Convert "=54, "步骤 "=enum."打开连接", "元素"="实时数据", "TCP服务端掉线计数"=4, "TCP掉线时间节点"="2019/05/08 15:24:17"} ("状态信息"), "1st Error to Convert"=w1415, "步骤"=w1414, "元素"=w1413, "TCP服务端掉线计数"=w1412, "TCP掉线时间节点"=w1411) -> (→"状态信息":T3)
    n1249 = local read "数据发送协议"() -> (w1383:enum16{"2005-212协议", "2017-212协议"})
    n1250 = property on="重发时间" class="Enum (严格)"("DisabledEnum"=w1388) -> ()  [unwired: 2 in, 2 out]
    n1251 = property on="重发日期" class="Enum (严格)"("DisabledEnum"=w1388) -> ()  [unwired: 2 in, 2 out]
    n1252 = property on="VISA resource name" class="VISAName"("DisabledEnum"=w1388) -> ()  [unwired: 2 in, 2 out]
    n1253 = property on="baud rate" class="DigNum (严格)"("DisabledEnum"=w1388) -> ()  [unwired: 2 in, 2 out]
    n1254 = property on="数据发送协议" class="Enum (严格)"("DisabledEnum"=w1388) -> ()  [unwired: 2 in, 2 out]
    n1255 = global write "全局1.vi" "数据发送版本"(w1383) -> ()
    n1256 = global write "全局1.vi" "系统编码ST"(w1427) -> ()
  }
  n1257 = for {
    N: 1 -> [_]
    w1476 = "数据发送协议"
    w1483 = "线程一自主部署站点保存"
    w1499 = "数据发送通道" ("section")
    (unwired) path "C:/LabVIEW Project/builds/平台数据发送系统" ("Application Directory")
    w1550 = "" ("参数")
    w1511 = FALSE ("数据发送中断")
    w1521 = 0 ("数值")
    # "版本改动:增加了远程反控命令，和仪器端双向通讯，modbus TCP读写"
    # "ST参数选择"
    # "初始化"
    n1258 = property class="VI"() -> ("Panel"=w1554:refnum<vi>)  [unwired: 2 in, 2 out]
    n1259 = local write "核查数据上传"(w1511) -> ()
    n1260 = global write "全局 实时数据参数.vi" "参数"(w1550) -> ()
    n1261 = local write "心跳包"(w1511) -> ()
    n1262 = local write "查询数据发送"(w1511) -> ()
    n1263 = local write "实时小时数据上传"(w1511) -> ()
    n1264 = local write "系统状态改变"(w1511) -> ()
    n1265 = global write "全局 小时数据发送次数.vi" "小时数据发送次数"(w1521) -> ()
    n1266 = local write "重发数据"(w1511) -> ()
    n1267 = property class="Pnl"(reference=w1554) -> ("Panes[]"=w1553:refnum<vi>[])  [unwired: 1 in, 2 out]
    n1268 = global write "全局 实时数据参数.vi" "data"(string[][] [] ("data")) -> ()
    n1269 = property on="窗格" class="Pane"("Origin"=T11 {"Horizontal"=0, "Vertical"=0} ("原点")) -> ()  [unwired: 2 in, 2 out]
    n1270 = local write "空闲时间"(0.0 ("try")) -> ()
    n1271 = global write "全局1.vi" "枚举"(enum16{"返回请求应答", "上传数据", "返回执行结果"}."返回请求应答" ("枚举")) -> ()
    n1272 = global write "全局 实时数据参数.vi" "连接的字符串"(w1550) -> ()
    n1273 = call <vilib>:"Application Directory.vi"() -> ("Application Directory"=w1548:path)
    n1274 = for {
      tunnel: w1553 -> [w1564] mode=indexing
      tunnel: u32 15592941 ("窗格颜色") -> [w1565]
      n1275 = property class="Pane"(reference=w1564, "PaneColor"=w1565) -> ()  [unwired: 1 in, 2 out]
    }
    n1276 = Build Path(base path=w1548, name or relative path="data\\Set.ini" ("名称或相对路径")) -> (appended path=w1546:path)
    n1277 = call <vilib>:"Open Config Data.vi"("configuration file path"=w1546) -> ("error out"=w1544:errorcluster, "refnum"=w1545:T8)  [unwired: 8 in, 1 out]
    n1278 = call <vilib>:"Application Directory.vi"() -> ("Application Directory"=w1510:path)
    n1279 = call-poly <vilib>:"Read Key.vi"("section"=w1483, "error in (no error)"=w1544, "key"="站点名称", "refnum"=w1545) -> ("error out"=w1541:errorcluster, "value"=w1497:string, "refnum out"=w1542:T8)  [unwired: 4 in, 1 out]
    n1280 = call <vilib>:"Application Directory.vi"() -> ("Application Directory"=w1506:path)
    n1281 = call <vilib>:"Recursive File List.vi"("pattern"="*.exe", "Folder Path"=w1510) -> ("All Files in Dir"=w1519:path[])  [unwired: 5 in, 4 out]
    n1282 = local write "站点名称"(w1497) -> ()
    n1283 = Build Path(base path=w1506, name or relative path="data\\background.jpg" ("名称或相对路径")) -> (appended path=w1505:path)
    n1284 = Index Array(array=w1519) -> (element=w1518:path)  [unwired: 1 in]
    n1285 = Get Date/Time In Seconds() -> (seconds since 1Jan1904=w1558:timestamp)
    n1286 = call <vilib>:"Read JPEG File.vi"("path to JPEG file"=w1505) -> ("error out"=w1503:errorcluster, "image data"=w1504:T13)  [unwired: 8 in, 1 out]
    n1287 = Format Date/Time String(time format string (%c)="%Y%m%d%H%M%S%3u" ("时间格式字符串(%c)"), seconds (now)=w1558) -> (date/time string=w1557:string)  [unwired: 1 in]
    n1288 = call-poly <vilib>:"Read Key.vi"("section"=w1483, "error in (no error)"=w1541, "key"="站点设备", "refnum"=w1542) -> ("error out"=w1538:errorcluster, "value"=w1496:string, "refnum out"=w1539:T8)  [unwired: 4 in, 1 out]
    n1289 = File/Directory Info(path=w1518) -> (last mod=w1517:timestamp)  [unwired: 1 in, 6 out]
    n1290 = call <vilib>:"FileVersionInfo.vi"("Application Path in"=w1518) -> ("error out"=w1502:errorcluster, "File Version Info"=w1514:string)  [unwired: 7 in, 2 out]
    n1291 = property on="窗格" class="Pane"("BackgroundImage"=w1504) -> ()  [unwired: 2 in, 2 out]
    n1292 = Format Date/Time String(time format string (%c)="\n%Y%m%d%H%M" ("时间格式字符串(%c)"), seconds (now)=w1517) -> (date/time string=w1513:string)  [unwired: 1 in]
    n1293 = local write "站点设备"(w1496) -> ()
    n1294 = Search and Replace String(input string=w1557, search string="." ("搜索字符串")) -> (result string=w1555:string)  [unwired: 6 in, 3 out]
    n1295 = call-poly <vilib>:"Read Key.vi"("section"=w1483, "error in (no error)"=w1538, "key"="IP", "refnum"=w1539) -> ("error out"=w1535:errorcluster, "value"=w1495:string, "refnum out"=w1536:T8)  [unwired: 4 in, 1 out]
    n1296 = Concatenate Strings("V" ("字符串"), w1514, w1513) -> (→"软件版本":string)
    n1297 = local write "QN"(w1555) -> ()
    n1298 = call <vilib>:"Simple Error Handler.vi"("error in (no error)"=w1502) -> ()  [unwired: 4 in, 5 out]
    n1299 = call <vilib>:"Simple Error Handler.vi"("error in (no error)"=w1503) -> ()  [unwired: 4 in, 5 out]
    n1300 = local write "IP"(w1495) -> ()
    n1301 = call-poly <vilib>:"Read Key.vi"("section"=w1483, "error in (no error)"=w1535, "key"="PORT", "refnum"=w1536) -> ("error out"=w1531:errorcluster, "value"=w1494:string, "refnum out"=w1532:T8)  [unwired: 4 in, 1 out]
    n1302 = call <vilib>:"Application Directory.vi"() -> ("Application Directory"=w1509:path)
    n1303 = local write "PORT"(w1494) -> ()
    n1304 = call "查询启动项.vi"("启动文件路径"=w1509) -> ("包含启动项"=w1508:bool)  [unwired: 9 in, 1 out]
    n1305 = call-poly <vilib>:"Read Key.vi"("section"=w1483, "error in (no error)"=w1531, "key"="MN", "refnum"=w1532) -> ("error out"=w1490:errorcluster, "value"=w1493:string, "refnum out"=w1491:T8)  [unwired: 4 in, 1 out]
    n1306 = local write "MN"(w1493) -> ()
    n1307 = local write "开机启动"(w1508) -> ()
    n1308 = call-poly <vilib>:"Read Key.vi"("section"=w1483, "error in (no error)"=w1490, "key"="PW", "refnum"=w1491) -> ("error out"=w1488:errorcluster, "value"=w1492:string, "refnum out"=w1489:T8)  [unwired: 4 in, 1 out]
    n1309 = local write "PW"(w1492) -> ()
    n1310 = call-poly <vilib>:"Read Key.vi"("section"=w1483, "error in (no error)"=w1488, "key"="VISA", "refnum"=w1489) -> ("error out"=w1484:errorcluster, "value"=w1486:string, "refnum out"=w1485:T8)  [unwired: 4 in, 1 out]
    n1311 = local write "VISA resource name"(w1486) -> ()
    n1312 = call-poly <vilib>:"Read Key.vi"("section"=w1483, "error in (no error)"=w1484, "key"="BAUDRATE", "refnum"=w1485) -> ("error out"=w1479:errorcluster, "value"=w1481:i32, "refnum out"=w1480:T8)  [unwired: 4 in, 1 out]
    n1313 = local write "baud rate"(w1481) -> ()
    n1314 = call-poly <vilib>:"Read Key.vi"("section"="系统编码选择", "error in (no error)"=w1479, "key"="系统编码", "refnum"=w1480) -> ("error out"=w1525:errorcluster, "value"=w1527:string, "refnum out"=w1526:T8)  [unwired: 4 in, 1 out]
    n1315 = local write "系统编码选择框"(w1527) -> ()
    n1316 = call-poly <vilib>:"Read Key.vi"("section"="掉线时间存储", "error in (no error)"=w1525, "key"="掉线时间", "refnum"=w1526) -> ("error out"=w1500:errorcluster, "value"=w1522:string, "refnum out"=w1501:T8)  [unwired: 4 in, 1 out]
    n1317 = global write "全局 数据发送重叠.vi" "TCP掉线时间节点"(w1522) -> ()
    n1318 = local write "TCP掉线时间节点"(w1522) -> ()
    n1319 = call-poly <vilib>:"Read Key.vi"("section"=w1499, "error in (no error)"=w1500, "key"=w1499, "refnum"=w1501) -> ("error out"=w1477:errorcluster, "value"=w1498:i32, "refnum out"=w1478:T8)  [unwired: 4 in, 1 out]
    n1320 = local write "数据发送通道"(w1498) -> ()
    n1321 = call-poly <vilib>:"Read Key.vi"("section"=w1476, "error in (no error)"=w1477, "key"=w1476, "refnum"=w1478) -> ("error out"=w1474:errorcluster, "value"=w1472:i32, "found?"=w1473:bool, "refnum out"=w1475:T8)  [unwired: 4 in]
    n1322 = case shown="假" w1473 {
      tunnel: w1472 -> [_ w1563]
      tunnel: [1 ("value") w1563] -> w1471
      frame False {
      }
      frame True {
      }
    }
    n1323 = local write "数据发送协议"(w1471) -> ()
    n1324 = call <vilib>:"Close Config Data.vi"("error in (no error)"=w1474, "refnum"=w1475) -> ()  [unwired: 8 in, 2 out]
    "TCP服务端掉线计数" <- w1521
  }
  n1325 = property class="App"() -> ("App.Kind"=w31:T14)  [unwired: 2 in, 2 out]
  n1326 = case shown="\"Development System\", 默认" w31 {
    tunnel: [T15."Standard" ("状态") T15."Hidden" ("状态")] -> w3
    frame "Development System", Default {
    }
    frame "Run Time System" {
    }
  }
  n1327 = call "获取需发送的数据表.vi"() -> ("error out"=w42:errorcluster, "tables"=w51:string[])  [unwired: 10 in]
  n1328 = call <vilib>:"Clear Errors.vi"("error in (no error)"=w42) -> ()  [unwired: 5 in, 2 out]
  n1329 = call <vilib>:"Application Directory.vi"() -> ("Application Directory"=w25:path)
  n1330 = Build Path(base path=w25, name or relative path="data\\tubiao.ico" ("名称或相对路径")) -> (appended path=w15:path)
  n1331 = Insert Into Array(array=w51, index=0 ("索引"), new element="实时数据" ("新元素/子数组")) -> (w52:string[])
  n1332 = Current VI's Path() -> (path=w28:path)
  n1333 = Build Array(w15) -> (w20:path[])
  n1334 = Open VI Reference(vi path=w28) -> (vi reference=w29:refnum<vi>)  [unwired: 5 in, 1 out]
  n1335 = Array Size(array=w52) -> (size(s)=w49:i32)
  n1336 = invoke class="VI" method="FP.Open"(reference=w29, "Activate"=TRUE ("激活？"), "State"=w3) -> (error out=w30:errorcluster)  [unwired: 2 in, 4 out]
  n1337 = call <vilib>:"Constructor.vi"("error in"=w30, "IconFilePathList"=w20) -> ("error out"=w16:errorcluster, "NotifyIcon"=w24:refnum<class "NotifyIcon.lvclass">)  [unwired: 8 in]
  n1338 = Obtain Queue(name (unnamed)="STEP" ("名称（未命名）"), element data type=T6."初始化" ("枚举")) -> (queue out=w47:refnum<queue>)  [unwired: 3 in, 2 out]
  n1339 = for {
    shift-right: [w1572] -> w1
    shift-left: w16 -> [w1573]
    tunnel: string[] ["Open线程一", "-", "Exit线程一"] -> [w1571] mode=indexing
    tunnel: w23 -> [w1570] mode=indexing
    shift-right: [w1568] -> w2
    shift-left: w24 -> [w1569]
    # "2."
    n1340 = call <vilib>:"InsertMenuItem.vi"("error in"=w1573, "ItemTag"=w1570, "ItemName"=w1571, "NotifyIcon in"=w1569) -> ("error out"=w1572:errorcluster, "NotifyIcon out"=w1568:refnum<class "NotifyIcon.lvclass">)  [unwired: 6 in]
  }
  n1341 = Index Array(array=w23) -> (element=w22:string)  [unwired: 1 in]
  n1342 = Enqueue Element(queue=w47, element=T6."初始化" ("元素")) -> (queue out=w55:refnum<queue>)  [unwired: 2 in, 2 out]
  "主队列输出" <- w55
  n1343 = property class="NotifyIcon"(reference=w2, error in=w1, "Public:Visible"=TRUE ("Visible"), "Public:DefaultMenuItem"=w22, "Public:TipText"="平台发送系统线程一" ("TipText")) -> (reference out=w7:refnum<class "NotifyIcon.lvclass">, error out=w17:errorcluster, "Public:SelectedItemEvent"=w18:refnum<user-event>)
  n1344 = while {
    shift-right: [w1574] -> _
    shift-left: errorcluster {"status"=FALSE, "code"=0, "source"=""} ("error out") -> [w1586]
    shift-right: [w1583] -> _
    shift-left: _ -> [w1582]
    tunnel: w55 -> [w1585]
    tunnel: w52 -> [w1581]
    shift-right: [w1579] -> _
    shift-left: 0 ("索引") -> [w1580]
    tunnel: w49 -> [w1578]
    shift-right: [w1576] -> _
    shift-left: 0 ("索引") -> [w1577]
    stop <- FALSE stop-if-true
    n1345 = Wait (ms)(milliseconds to wait=u32 300 ("等待时间（毫秒）")) -> ()  [unwired: 1 out]
    n1346 = case shown="无错误" w1586 {
      selector: w1586 -> [w1604 w2320]
      tunnel: [w1587 w2323] -> w1574
      tunnel: w1585 -> [w1603 w2318]
      tunnel: [w1588 w2322] -> w1583
      tunnel: w1582 -> [w1600 w2322]
      tunnel: w1581 -> [w1599 _]
      tunnel: w1580 -> [w1594 w2321]
      tunnel: [w1597 w2321] -> w1579
      tunnel: w1578 -> [w1596 _]
      tunnel: w1577 -> [w1591 w2317]
      tunnel: [w1590 w2317] -> w1576
      frame No Error {
        n1347 = Less?(x=w1594, y=w1596) -> (x < y?=w1595:bool)
        n1348 = Dequeue Element(queue=w1603) -> (queue out=w1601:refnum<queue>, element=w1602:T6)  [unwired: 2 in, 2 out]
        "步骤" <- w1602
        n1349 = Select(t=w1594, s=w1595, f=0) -> (s? t:f=w1593:i32)
        n1350 = local read "元素"() -> (w1589:string)
        n1351 = Index Array(array=w1599, index=w1593) -> (element=→"元素":string)
        n1352 = case shown="\"读取数据\"" w1602 {
          tunnel: w1604 -> [w1611 _ w1636 w1776 w2234 w2314]
          tunnel: w1601 -> [w1607 w1625 w1631 w1791 w2232 w2312]
          tunnel: [w1611 w1613 w1636 w1774 w2231 w2314] -> w1587
          tunnel: [string[] [] ("待发送第一条数据") w1627 w1630 w1812 w2235 _] -> w1588
          tunnel: w1600 -> [_ w1627 _ w1812 w2235 w2313]
          tunnel: w1589 -> [_ _ _ _ _ w2307]
          tunnel: w1593 -> [w1608 w1624 w1635 w1813 w2236 w2303]
          tunnel: [w1608 w1624 w1634 w1813 w2236 w2304] -> w1597
          tunnel: w1591 -> [w1605 w1622 w1633 _ w2227 w2301]
          tunnel: [w1605 w1622 w1633 0 ("索引") w2230 w2301] -> w1590
          frame "初始化", Default {
            n1353 = Enqueue Element(queue=w1607, element=T6."打开连接" ("元素"), timeout in ms (-1)=1000 ("超时毫秒(-1)")) -> ()  [unwired: 1 in, 3 out]
          }
          frame "打开连接" {
            (unwired) "47.98.43.76"
            # "和时通数据接入平台端接收IP端口号，61.191.22.195:10003。"
            # "47.98.43.76:6666"
            n1354 = Enqueue Element(queue=w1625, element=T6."表格比对" ("元素"), timeout in ms (-1)=1000 ("超时毫秒(-1)")) -> ()  [unwired: 1 in, 3 out]
            n1355 = local read "数据发送通道"() -> (w1612:enum16{"TCP", "VISA"})
            n1356 = call "VISATCP组合选择发送.vi"("IP"="IP", "数据发送通道"=w1612, "命令"="open", "PORT"="PORT", "VISA resource name"="VISA resource name", "baud rate"="baud rate") -> ("错误输出"=w1613:errorcluster)  [unwired: 6 in, 3 out]
            n1357 = Unbundle By Name(w1613) -> ("status"=w1621:bool, "code"=→"1st Error to Convert":i32)
            n1358 = Not(x=w1621) -> (.not. x?=→"通信状态":bool)
          }
          frame "表格比对" {
            # "在发送数据完之后通过TCP掉线计数仍然大于1且列队中还有元素判定再次回到表格对比\n再在表格对比这里加上出列队（前提先一次把水样测试、核查等5个元素入列队）...........LOOP直到5种测量数据全部发送完毕"
            n1359 = disable-structure shown="禁用" {
              disable-tunnel: [w1638 _] -> _
              frame Disabled {
                n1360 = local read "TCP服务端掉线计数"() -> (w1640:i32)
                n1361 = Greater Or Equal?(x=w1640, y=1) -> (x >= y?=w1637:bool)
                n1362 = case shown="真" w1637 {
                  tunnel: [T6."读取数据" ("元素") w1642] -> w1638
                  frame False {
                  }
                  frame True {
                    n1363 = local read "重发数据"() -> (w1643:bool)
                    n1364 = Obtain Queue(name (unnamed)="重发掉线数据" ("名称（未命名）"), element data type=T16."水样测试") -> (queue out=w1649:refnum<queue>, error out=w1646:errorcluster)  [unwired: 3 in, 1 out]
                    n1365 = case shown="假" w1643 {
                      tunnel: w1649 -> [w1655 w1662]
                      tunnel: [w1653 w1662] -> w1647
                      tunnel: w1646 -> [w1652 w1661]
                      tunnel: [w1651 w1661] -> w1645
                      frame False {
                        n1366 = for {
                          N: 8 -> [_]
                          tunnel: w1655 -> [w1660]
                          tunnel: [w1658] -> w1653
                          tunnel: w1652 -> [w1657]
                          tunnel: [w1656] -> w1651
                          i -> [w1659]
                          n1367 = Enqueue Element(queue=w1660, element=w1659, error in (no error)=w1657) -> (queue out=w1658:refnum<queue>, error out=w1656:errorcluster)  [unwired: 1 in, 1 out]
                        }
                      }
                      frame True {
                      }
                    }
                    n1368 = Dequeue Element(queue=w1647, error in (no error)=w1645) -> (element=w1644:T16)  [unwired: 1 in, 3 out]
                    n1369 = case shown="\"加标回收\"" w1644 {
                      tunnel: [w1663 w1678 w1692 w1702 w1712 w1725 w1738 w1751] -> w1642
                      frame "水样测试", Default {
                        n1370 = flat-sequence {
                          tunnel: [w1671] -> w1663
                          frame #0 {
                            n1371 = global write "全局 小时数据发送次数.vi" "小时数据发送次数"(0 ("数值")) -> ()
                            n1372 = global write "全局 实时数据参数.vi" "实时数据参数"("水样测试") -> ()
                            n1373 = local write "table元素"("提取实时数据" ("新元素/子数组")) -> ()
                            n1374 = global write "全局1.vi" "枚举"(enum16{"返回请求应答", "上传数据", "返回执行结果"}."上传数据" ("枚举")) -> ()
                          }
                          frame #1 {
                            n1375 = call "从数据库获取数据通用可配置(子VI).vi"("table输入"="实时数据" ("新元素/子数组"), "列队名（唯一）"="adiao") -> ()  [unwired: 8 in, 2 out]
                          }
                          frame #2 {
                            # "数据处理整合"
                            n1376 = call "数据处理整合 (子VI).vi"("枚举"=enum16{"实时数据排序", "小时数据排序"}."实时数据排序") -> ("已排序的数组"=w1675:string[])  [unwired: 10 in]
                            n1377 = Array Size(array=w1675) -> (size(s)=w1674:i32)
                            n1378 = global write "全局 数据数组大小.vi" "数据数组大小"(w1674) -> ()
                            n1379 = Greater Than 0?(x=w1674) -> (x > 0?=w1673:bool)
                            n1380 = case shown="真" w1673 {
                              tunnel: [T6."表格比对" ("元素") T6."发送数据" ("元素")] -> w1671
                              frame False {
                              }
                              frame True {
                              }
                            }
                            "重发数据" <- TRUE ("重发数据中")
                          }
                        }
                      }
                      frame "小时数据" {
                        n1381 = flat-sequence {
                          tunnel: [w1686] -> w1678
                          frame #0 {
                            n1382 = local read "TCP掉线时间节点"() -> (w1680:string)
                            n1383 = call "当前时间格式显示 (子VI).vi"() -> ("当前时间格式显示"=w1679:string)  [unwired: 11 in]
                            n1384 = global write "全局 时间2.vi" "小时数据时间2"(w1679) -> ()
                            n1385 = global write "全局 水样时间.vi" "小时数据时间"(w1680) -> ()
                            n1386 = global write "全局 小时数据发送次数.vi" "小时数据发送次数"(0 ("数值")) -> ()
                            n1387 = local write "table元素"("小时数据" ("新元素/子数组")) -> ()
                            n1388 = global write "全局1.vi" "枚举"(enum16{"返回请求应答", "上传数据", "返回执行结果"}."返回请求应答" ("枚举")) -> ()
                          }
                          frame #1 {
                            n1389 = call "从数据库获取数据通用可配置(子VI).vi"("table输入"="小时数据" ("新元素/子数组"), "列队名（唯一）"="XS" ("名称（未命名）")) -> ()  [unwired: 8 in, 2 out]
                          }
                          frame #2 {
                            # "数据处理整合"
                            n1390 = call "数据处理整合 (子VI).vi"() -> ("已排序的数组"=w1689:string[])  [unwired: 11 in]
                            n1391 = Array Size(array=w1689) -> (size(s)=w1688:i32)
                            n1392 = global write "全局 数据数组大小.vi" "数据数组大小"(w1688) -> ()
                            n1393 = Greater Than 0?(x=w1688) -> (x > 0?=w1687:bool)
                            n1394 = case shown="真" w1687 {
                              tunnel: [T6."表格比对" ("元素") T6."发送数据" ("元素")] -> w1686
                              frame False {
                              }
                              frame True {
                              }
                            }
                          }
                        }
                      }
                      frame "日志信息" {
                        n1395 = flat-sequence {
                          tunnel: [w1696] -> w1692
                          frame #0 {
                            n1396 = global write "全局 小时数据发送次数.vi" "小时数据发送次数"(0 ("数值")) -> ()
                            n1397 = global write "全局1.vi" "枚举"(enum16{"返回请求应答", "上传数据", "返回执行结果"}."上传数据" ("枚举")) -> ()
                            n1398 = local write "table元素"("操作日志" ("新元素/子数组")) -> ()
                          }
                          frame #1 {
                            n1399 = call "获取操作日志 (子VI).vi"() -> ()  [unwired: 12 in]
                          }
                          frame #2 {
                            # "数据处理整合"
                            n1400 = call "数据处理整合 (子VI).vi"() -> ("已排序的数组"=w1699:string[])  [unwired: 11 in]
                            n1401 = Array Size(array=w1699) -> (size(s)=w1698:i32)
                            n1402 = global write "全局 数据数组大小.vi" "数据数组大小"(w1698) -> ()
                            n1403 = Greater Than 0?(x=w1698) -> (x > 0?=w1697:bool)
                            n1404 = case shown="假" w1697 {
                              tunnel: [T6."表格比对" ("元素") T6."发送数据" ("元素")] -> w1696
                              frame False {
                              }
                              frame True {
                              }
                            }
                          }
                        }
                      }
                      frame "报警信息" {
                        n1405 = flat-sequence {
                          tunnel: [w1706] -> w1702
                          frame #0 {
                            n1406 = global write "全局 小时数据发送次数.vi" "小时数据发送次数"(0 ("数值")) -> ()
                            n1407 = global write "全局1.vi" "枚举"(enum16{"返回请求应答", "上传数据", "返回执行结果"}."上传数据" ("枚举")) -> ()
                            n1408 = local write "table元素"("报警信息" ("新元素/子数组")) -> ()
                          }
                          frame #1 {
                            n1409 = call "获取报警信息 (子VI).vi"() -> ()  [unwired: 12 in]
                          }
                          frame #2 {
                            # "数据处理整合"
                            n1410 = call "数据处理整合 (子VI).vi"() -> ("已排序的数组"=w1709:string[])  [unwired: 11 in]
                            n1411 = Array Size(array=w1709) -> (size(s)=w1708:i32)
                            n1412 = Greater Than 0?(x=w1708) -> (x > 0?=w1707:bool)
                            n1413 = global write "全局 数据数组大小.vi" "数据数组大小"(w1708) -> ()
                            n1414 = case shown="假" w1707 {
                              tunnel: [T6."表格比对" ("元素") T6."发送数据" ("元素")] -> w1706
                              frame False {
                              }
                              frame True {
                              }
                            }
                          }
                        }
                      }
                      frame "零点核查" {
                        n1415 = flat-sequence {
                          tunnel: [w1719] -> w1712
                          frame #0 {
                            n1416 = global write "全局 小时数据发送次数.vi" "小时数据发送次数"(0 ("数值")) -> ()
                            n1417 = global write "全局 实时数据参数.vi" "实时数据参数"("空白测试") -> ()
                            n1418 = local write "table元素"("实时数据" ("新元素/子数组")) -> ()
                            n1419 = global write "全局1.vi" "枚举"(enum16{"返回请求应答", "上传数据", "返回执行结果"}."返回请求应答" ("枚举")) -> ()
                          }
                          frame #1 {
                            n1420 = call "从数据库获取数据通用可配置(子VI).vi"("table输入"="实时数据" ("新元素/子数组"), "列队名（唯一）"="bdiao") -> ()  [unwired: 8 in, 2 out]
                          }
                          frame #2 {
                            # "数据处理整合"
                            n1421 = call "数据处理整合 (子VI).vi"() -> ("已排序的数组"=w1722:string[])  [unwired: 11 in]
                            n1422 = Array Size(array=w1722) -> (size(s)=w1721:i32)
                            n1423 = global write "全局 数据数组大小.vi" "数据数组大小"(w1721) -> ()
                            n1424 = Greater Than 0?(x=w1721) -> (x > 0?=w1720:bool)
                            n1425 = case shown="假" w1720 {
                              tunnel: [T6."表格比对" ("元素") T6."发送数据" ("元素")] -> w1719
                              frame False {
                              }
                              frame True {
                              }
                            }
                          }
                        }
                      }
                      frame "标样核查" {
                        n1426 = flat-sequence {
                          tunnel: [w1732] -> w1725
                          frame #0 {
                            n1427 = global write "全局 小时数据发送次数.vi" "小时数据发送次数"(0 ("数值")) -> ()
                            n1428 = global write "全局 实时数据参数.vi" "实时数据参数"("跨度核查") -> ()
                            n1429 = global write "全局1.vi" "枚举"(enum16{"返回请求应答", "上传数据", "返回执行结果"}."返回请求应答" ("枚举")) -> ()
                            n1430 = local write "table元素"("实时数据" ("新元素/子数组")) -> ()
                          }
                          frame #1 {
                            n1431 = call "从数据库获取数据通用可配置(子VI).vi"("table输入"="实时数据" ("新元素/子数组"), "列队名（唯一）"="cdiao") -> ()  [unwired: 8 in, 2 out]
                          }
                          frame #2 {
                            # "数据处理整合"
                            n1432 = call "数据处理整合 (子VI).vi"() -> ("已排序的数组"=w1735:string[])  [unwired: 11 in]
                            n1433 = Array Size(array=w1735) -> (size(s)=w1734:i32)
                            n1434 = global write "全局 数据数组大小.vi" "数据数组大小"(w1734) -> ()
                            n1435 = Greater Than 0?(x=w1734) -> (x > 0?=w1733:bool)
                            n1436 = case shown="假" w1733 {
                              tunnel: [T6."表格比对" ("元素") T6."发送数据" ("元素")] -> w1732
                              frame False {
                              }
                              frame True {
                              }
                            }
                          }
                        }
                      }
                      frame "平行样" {
                        n1437 = flat-sequence {
                          tunnel: [w1745] -> w1738
                          frame #0 {
                            n1438 = global write "全局 小时数据发送次数.vi" "小时数据发送次数"(0 ("数值")) -> ()
                            n1439 = global write "全局 实时数据参数.vi" "实时数据参数"("平行样测试") -> ()
                            n1440 = local write "table元素"("提取实时数据" ("新元素/子数组")) -> ()
                            n1441 = global write "全局1.vi" "枚举"(enum16{"返回请求应答", "上传数据", "返回执行结果"}."上传数据" ("枚举")) -> ()
                          }
                          frame #1 {
                            n1442 = call "从数据库获取数据通用可配置(子VI).vi"("table输入"="实时数据" ("新元素/子数组"), "列队名（唯一）"="ddiao") -> ()  [unwired: 8 in, 2 out]
                          }
                          frame #2 {
                            # "数据处理整合"
                            n1443 = call "数据处理整合 (子VI).vi"() -> ("已排序的数组"=w1748:string[])  [unwired: 11 in]
                            n1444 = Array Size(array=w1748) -> (size(s)=w1747:i32)
                            n1445 = global write "全局 数据数组大小.vi" "数据数组大小"(w1747) -> ()
                            n1446 = Greater Than 0?(x=w1747) -> (x > 0?=w1746:bool)
                            n1447 = case shown="假" w1746 {
                              tunnel: [T6."表格比对" ("元素") T6."发送数据" ("元素")] -> w1745
                              frame False {
                              }
                              frame True {
                              }
                            }
                          }
                        }
                      }
                      frame "加标回收" {
                        n1448 = flat-sequence {
                          tunnel: [w1759] -> w1751
                          frame #0 {
                            n1449 = global write "全局 小时数据发送次数.vi" "小时数据发送次数"(0 ("数值")) -> ()
                            n1450 = global write "全局 实时数据参数.vi" "实时数据参数"("加标回收测试") -> ()
                            n1451 = global write "全局1.vi" "枚举"(enum16{"返回请求应答", "上传数据", "返回执行结果"}."上传数据" ("枚举")) -> ()
                            n1452 = local write "table元素"("实时数据" ("新元素/子数组")) -> ()
                          }
                          frame #1 {
                            n1453 = call "从数据库获取数据通用可配置(子VI).vi"("table输入"="加标回收" ("新元素/子数组"), "列队名（唯一）"="ediao") -> ()  [unwired: 8 in, 2 out]
                          }
                          frame #2 {
                            # "数据处理整合"
                            n1454 = call "加标回收数据处理整合 (子VI).vi"() -> ("已排序的数组"=w1758:string[])  [unwired: 11 in]
                            n1455 = Array Size(array=w1758) -> (size(s)=w1761:i32)
                            n1456 = global write "全局 数据数组大小.vi" "数据数组大小"(w1761) -> ()
                            n1457 = Greater Than 0?(x=w1761) -> (x > 0?=w1760:bool)
                            n1458 = case shown="假" w1760 {
                              tunnel: [T6."读取数据" ("元素") T6."发送数据" ("元素")] -> w1759
                              frame False {
                              }
                              frame True {
                              }
                            }
                          }
                        }
                      }
                    }
                  }
                }
              }
              frame Enabled {
              }
            }
            n1459 = disable-structure shown="启用" {
              disable-tunnel: [w1770 _] -> w1630
              frame Disabled {
                n1460 = call "数据表比对.vi"("查询元素输入"="氨氮" ("table输入 2"), "table输入"="实时数据") -> ("待发送第一条数据"=w1770:string[], "待发送数据"=w1764:string[][])  [unwired: 6 in, 2 out]
                n1461 = Empty Array?(array=w1764) -> (empty?=w1769:bool)
                n1462 = local read "心跳包"() -> (w1767:bool)
                n1463 = Not(x=w1769) -> (.not. x?=w1768:bool)
                n1464 = Or(x=w1768, y=w1767) -> ()  [unwired: 1 out]
              }
              frame Enabled {
              }
            }
            n1465 = case shown="假" FALSE {
              tunnel: w1635 -> [w1772 w1773]
              tunnel: [w1771 w1773] -> w1634
              frame False {
                n1466 = Increment(x=w1772) -> (x+1=w1771:i32)
              }
              frame True {
              }
            }
            n1467 = Enqueue Element(queue=w1631, element=T6."读取数据" ("元素"), timeout in ms (-1)=1000 ("超时毫秒(-1)")) -> ()  [unwired: 1 in, 3 out]
          }
          frame "读取数据" {
            w1787 = FALSE ("数据正在发送")
            # "设置测量时间间隔"
            # "1000设置超时时间和重发次数\n1011提取监测仪表时间\n1012设置监测仪表时间\n1014提取数采仪时间\n1015设置数采仪时间\n1061提取实时数据间隔\n1062设置实时数据间隔\n1072设置数采仪访问密码"
            # "6分钟掉线重连"
            n1468 = property on="TCP服务端掉线计数" class="DigNum (严格)"("Value"=0 ("TCP服务端掉线计数")) -> ()  [unwired: 2 in, 2 out]
            n1469 = global write "全局 数据发送重叠.vi" "掉线指示灯"(FALSE ("数据发送重叠")) -> ()
            n1470 = local write "重发数据"(w1787) -> ()
            n1471 = local write "查询数据发送"(w1787) -> ()
            n1472 = property on="实时数据发送时间间隔/min" class="DigNum (严格)"() -> ("Value"=w1799:u32)  [unwired: 2 in, 2 out]
            n1473 = global write "实时数据发送间隔全局.vi" "实时数据发送间隔"(w1799) -> ()
            n1474 = property on="设置超时时间/min" class="DigNum (严格)"() -> ("Value"=w1801:i32)  [unwired: 2 in, 2 out]
            n1475 = Multiply(x=w1801, y=10000) -> ()  [unwired: 1 out]
            n1476 = local read "数据发送通道"() -> (w1778:enum16{"TCP", "VISA"})
            n1477 = call "VISATCP组合选择发送.vi"("数据发送通道"=w1778, "命令"="read", "error in (no error)"=w1776) -> ("读取缓冲区"=w1775:string, "错误输出"=w1774:errorcluster)  [unwired: 9 in, 2 out]
            n1478 = Empty String/Path?(string/path=w1775) -> (empty?=w1784:bool)
            n1479 = case shown="假" w1784 {
              tunnel: w1775 -> [w1820 _]
              frame False {
                n1480 = call "数据记录.vi"("写入字段"=w1820) -> ("连接的字符串"=→"读取报文显示":string)  [unwired: 10 in]
                n1481 = global write "全局1.vi" "数据输出"(w1820) -> ()
                "数据输出" <- w1820
              }
              frame True {
              }
            }
            n1482 = control-ref of="数组 2"() -> (w1803:refnum<vi>)
            n1483 = control-ref of="数组"() -> (w1802:refnum<vi>)
            n1484 = call "读取数据处理 (子VI).vi"("Array输入"=w1803, "data out"=w1775, "reference"=w1802) -> ("数组"=→"数组":string[], "系统编码ST"=→"系统编码ST":string, "数组 2"=→"数组 2":string[], "命令编码CN"=w1792:string, "设备编码MN"=→"设备编码MN":string, "密码PW"=→"密码PW":string, "数据"=→"数据":string, "拆分包及应答Flag"=→"拆分包及应答Flag":string, "时间QN"=w1795:string)  [unwired: 4 in]
            "命令编码CN" <- w1792
            "时间QN" <- w1795
            n1485 = Search/Split String(string=w1795, search string/char (-)="QN=" ("搜索字符串/字符(-)")) -> (match + rest of string=w1793:string)  [unwired: 1 in, 2 out]
            n1486 = String Subset(string=w1793, offset (0)=3 ("偏移量(0)")) -> (substring=→"QN":string)  [unwired: 1 in]
            n1487 = local read "核查数据上传"() -> (w1782:bool)
            n1488 = local read "实时小时数据上传"() -> (w1783:bool)
            n1489 = Not(x=w1782) -> (.not. x?=w1780:bool)
            n1490 = Not(x=w1783) -> (.not. x?=w1781:bool)
            n1491 = And(x=w1781, y=w1780) -> (x .and. y?=w1779:bool)
            n1492 = case shown="真" w1779 {
              tunnel: w1792 -> [_ w1818]
              tunnel: ["" ("命令编码CN") w1815] -> w1785
              frame False {
              }
              frame True {
                n1493 = Search/Split String(string=w1818, search string/char (-)="CN=" ("搜索字符串/字符(-)")) -> (match + rest of string=w1816:string)  [unwired: 1 in, 2 out]
                n1494 = String Subset(string=w1816, offset (0)=3 ("偏移量(0)")) -> (substring=w1815:string)  [unwired: 1 in]
              }
            }
            n1495 = case shown="\"2061\"" w1785 {
              tunnel: w1791 -> [w1823 w1825 w1839 w1842 w1845 w1848 w1851 w1854 w1861 w1864 w1883 w1901 w1920 w1938 w1957 w1976 w1991 w2113 w2116 w2120 w2126 w2144 w2147 w2159 w2182 w2188]
              tunnel: [w1823 w1825 w1839 w1842 w1845 w1848 w1851 w1854 w1861 w1864 w1883 w1901 w1920 w1938 w1957 w1976 w1991 w2113 w2116 w2120 w2126 w2144 w2147 w2159 w2182 w2188] -> w1789
              tunnel: [T6."读取数据" ("元素") T6."发送数据" ("元素") T6."发送数据" ("元素") T6."发送数据" ("元素") T6."发送数据" ("元素") T6."发送数据" ("元素") T6."发送数据" ("元素") T6."发送数据" ("元素") T6."发送数据" ("元素") w1863 w1882 w1900 w1919 w1937 w1956 w1975 w1990 T6."发送数据" ("元素") w2115 w2119 T6."发送数据" ("元素") T6."发送数据" ("元素") T6."发送数据" ("元素") T6."发送数据" ("元素") T6."发送数据" ("元素") T6."发送数据" ("元素")] -> w1788
              tunnel: w1785 -> [_ _ _ _ _ _ _ _ _ _ _ _ _ _ _ _ _ _ _ _ _ _ _ _ _ w2186]
              frame "", Default {
              }
              frame "1000" {
                # "发回给平台"
                # "反控指令"
                # "3042~3086"
                # "1000"
                n1496 = property on="数据" class="Str"() -> ("Value"=w1831:string)  [unwired: 2 in, 2 out]
                n1497 = String Subset(string=w1831, offset (0)=9 ("偏移量(0)"), length (rest)=1 ("长度（剩余）")) -> (substring=w1828:string)
                n1498 = Decimal String To Number(string=w1828) -> (number=→"设置超时时间/min":i32)  [unwired: 2 in, 1 out]
                n1499 = local write "table元素"("反控命令" ("新元素/子数组")) -> ()
              }
              frame "1011" {
                # "1011"
                n1500 = local read "数据"() -> (w1837:string)
                n1501 = Search/Split String(string=w1837, search string/char (-)="PolId=" ("搜索字符串/字符(-)")) -> (match + rest of string=w1835:string)  [unwired: 1 in, 2 out]
                n1502 = String Subset(string=w1835, offset (0)=6 ("偏移量(0)"), length (rest)=6 ("长度（剩余）")) -> (substring=w1832:string)
                n1503 = global write "全局 提取仪器参数.vi" "仪器编码"(w1832) -> ()
                n1504 = local write "table元素"("提取监测仪表时间") -> ()
              }
              frame "1012" {
                # "设置监测仪表时间"
                n1505 = local write "table元素"("反控命令" ("新元素/子数组")) -> ()
              }
              frame "1014" {
                # "1014"
                n1506 = local write "table元素"("提取数采仪时间") -> ()
              }
              frame "1015" {
                # "设置数采仪时间"
                n1507 = local write "table元素"("反控命令" ("新元素/子数组")) -> ()
              }
              frame "1061" {
                # "1061"
                n1508 = local write "table元素"("提取实时数据间隔") -> ()
              }
              frame "1062" {
                # "发回给平台"
                # "反控指令"
                # "3042~3086"
                # "设置数据发送时间间隔"
                # "1062"
                n1509 = property on="数据" class="Str"() -> ("Value"=w1859:string)  [unwired: 2 in, 2 out]
                n1510 = String Subset(string=w1859, offset (0)=12 ("偏移量(0)")) -> (substring=w1857:string)  [unwired: 1 in]
                n1511 = Decimal String To Number(string=w1857) -> (number=w1856:i32)  [unwired: 2 in, 1 out]
                n1512 = property on="实时数据发送时间间隔/min" class="DigNum (严格)"("Value"=w1856) -> ()  [unwired: 2 in, 2 out]
                n1513 = local write "table元素"("反控命令" ("新元素/子数组")) -> ()
              }
              frame "1072" {
                # "设置数采仪密码"
                n1514 = local write "table元素"("反控命令" ("新元素/子数组")) -> ()
              }
              frame "2011" {
                w1869 = 0 ("数值")
                # "2011提取实时数据"
                n1515 = local read "数据"() -> (w1870:string)
                n1516 = String Subset(string=w1870, offset (0)=10 ("偏移量(0)"), length (rest)=14 ("长度（剩余）")) -> (substring=w1866:string)
                n1517 = String Subset(string=w1870, offset (0)=33 ("偏移量(0)"), length (rest)=14 ("长度（剩余）")) -> (substring=w1868:string)
                n1518 = call "格式时间字符串.vi"("字符串"=w1866) -> ("连接的字符串"=w1865:string)  [unwired: 10 in]
                n1519 = call "格式时间字符串.vi"("字符串"=w1868) -> ("连接的字符串"=w1867:string)  [unwired: 10 in]
                n1520 = global write "全局 小时数据发送次数.vi" "小时数据发送次数"(w1869) -> ()
                n1521 = global write "全局1.vi" "枚举"(w1869) -> ()
                n1522 = global write "起始时间.vi" "结束时间"(w1867) -> ()
                n1523 = global write "起始时间.vi" "起始时间"(w1865) -> ()
                n1524 = flat-sequence {
                  tunnel: [T6."发送数据" ("元素")] -> w1863
                  frame #0 {
                    w1875 = "提取实时数据" ("新元素/子数组")
                    n1525 = global write "全局 实时数据参数.vi" "实时数据参数"("水样测试") -> ()
                    n1526 = call "从数据库获取数据通用可配置(子VI).vi"("table输入"=w1875, "列队名（唯一）"=w1875) -> ()  [unwired: 8 in, 2 out]
                  }
                  frame #1 {
                    # "数据处理整合"
                    n1527 = local write "table元素"("提取实时数据" ("新元素/子数组")) -> ()
                    n1528 = call "数据处理整合 (子VI).vi"("枚举"=enum16{"实时数据排序", "小时数据排序"}."实时数据排序") -> ("已排序的数组"=w1878:string[])  [unwired: 10 in]
                    n1529 = Array Size(array=w1878) -> (size(s)=w1879:i32)
                    n1530 = global write "全局 数据数组大小.vi" "数据数组大小"(w1879) -> ()
                  }
                  frame #2 {
                  }
                }
              }
              frame "2061" {
                w1884 = 0 ("数值")
                n1531 = flat-sequence {
                  tunnel: [T6."发送数据" ("元素")] -> w1882
                  frame #0 {
                    # "格式时间"
                    # "2061、提取小时数据"
                    n1532 = local read "数据"() -> (w1891:string)
                    n1533 = String Subset(string=w1891, offset (0)=33 ("偏移量(0)"), length (rest)=14 ("长度（剩余）")) -> (substring=w1886:string)
                    n1534 = String Subset(string=w1891, offset (0)=10 ("偏移量(0)"), length (rest)=14 ("长度（剩余）")) -> (substring=w1887:string)
                    n1535 = call "格式时间字符串.vi"("字符串"=w1887) -> ("连接的字符串"=w1888:string)  [unwired: 10 in]
                    n1536 = call "格式时间字符串.vi"("字符串"=w1886) -> ("连接的字符串"=w1885:string)  [unwired: 10 in]
                    n1537 = global write "全局 水样时间.vi" "小时数据时间"(w1888) -> ()
                    n1538 = global write "全局 时间2.vi" "小时数据时间2"(w1885) -> ()
                  }
                  frame #1 {
                    w1894 = "小时数据" ("名称（未命名）")
                    # "提取COD、氨氮、多参数、总磷、总氮数据"
                    n1539 = call "从数据库获取数据通用可配置(子VI).vi"("table输入"=w1894, "列队名（唯一）"=w1894) -> ()  [unwired: 8 in, 2 out]
                  }
                  frame #2 {
                    # "数据处理整合"
                    n1540 = call "数据处理整合 (子VI).vi"("枚举"=enum16{"实时数据排序", "小时数据排序"}."小时数据排序") -> ("已排序的数组"=w1897:string[])  [unwired: 10 in]
                    n1541 = local write "table元素"("提取小时数据" ("新元素/子数组")) -> ()
                    n1542 = Array Size(array=w1897) -> (size(s)=w1896:i32)
                    n1543 = global write "全局 数据数组大小.vi" "数据数组大小"(w1896) -> ()
                  }
                  frame #3 {
                  }
                }
                n1544 = global write "全局 小时数据发送次数.vi" "小时数据发送次数"(w1884) -> ()
                n1545 = global write "全局1.vi" "枚举"(w1884) -> ()
              }
              frame "2062" {
                w1902 = 0 ("数值")
                n1546 = flat-sequence {
                  tunnel: [T6."发送数据" ("元素")] -> w1900
                  frame #0 {
                    # "格式时间"
                    # "2062、提取标样核查数据"
                    n1547 = local read "数据"() -> (w1909:string)
                    n1548 = String Subset(string=w1909, offset (0)=33 ("偏移量(0)"), length (rest)=14 ("长度（剩余）")) -> (substring=w1904:string)
                    n1549 = String Subset(string=w1909, offset (0)=10 ("偏移量(0)"), length (rest)=14 ("长度（剩余）")) -> (substring=w1905:string)
                    n1550 = call "格式时间字符串.vi"("字符串"=w1905) -> ("连接的字符串"=w1906:string)  [unwired: 10 in]
                    n1551 = call "格式时间字符串.vi"("字符串"=w1904) -> ("连接的字符串"=w1903:string)  [unwired: 10 in]
                    n1552 = global write "全局 水样时间.vi" "时间"(w1906) -> ()
                    n1553 = global write "全局 时间2.vi" "时间2"(w1903) -> ()
                  }
                  frame #1 {
                    # "提取COD、氨氮、多参数、总磷、总氮数据"
                    n1554 = call "从数据库获取数据通用可配置(子VI).vi"("table输入"="标样核查" ("新元素/子数组"), "列队名（唯一）"="核查数据" ("新元素/子数组")) -> ()  [unwired: 8 in, 2 out]
                  }
                  frame #2 {
                    # "数据处理整合"
                    n1555 = local write "table元素"("核查数据" ("新元素/子数组")) -> ()
                    n1556 = call "数据处理整合 (子VI).vi"("枚举"=enum16{"实时数据排序", "小时数据排序"}."实时数据排序") -> ("已排序的数组"=w1915:string[])  [unwired: 10 in]
                    n1557 = Array Size(array=w1915) -> (size(s)=w1916:i32)
                    n1558 = global write "全局 数据数组大小.vi" "数据数组大小"(w1916) -> ()
                  }
                  frame #3 {
                  }
                }
                n1559 = global write "全局 小时数据发送次数.vi" "小时数据发送次数"(w1902) -> ()
                n1560 = global write "全局1.vi" "枚举"(w1902) -> ()
              }
              frame "2063" {
                w1925 = 0 ("数值")
                # "2063提取加标回收数据"
                n1561 = local read "数据"() -> (w1926:string)
                n1562 = String Subset(string=w1926, offset (0)=10 ("偏移量(0)"), length (rest)=14 ("长度（剩余）")) -> (substring=w1922:string)
                n1563 = String Subset(string=w1926, offset (0)=33 ("偏移量(0)"), length (rest)=14 ("长度（剩余）")) -> (substring=w1924:string)
                n1564 = call "格式时间字符串.vi"("字符串"=w1922) -> ("连接的字符串"=w1921:string)  [unwired: 10 in]
                n1565 = call "格式时间字符串.vi"("字符串"=w1924) -> ("连接的字符串"=w1923:string)  [unwired: 10 in]
                n1566 = global write "全局 小时数据发送次数.vi" "小时数据发送次数"(w1925) -> ()
                n1567 = global write "全局1.vi" "枚举"(w1925) -> ()
                n1568 = global write "起始时间.vi" "结束时间"(w1923) -> ()
                n1569 = global write "起始时间.vi" "起始时间"(w1921) -> ()
                n1570 = flat-sequence {
                  tunnel: [T6."发送数据" ("元素")] -> w1919
                  frame #0 {
                    w1931 = "提取加标回收" ("新元素/子数组")
                    n1571 = call "从数据库获取数据通用可配置(子VI).vi"("table输入"=w1931, "列队名（唯一）"=w1931) -> ()  [unwired: 8 in, 2 out]
                  }
                  frame #1 {
                    n1572 = local write "table元素"("提取加标回收" ("新元素/子数组")) -> ()
                    n1573 = call "加标回收数据处理整合 (子VI).vi"("枚举"=enum16{"实时数据排序", "小时数据排序"}."实时数据排序") -> ("已排序的数组"=w1932:string[])  [unwired: 10 in]
                    n1574 = Array Size(array=w1932) -> (size(s)=w1934:i32)
                    n1575 = global write "全局 数据数组大小.vi" "数据数组大小"(w1934) -> ()
                  }
                  frame #2 {
                  }
                }
              }
              frame "2065" {
                w1939 = 0 ("数值")
                n1576 = flat-sequence {
                  tunnel: [T6."发送数据" ("元素")] -> w1937
                  frame #0 {
                    # "格式时间"
                    # "2065、提取零点核查数据"
                    n1577 = local read "数据"() -> (w1948:string)
                    n1578 = global write "全局 实时数据参数.vi" "实时数据参数"("空白测试" ("新元素/子数组")) -> ()
                    n1579 = local write "table元素"("空白测试" ("新元素/子数组")) -> ()
                    n1580 = String Subset(string=w1948, offset (0)=33 ("偏移量(0)"), length (rest)=14 ("长度（剩余）")) -> (substring=w1943:string)
                    n1581 = String Subset(string=w1948, offset (0)=10 ("偏移量(0)"), length (rest)=14 ("长度（剩余）")) -> (substring=w1944:string)
                    n1582 = call "格式时间字符串.vi"("字符串"=w1944) -> ("连接的字符串"=w1945:string)  [unwired: 10 in]
                    n1583 = call "格式时间字符串.vi"("字符串"=w1943) -> ("连接的字符串"=w1942:string)  [unwired: 10 in]
                    n1584 = global write "全局 水样时间.vi" "时间"(w1945) -> ()
                    n1585 = global write "全局 时间2.vi" "时间2"(w1942) -> ()
                  }
                  frame #1 {
                    w1951 = "空白测试" ("新元素/子数组")
                    n1586 = call "从数据库获取数据通用可配置(子VI).vi"("table输入"=w1951, "列队名（唯一）"=w1951) -> ()  [unwired: 8 in, 2 out]
                  }
                  frame #2 {
                    # "数据处理整合"
                    n1587 = call "数据处理整合 (子VI).vi"("枚举"=enum16{"实时数据排序", "小时数据排序"}."实时数据排序") -> ("已排序的数组"=w1953:string[])  [unwired: 10 in]
                    n1588 = Array Size(array=w1953) -> (size(s)=w1954:i32)
                    n1589 = global write "全局 数据数组大小.vi" "数据数组大小"(w1954) -> ()
                  }
                  frame #3 {
                  }
                }
                n1590 = global write "全局 小时数据发送次数.vi" "小时数据发送次数"(w1939) -> ()
                n1591 = global write "全局1.vi" "枚举"(w1939) -> ()
              }
              frame "2066" {
                w1958 = 0 ("数值")
                n1592 = flat-sequence {
                  tunnel: [T6."发送数据" ("元素")] -> w1956
                  frame #0 {
                    # "格式时间"
                    # "2066、提取跨度核查数据"
                    n1593 = local read "数据"() -> (w1967:string)
                    n1594 = String Subset(string=w1967, offset (0)=33 ("偏移量(0)"), length (rest)=14 ("长度（剩余）")) -> (substring=w1962:string)
                    n1595 = String Subset(string=w1967, offset (0)=10 ("偏移量(0)"), length (rest)=14 ("长度（剩余）")) -> (substring=w1963:string)
                    n1596 = global write "全局 实时数据参数.vi" "实时数据参数"("跨度核查" ("新元素/子数组")) -> ()
                    n1597 = local write "table元素"("跨度核查" ("新元素/子数组")) -> ()
                    n1598 = call "格式时间字符串.vi"("字符串"=w1963) -> ("连接的字符串"=w1964:string)  [unwired: 10 in]
                    n1599 = call "格式时间字符串.vi"("字符串"=w1962) -> ("连接的字符串"=w1961:string)  [unwired: 10 in]
                    n1600 = global write "全局 水样时间.vi" "时间"(w1964) -> ()
                    n1601 = global write "全局 时间2.vi" "时间2"(w1961) -> ()
                  }
                  frame #1 {
                    w1970 = "跨度核查" ("新元素/子数组")
                    (unwired) "跨度核查" ("名称（未命名）")
                    # "提取COD、氨氮、多参数、总磷、总氮数据"
                    n1602 = call "从数据库获取数据通用可配置(子VI).vi"("table输入"=w1970, "列队名（唯一）"=w1970) -> ()  [unwired: 8 in, 2 out]
                  }
                  frame #2 {
                    # "数据处理整合"
                    n1603 = call "数据处理整合 (子VI).vi"("枚举"=enum16{"实时数据排序", "小时数据排序"}."实时数据排序") -> ("已排序的数组"=w1973:string[])  [unwired: 10 in]
                    n1604 = Array Size(array=w1973) -> (size(s)=w1972:i32)
                    n1605 = global write "全局 数据数组大小.vi" "数据数组大小"(w1972) -> ()
                  }
                  frame #3 {
                  }
                }
                n1606 = global write "全局 小时数据发送次数.vi" "小时数据发送次数"(w1958) -> ()
                n1607 = global write "全局1.vi" "枚举"(w1958) -> ()
              }
              frame "3015" {
                n1608 = flat-sequence {
                  tunnel: [T6."发送数据" ("元素")] -> w1975
                  frame #0 {
                    # "发命令给中控"
                    # "发回给平台"
                    # "3015、手动远程留样"
                    n1609 = local write "table元素"("超标留样返回" ("新元素/子数组")) -> ()
                    n1610 = Insert Into Array(array=u16[] [] ("holding register values"), index=0 ("索引"), new element=u16 1 ("新元素/子数组")) -> (w1979:u16[])
                    n1611 = call "Modbus Master.vi"("Unit ID"=u8 1, "读取写入选择"="写入", "holding register values"=w1979, "starting address"=u16 10) -> ()  [unwired: 6 in, 2 out]
                  }
                  frame #1 {
                  }
                }
              }
              frame "3020" {
                n1612 = flat-sequence {
                  tunnel: [w1995] -> w1989
                  tunnel: [w1996] -> w1988
                  tunnel: [w1994] -> w1987
                  tunnel: [w1992] -> w1986
                  tunnel: w1989 -> [w2045]
                  tunnel: w1988 -> [w2044]
                  tunnel: w1987 -> [w2043]
                  tunnel: w1986 -> [w2042]
                  tunnel: [T6."发送数据" ("元素")] -> w1990
                  frame #0 {
                    w2015 = 0 ("数值")
                    # "3020、提取日志、报警，仪器参数"
                    n1613 = local read "数据"() -> (w2016:string)
                    n1614 = Search/Split String(string=w2016, search string/char (-)="BeginTime=" ("搜索字符串")) -> (match + rest of string=w2014:string)  [unwired: 1 in, 2 out]
                    n1615 = local read "数据"() -> (w2000:string)
                    n1616 = case shown="\"\"" w2014 {
                      tunnel: ["1904/01/01 00:00:00" w2039] -> w2018
                      tunnel: w2014 -> [_ w2033]
                      tunnel: [w2026 w2034] -> w2013
                      frame "" {
                        # "时间"
                        n1617 = Get Date/Time In Seconds() -> (seconds since 1Jan1904=w2027:timestamp)
                        n1618 = Format Date/Time String(time format string (%c)="%Y%m%d%H%M%S%3u" ("时间格式字符串(%c)"), seconds (now)=w2027) -> (date/time string=w2031:string)  [unwired: 1 in]
                        n1619 = Search and Replace String(input string=w2031, search string="." ("搜索字符串")) -> (result string=w2030:string)  [unwired: 6 in, 3 out]
                        n1620 = call "格式时间字符串.vi"("字符串"=w2030) -> ("连接的字符串"=w2026:string)  [unwired: 10 in]
                      }
                      frame "真", Default {
                        # "格式时间"
                        n1621 = String Subset(string=w2033, offset (0)=33 ("偏移量(0)"), length (rest)=14 ("长度（剩余）")) -> (substring=w2037:string)
                        n1622 = String Subset(string=w2033, offset (0)=10 ("偏移量(0)"), length (rest)=14 ("长度（剩余）")) -> (substring=w2038:string)
                        n1623 = call "格式时间字符串.vi"("字符串"=w2037) -> ("连接的字符串"=w2034:string)  [unwired: 10 in]
                        n1624 = call "格式时间字符串.vi"("字符串"=w2038) -> ("连接的字符串"=w2039:string)  [unwired: 10 in]
                      }
                    }
                    n1625 = call "日志报警参数选择 (子VI).vi"("String输入"=w2000) -> ("输出簇"=w1999:T18)  [unwired: 9 in, 1 out]
                    n1626 = Unbundle By Name(w1999) -> ("高锰酸盐"=w2007:string, "化学需氧量"=w2008:string, "氨氮"=w2009:string, "总磷"=w2010:string, "总氮"=w2011:string, "数采仪"=w2012:string, "高锰酸盐"=w2001:bool, "化学需氧量"=w2002:bool, "氨氮"=w2003:bool, "总磷"=w2004:bool, "总氮"=w2005:bool, "数采仪"=w2006:bool)
                    n1627 = Build Array(w2007, w2008, w2009, w2010, w2011, w2012) -> (w1994:string[])
                    n1628 = global write "全局 时间2.vi" "时间2"(w2013) -> ()
                    n1629 = Build Array(w2001, w2002, w2003, w2004, w2005, w2006) -> (w1993:bool[])
                    n1630 = global write "全局 水样时间.vi" "时间"(w2018) -> ()
                    n1631 = Or Array Elements(Boolean array=w1993) -> (logical OR=w1992:bool)
                    n1632 = global write "全局 小时数据发送次数.vi" "小时数据发送次数"(w2015) -> ()
                    n1633 = Obtain Queue(name (unnamed)="操作日志报警信息" ("名称（未命名）"), element data type=T17."CODMn") -> (queue out=w1995:refnum<queue>, error out=w1996:errorcluster)  [unwired: 3 in, 1 out]
                    n1634 = case shown="假" w1992 {
                      tunnel: w1995 -> [_ w2020]
                      tunnel: w1993 -> [_ w2019]
                      frame False {
                      }
                      frame True {
                        n1635 = for {
                          tunnel: w2019 -> [w2022] mode=indexing
                          tunnel: w2020 -> [w2021]
                          i -> [w2023]
                          n1636 = case shown="真" w2022 {
                            tunnel: w2023 -> [_ w2025]
                            tunnel: w2021 -> [_ w2024]
                            frame False {
                            }
                            frame True {
                              n1637 = call "提取日志报警参数入列队 (子VI).vi"("枚举"=w2025, "queue in"=w2024) -> ()  [unwired: 10 in]
                            }
                          }
                        }
                      }
                    }
                    n1638 = global write "全局1.vi" "枚举"(w2015) -> ()
                  }
                  frame #1 {
                    # "按需求提取COD、氨氮、总磷、总氮日志"
                    # "按需求提取COD、氨氮、总磷、总氮日志"
                    n1639 = case shown="真" w2042 {
                      tunnel: w2044 -> [_ w2048]
                      tunnel: w2045 -> [_ w2047]
                      tunnel: w2043 -> [_ w2046]
                      frame False {
                      }
                      frame True {
                        n1640 = while {
                          shift-right: [w2062] -> _
                          shift-left: w2047 -> [w2063]
                          tunnel: w2048 -> [w2061]
                          tunnel: w2046 -> [w2056]
                          stop <- w2058 stop-if-true
                          n1641 = Dequeue Element(queue=w2063, error in (no error)=w2061) -> (queue out=w2060:refnum<queue>, element=w2055:T17)  [unwired: 1 in, 2 out]
                          n1642 = Index Array(array=w2056) -> (element #1=w2054:string, element #2=w2053:string, element #3=w2052:string, element #4=w2051:string, element #5=w2050:string, element #6=w2049:string)  [unwired: 6 in]
                          n1643 = case shown="\"CODCr\"" w2055 {
                            tunnel: w2060 -> [w2068 _ w2077 w2082 w2086 w2091]
                            tunnel: [w2068 _ w2077 w2082 w2086 w2091] -> w2062
                            tunnel: w2054 -> [w2065 _ _ _ _ _]
                            tunnel: w2053 -> [_ w2070 _ _ _ _]
                            tunnel: w2052 -> [_ _ w2074 _ _ _]
                            tunnel: w2051 -> [_ _ _ w2079 _ _]
                            tunnel: w2050 -> [_ _ _ _ w2084 _]
                            tunnel: w2049 -> [_ _ _ _ _ w2088]
                            frame "CODMn" {
                              w2064 = string[][] [] ("氨氮")
                              n1644 = call "数据表比对.vi"("仪器日志参数"="CODMn" ("元素"), "table输入"=w2065) -> ("待发送数据"=w2066:string[][])  [unwired: 6 in, 3 out]
                              n1645 = global write "全局 所有参数.vi" "CODMn"(w2066) -> ()
                              n1646 = global write "全局 所有参数.vi" "总氮"(w2064) -> ()
                              n1647 = global write "全局 所有参数.vi" "CODCr"(w2064) -> ()
                              n1648 = global write "全局 所有参数.vi" "总磷"(w2064) -> ()
                              n1649 = global write "全局 所有参数.vi" "氨氮"(w2064) -> ()
                            }
                            frame "CODCr" {
                              w2069 = string[][] [] ("氨氮")
                              n1650 = call "数据表比对.vi"("仪器日志参数"="CODCr" ("元素"), "table输入"=w2070) -> ("待发送数据"=w2071:string[][])  [unwired: 6 in, 3 out]
                              n1651 = global write "全局 所有参数.vi" "CODCr"(w2071) -> ()
                              n1652 = global write "全局 所有参数.vi" "CODMn"(w2069) -> ()
                              n1653 = global write "全局 所有参数.vi" "总氮"(w2069) -> ()
                              n1654 = global write "全局 所有参数.vi" "总磷"(w2069) -> ()
                              n1655 = global write "全局 所有参数.vi" "氨氮"(w2069) -> ()
                            }
                            frame "氨氮" {
                              w2073 = string[][] [] ("氨氮")
                              n1656 = call "数据表比对.vi"("仪器日志参数"="氨氮" ("元素"), "table输入"=w2074) -> ("待发送数据"=w2075:string[][])  [unwired: 6 in, 3 out]
                              n1657 = global write "全局 所有参数.vi" "氨氮"(w2075) -> ()
                              n1658 = global write "全局 所有参数.vi" "CODMn"(w2073) -> ()
                              n1659 = global write "全局 所有参数.vi" "总氮"(w2073) -> ()
                              n1660 = global write "全局 所有参数.vi" "CODCr"(w2073) -> ()
                              n1661 = global write "全局 所有参数.vi" "总磷"(w2073) -> ()
                            }
                            frame "总磷" {
                              w2078 = string[][] [] ("氨氮")
                              n1662 = call "数据表比对.vi"("仪器日志参数"="总磷" ("元素"), "table输入"=w2079) -> ("待发送数据"=w2080:string[][])  [unwired: 6 in, 3 out]
                              n1663 = global write "全局 所有参数.vi" "总磷"(w2080) -> ()
                              n1664 = global write "全局 所有参数.vi" "CODMn"(w2078) -> ()
                              n1665 = global write "全局 所有参数.vi" "总氮"(w2078) -> ()
                              n1666 = global write "全局 所有参数.vi" "CODCr"(w2078) -> ()
                              n1667 = global write "全局 所有参数.vi" "氨氮"(w2078) -> ()
                            }
                            frame "总氮" {
                              w2083 = string[][] [] ("氨氮")
                              n1668 = call "数据表比对.vi"("仪器日志参数"="总氮" ("元素"), "table输入"=w2084) -> ("待发送数据"=w2085:string[][])  [unwired: 6 in, 3 out]
                              n1669 = global write "全局 所有参数.vi" "总氮"(w2085) -> ()
                              n1670 = global write "全局 所有参数.vi" "CODMn"(w2083) -> ()
                              n1671 = global write "全局 所有参数.vi" "氨氮"(w2083) -> ()
                              n1672 = global write "全局 所有参数.vi" "CODCr"(w2083) -> ()
                              n1673 = global write "全局 所有参数.vi" "总磷"(w2083) -> ()
                            }
                            frame "数采仪" {
                              n1674 = call "数据表比对.vi"("仪器日志参数"="系统" ("元素"), "table输入"=w2088) -> ("待发送数据"=w2089:string[][])  [unwired: 6 in, 3 out]
                              n1675 = global write "全局 所有参数.vi" "DO"(w2089) -> ()
                            }
                          }
                          n1676 = Get Queue Status(queue=w2060) -> (# elements in queue=w2059:i32)  [unwired: 2 in, 7 out]
                          n1677 = Wait (ms)(milliseconds to wait=u32 300 ("等待时间（毫秒）")) -> ()  [unwired: 1 out]
                          n1678 = Equal To 0?(x=w2059) -> (x = 0?=w2058:bool)
                        }
                      }
                    }
                  }
                  frame #2 {
                    n1679 = local read "数据"() -> (w2100:string)
                    n1680 = Search/Split String(string=w2100, search string/char (-)="InfoId=" ("搜索字符串/字符(-)")) -> (match + rest of string=w2098:string)  [unwired: 1 in, 2 out]
                    n1681 = String Subset(string=w2098, offset (0)=7 ("偏移量(0)"), length (rest)=6 ("长度（剩余）")) -> (substring=w2094:string)
                    n1682 = case shown="\"i13001\", \"i13002\", \"i13003\", \"i13004\", \"i13005\", \"i13006\", \"i13007\", \"i13008\", \"i13009\", \"i13010\", \"i13011\", \"i13012\", \"i13013\"" w2094 {
                      selector: w2094 -> [_ w2105 _]
                      tunnel: ["操作日志" ("名称（未命名）") "提取仪器参数" ("名称（未命名）") "报警信息" ("名称（未命名）")] -> w2093
                      tunnel: [w2101 1 ("数据数组大小") w2108] -> w2092
                      frame "i11001", "i21001" {
                        # "数据处理整合"
                        # "i11001日志"
                        n1683 = call "数据处理整合 (子VI).vi"("枚举"=enum16{"实时数据排序", "小时数据排序"}."实时数据排序") -> ("已排序的数组"=w2102:string[])  [unwired: 10 in]
                        n1684 = Array Size(array=w2102) -> (size(s)=w2101:i32)
                      }
                      frame "i13001", "i13002", "i13003", "i13004", "i13005", "i13006", "i13007", "i13008", "i13009", "i13010", "i13011", "i13012", "i13013" {
                        n1685 = global write "全局 提取仪器参数.vi" "参数编码"(w2105) -> ()
                        n1686 = call "数据处理直接插入整合 (子VI).vi"() -> ()  [unwired: 12 in]
                      }
                      frame "i12001", Default {
                        # "数据处理整合"
                        # "i12001状态"
                        n1687 = call "数据处理整合 (子VI).vi"("枚举"=enum16{"实时数据排序", "小时数据排序"}."实时数据排序") -> ("已排序的数组"=w2109:string[])  [unwired: 10 in]
                        n1688 = Array Size(array=w2109) -> (size(s)=w2108:i32)
                      }
                    }
                    n1689 = global write "全局 数据数组大小.vi" "数据数组大小"(w2092) -> ()
                    n1690 = local write "table元素"(w2093) -> ()
                  }
                }
              }
              frame "3021" {
                # "设置仪表参数"
                n1691 = local write "table元素"("反控命令" ("新元素/子数组")) -> ()
              }
              frame "3040" {
                # "提取现场系统信息（3040）"
                n1692 = flat-sequence {
                  tunnel: [T6."发送数据" ("元素")] -> w2115
                  frame #0 {
                    n1693 = local write "table元素"("提取现场系统信息" ("新元素/子数组")) -> ()
                  }
                  frame #1 {
                  }
                }
              }
              frame "3041" {
                # "提取现场经纬度及环境信息（3041）"
                n1694 = flat-sequence {
                  tunnel: [T6."发送数据" ("元素")] -> w2119
                  frame #0 {
                    n1695 = call "获取环境参数 (子VI).vi"() -> ()  [unwired: 12 in]
                    n1696 = local write "table元素"("提取经纬度环境信息" ("新元素/子数组")) -> ()
                  }
                  frame #1 {
                  }
                }
              }
              frame "3042" {
                # "发命令给中控"
                # "反控指令"
                # "0维护，1常规，2应急，3质控"
                # "反控指令\n切换运行模式"
                n1697 = local write "table元素"("反控命令" ("新元素/子数组")) -> ()
                n1698 = property on="数据" class="Str"() -> ("Value"=w2138:string)  [unwired: 2 in, 2 out]
                n1699 = Search/Split String(string=w2138, search string/char (-)="RunMode" ("搜索字符串/字符(-)")) -> (match + rest of string=w2136:string)  [unwired: 1 in, 2 out]
                n1700 = String Subset(string=w2136, offset (0)=8 ("偏移量(0)"), length (rest)=1 ("长度（剩余）")) -> (substring=w2133:string)
                n1701 = case shown="\"2\"" w2133 {
                  tunnel: [u16 0 ("新元素/子数组") u16 1 ("新元素/子数组") u16 2 ("新元素/子数组") u16 3 ("新元素/子数组")] -> w2127
                  frame "0", Default {
                  }
                  frame "1" {
                  }
                  frame "2" {
                  }
                  frame "3" {
                  }
                }
                n1702 = Insert Into Array(array=u16[] [] ("holding register values"), index=0 ("索引"), new element=w2127) -> (w2128:u16[])
                n1703 = call "Modbus Master.vi"("Unit ID"=u8 1, "读取写入选择"="写入", "holding register values"=w2128, "starting address"=u16 0) -> ()  [unwired: 6 in, 2 out]
              }
              frame "3043" {
                # "远程重启数采仪"
                n1704 = local write "table元素"("反控命令" ("新元素/子数组")) -> ()
              }
              frame "3044" {
                # "发回给平台"
                # "反控指令"
                # "3042~3086"
                # "反控指令\n单次测量"
                # "3044"
                n1705 = local write "table元素"("反控命令" ("新元素/子数组")) -> ()
                n1706 = flat-sequence {
                  frame #0 {
                    # "发命令给中控"
                    n1707 = call "Modbus Master.vi"("Unit ID"=u8 1, "读取写入选择"="写入", "holding register values"=u16[] [1], "starting address"=u16 2) -> ()  [unwired: 6 in, 2 out]
                  }
                  frame #1 {
                    n1708 = Wait (ms)(milliseconds to wait=u32 500 ("等待时间（毫秒）")) -> ()  [unwired: 1 out]
                  }
                  frame #2 {
                    n1709 = call "Modbus Master.vi"("Unit ID"=u8 1, "读取写入选择"="写入", "holding register values"=u16[] [0], "starting address"=u16 2) -> ()  [unwired: 6 in, 2 out]
                  }
                }
              }
              frame "3045", "3046" {
                # "发回给平台"
                # "反控指令"
                # "3042~3086"
                # "反控指令\n急停"
                # "3045"
                n1710 = flat-sequence {
                  frame #0 {
                    # "发命令给中控"
                    n1711 = call "Modbus Master.vi"("Unit ID"=u8 1, "读取写入选择"="写入", "holding register values"=u16[] [1], "starting address"=u16 3) -> ()  [unwired: 6 in, 2 out]
                  }
                  frame #1 {
                    n1712 = Wait (ms)(milliseconds to wait=u32 500 ("等待时间（毫秒）")) -> ()  [unwired: 1 out]
                  }
                  frame #2 {
                    n1713 = call "Modbus Master.vi"("Unit ID"=u8 1, "读取写入选择"="写入", "holding register values"=u16[] [0], "starting address"=u16 3) -> ()  [unwired: 6 in, 2 out]
                  }
                }
                n1714 = local write "table元素"("反控命令" ("新元素/子数组")) -> ()
              }
              frame "3056" {
                # "发命令给中控"
                # "设置测量时间间隔"
                # "发回给平台"
                n1715 = property on="数据" class="Str"() -> ("Value"=w2176:string)  [unwired: 2 in, 2 out]
                n1716 = local write "table元素"("反控命令" ("新元素/子数组")) -> ()
                n1717 = Search/Split String(string=w2176, search string/char (-)="RunInterval" ("搜索字符串/字符(-)")) -> (match + rest of string=w2177:string)  [unwired: 1 in, 2 out]
                n1718 = Decimal String To Number(string=w2177, offset=12 ("偏移量(0)")) -> (number=w2172:i32)  [unwired: 1 in, 1 out]
                n1719 = Insert Into Array(array=u16[] [] ("holding register values"), index=0 ("索引"), new element=w2172) -> (w2171:u16[])
                n1720 = call "Modbus Master.vi"("Unit ID"=u8 1, "读取写入选择"="写入", "holding register values"=w2171, "starting address"=u16 14) -> ()  [unwired: 6 in, 2 out]
              }
              frame "3080", "3081", "3082", "3083", "3084", "3085", "3086" {
                # "30 启动标液核查  1CODmn  2 氨氮  3总磷  4总氮  5CODCr\n31 加标回收\n32 平行样测试\n33 零点核查\n34 跨度核查\n35 校零\n36 校标"
                # "发回给平台"
                n1721 = flat-sequence {
                  tunnel: w2186 -> [w2192]
                  tunnel: [w2190] -> w2185
                  tunnel: w2185 -> [w2218]
                  tunnel: [w2218] -> w2184
                  tunnel: w2184 -> [w2221]
                  frame #0 {
                    # "1CODmn  2 氨氮  3总磷  4总氮  5CODCr"
                    # "启动单台仪器标液核查"
                    # "发命令给中控"
                    n1722 = property on="数据" class="Str"() -> ("Value"=w2202:string)  [unwired: 2 in, 2 out]
                    n1723 = Search/Split String(string=w2202, search string/char (-)="PolId" ("搜索字符串/字符(-)")) -> (match + rest of string=w2197:string)  [unwired: 1 in, 2 out]
                    n1724 = String Subset(string=w2197, offset (0)=6 ("偏移量(0)"), length (rest)=6 ("长度（剩余）")) -> (substring=w2194:string)
                    n1725 = case shown="\"w01019\"" w2194 {
                      tunnel: [0 ("长度（剩余）") 1 ("长度（剩余）") 2 ("长度（剩余）") 3 ("长度（剩余）") 4 ("长度（剩余）") 5 ("长度（剩余）")] -> w2193
                      frame "", Default {
                      }
                      frame "w01019" {
                      }
                      frame "w21003" {
                      }
                      frame "w21011" {
                      }
                      frame "w21001" {
                      }
                      frame "w01018" {
                      }
                    }
                    n1726 = Insert Into Array(array=u16[] [] ("holding register values"), index=0 ("索引"), new element=w2193) -> (w2198:u16[])
                    n1727 = case shown="\"3086\"" w2192 {
                      tunnel: [u16 99 ("starting address") u16 30 ("starting address") u16 31 ("starting address") u16 32 ("starting address") u16 33 ("starting address") u16 34 ("starting address") u16 35 ("starting address") u16 36 ("starting address")] -> w2190
                      frame "", Default {
                      }
                      frame "3080" {
                      }
                      frame "3081" {
                      }
                      frame "3082" {
                      }
                      frame "3083" {
                      }
                      frame "3084" {
                      }
                      frame "3085" {
                      }
                      frame "3086" {
                      }
                    }
                    n1728 = call "Modbus Master.vi"("Unit ID"=u8 1, "读取写入选择"="写入", "holding register values"=w2198, "starting address"=w2190) -> ()  [unwired: 6 in, 2 out]
                  }
                  frame #1 {
                    n1729 = Wait (ms)(milliseconds to wait=u32 500 ("等待时间（毫秒）")) -> ()  [unwired: 1 out]
                  }
                  frame #2 {
                    n1730 = call "Modbus Master.vi"("Unit ID"=u8 1, "读取写入选择"="写入", "holding register values"=u16[] [0], "starting address"=w2221) -> ()  [unwired: 6 in, 2 out]
                  }
                }
                n1731 = local write "table元素"("反控命令" ("新元素/子数组")) -> ()
              }
            }
            n1732 = Enqueue Element(queue=w1789, element=w1788, timeout in ms (-1)=1000 ("超时毫秒(-1)")) -> ()  [unwired: 1 in, 3 out]
          }
          frame "发送数据" {
            # "table输入，选择命令编码、发送哪些数据"
            n1733 = local read "table元素"() -> (w2228:string)
            n1734 = case shown="\"报警信息\", \"操作日志\", \"核查数据\", \"空白测试\", \"跨度核查\", \"零点核查\", \"实时数据\", \"提取加标回收\", \"提取实时数据\", \"提取小时数据\", \"提取仪器参数\", \"仪器参数\"" w2228 {
              tunnel: w2227 -> [w2239 w2243 w2245 w2252]
              tunnel: [w2237 w2242 w2246 w2250] -> w2225
              tunnel: [w2238 w2241 w2247 w2251] -> w2226
              frame "", Default {
                n1735 = Increment(x=w2239) -> (x+1=w2238:i32)
                n1736 = global write "全局1.vi" "枚举"(w2239) -> ()
                n1737 = Greater Or Equal?(x=w2238, y=3) -> (x >= y?=w2237:bool)
              }
              frame "反控命令" {
                n1738 = Increment(x=w2243) -> (x+1=w2241:i32)
                n1739 = global write "全局 反控命令枚举.vi" "反控命令枚举"(w2243) -> ()
                n1740 = Greater Or Equal?(x=w2241, y=2) -> (x >= y?=w2242:bool)
              }
              frame "超标留样返回", "提取监测仪表时间", "提取经纬度环境信息", "提取现场系统信息" {
                n1741 = Increment(x=w2245) -> (x+1=w2247:i32)
                n1742 = global write "全局1.vi" "枚举"(w2245) -> ()
                n1743 = Greater Or Equal?(x=w2247, y=3) -> (x >= y?=w2246:bool)
              }
              frame "报警信息", "操作日志", "核查数据", "空白测试", "跨度核查", "零点核查", "实时数据", "提取加标回收", "提取实时数据", "提取小时数据", "提取仪器参数", "仪器参数" {
                n1744 = global read "全局 小时数据发送次数.vi" "小时数据发送次数"() -> (w2254:i32)
                n1745 = global read "全局 数据数组大小.vi" "数据数组大小"() -> (w2249:i32)
                n1746 = Greater Or Equal?(x=w2254, y=w2249) -> (x >= y?=w2255:bool)
                n1747 = case shown="真" w2255 {
                  tunnel: w2252 -> [w2260 w2267]
                  tunnel: [w2260 w2261] -> w2256
                  frame False {
                  }
                  frame True {
                    n1748 = global read "全局 小时数据发送次数.vi" "小时数据发送次数"() -> (w2266:i32)
                    n1749 = global read "全局 数据数组大小.vi" "数据数组大小"() -> (w2263:i32)
                    n1750 = Equal To 0?(x=w2263) -> (x = 0?=w2264:bool)
                    n1751 = Equal To 0?(x=w2266) -> (x = 0?=w2265:bool)
                    n1752 = And(x=w2265, y=w2264) -> (x .and. y?=w2262:bool)
                    n1753 = case shown="假" w2262 {
                      tunnel: w2267 -> [w2269 _]
                      tunnel: [w2268 0 ("索引")] -> w2261
                      frame False {
                        n1754 = Increment(x=w2269) -> (x+1=w2268:i32)
                      }
                      frame True {
                      }
                    }
                  }
                }
                n1755 = Equal To 0?(x=w2256) -> (x = 0?=w2257:bool)
                n1756 = global write "全局1.vi" "枚举"(w2256) -> ()
                n1757 = case shown="真" w2257 {
                  tunnel: w2256 -> [w2258 _]
                  tunnel: [w2258 1] -> w2251
                  frame False {
                  }
                  frame True {
                  }
                }
                n1758 = Greater Or Equal?(x=w2251, y=2) -> (x >= y?=w2250:bool)
              }
            }
            n1759 = case shown="假" w2225 {
              tunnel: w2226 -> [w2271 _]
              tunnel: [w2271 1 ("索引")] -> w2230
              frame False {
              }
              frame True {
              }
            }
            n1760 = flat-sequence {
              tunnel: "table元素" -> [w2280]
              tunnel: w2234 -> [w2279]
              tunnel: [w2275] -> w2233
              tunnel: [w2284] -> w2231
              tunnel: w2233 -> [w2284]
              tunnel: w2232 -> [w2283]
              tunnel: w2225 -> [w2282]
              frame #0 {
                # "数据记录"
                # "数据编码"
                n1761 = local read "QN"() -> (w2278:string)
                n1762 = call "数据编码.vi"("table输入"=w2280, "错误常量 2"=w2279, "QN"=w2278) -> ("错误常量"=w2277:errorcluster, "通讯包字符串"=w2276:string)  [unwired: 11 in]
                n1763 = local read "数据发送通道"() -> (w2274:enum16{"TCP", "VISA"})
                n1764 = call "数据记录.vi"("写入字段"=w2276) -> ("连接的字符串"=→"发送报文显示":string)  [unwired: 10 in]
                n1765 = call "VISATCP组合选择发送.vi"("数据发送通道"=w2274, "命令"="write", "error in (no error)"=w2277, "写入缓冲区"=w2276) -> ("错误输出"=w2275:errorcluster)  [unwired: 8 in, 3 out]
              }
              frame #1 {
                n1766 = case shown="真" w2282 {
                  tunnel: w2283 -> [w2285 w2297]
                  frame False {
                    n1767 = Enqueue Element(queue=w2285, element=T6."发送数据" ("元素")) -> ()  [unwired: 2 in, 3 out]
                  }
                  frame True {
                    n1768 = local read "TCP服务端掉线计数"() -> (w2292:i32)
                    n1769 = Obtain Queue(name (unnamed)="重发掉线数据" ("名称（未命名）"), element data type=T16."水样测试") -> (queue out=w2290:refnum<queue>, error out=w2291:errorcluster)  [unwired: 3 in, 1 out]
                    n1770 = Get Queue Status(queue=w2290, error in (no error)=w2291) -> (# elements in queue=w2294:i32)  [unwired: 1 in, 7 out]
                    n1771 = Not Equal To 0?(x=w2294) -> (x != 0?=w2295:bool)
                    n1772 = Greater Or Equal?(x=w2292, y=1) -> (x >= y?=w2296:bool)
                    n1773 = And(x=w2295, y=w2296) -> (x .and. y?=w2288:bool)
                    n1774 = case shown="真" w2288 {
                      tunnel: [T6."读取数据" ("元素") T6."表格比对" ("元素")] -> w2298
                      frame False {
                      }
                      frame True {
                      }
                    }
                    n1775 = Enqueue Element(queue=w2297, element=w2298) -> ()  [unwired: 2 in, 3 out]
                  }
                }
              }
            }
            "查询数据发送" <- TRUE
          }
          frame "数据处理" {
            n1776 = local write "空闲时间"(0.0 ("空闲时间")) -> ()
            n1777 = local read "心跳包"() -> (w2309:bool)
            n1778 = Equal?(x=w2307, y="实时数据") -> (x = y?=w2305:bool)
            n1779 = case shown="假" w2309 {
              tunnel: w2313 -> [w2316 _]
              tunnel: w2307 -> [w2315 _]
              frame False {
                n1780 = call "插入单条数据.vi"("table输入"=w2315, "插入数据"=w2316) -> ()  [unwired: 8 in, 2 out]
              }
              frame True {
              }
            }
            n1781 = Select(t=0, s=w2305, f=w2303) -> (s? t:f=w2304:i32)
            n1782 = Enqueue Element(queue=w2312, element=T6."表格比对" ("元素"), timeout in ms (-1)=1000 ("超时毫秒(-1)")) -> ()  [unwired: 1 in, 3 out]
          }
        }
      }
      frame Error {
        n1783 = Unbundle By Name(w2320) -> ("code"=w2319:i32)
        n1784 = case shown="63" w2319 {
          tunnel: w2320 -> [w2325 w2335 w2368 w2396]
          tunnel: [w2331 w2351 w2384 w2396] -> w2324
          tunnel: w2318 -> [w2332 w2346 w2379 w2393]
          frame 0, Default {
            n1785 = Flush Queue(queue=w2332) -> (queue out=w2330:refnum<queue>)  [unwired: 1 in, 2 out]
            n1786 = Enqueue Element(queue=w2330, element=T6."初始化" ("元素"), timeout in ms (-1)=1000 ("超时毫秒(-1)")) -> ()  [unwired: 1 in, 3 out]
            n1787 = local read "数据发送通道"() -> (w2327:enum16{"TCP", "VISA"})
            n1788 = call "VISATCP组合选择发送.vi"("数据发送通道"=w2327, "命令"="close", "error in (no error)"=w2325) -> ("错误输出"=w2326:errorcluster)  [unwired: 9 in, 3 out]
            n1789 = call <vilib>:"Clear Errors.vi"("error in (no error)"=w2326) -> ("error out"=w2331:errorcluster)  [unwired: 5 in, 1 out]
            n1790 = global write "全局 数据发送重叠.vi" "掉线指示灯"(TRUE ("掉线指示灯")) -> ()
          }
          frame 63 {
            # "TCP服务器端口掉线"
            n1791 = Flush Queue(queue=w2346) -> (queue out=w2347:refnum<queue>)  [unwired: 1 in, 2 out]
            n1792 = local read "查询数据发送"() -> (w2343:bool)
            n1793 = property on="TCP服务端掉线计数" class="DigNum (严格)"() -> ("Value"=w2342:i32)  [unwired: 2 in, 2 out]
            n1794 = call <vilib>:"Boolean Crossing PtByPt.vi"("direction"=enum16{"either", "false-true", "true-false"}."false-true", "input"=w2343) -> ("crossing"=w2344:bool)  [unwired: 1 in]
            n1795 = Less Or Equal?(x=w2342, y=1) -> (x <= y?=w2340:bool)
            n1796 = Enqueue Element(queue=w2347, element=T6."初始化" ("元素"), timeout in ms (-1)=1000 ("超时毫秒(-1)")) -> ()  [unwired: 1 in, 3 out]
            n1797 = case shown="真" w2344 {
              frame False {
              }
              frame True {
                n1798 = disable-structure shown="禁用" {
                  frame Disabled {
                    # "判定数据为空时不写入临时表格"
                    n1799 = call "每个元素都写入临时表格 (子VI).vi"("组合框"="小时数据存储") -> ()  [unwired: 10 in, 1 out]
                  }
                  frame Enabled {
                  }
                }
              }
            }
            n1800 = case shown="真" w2340 {
              frame False {
                n1801 = global write "全局 数据发送重叠.vi" "TCP掉线时间节点"("TCP掉线时间节点") -> ()
                n1802 = local write "TCP掉线时间节点"("TCP掉线时间节点") -> ()
              }
              frame True {
                n1803 = Get Date/Time In Seconds() -> (seconds since 1Jan1904=w2364:timestamp)
                n1804 = Format Date/Time String(time format string (%c)="%Y%m%d%H%M%S%3u" ("时间格式字符串(%c)"), seconds (now)=w2364) -> (date/time string=w2366:string)  [unwired: 1 in]
                n1805 = call "格式时间字符串.vi"("字符串"=w2366) -> ("连接的字符串"=w2354:string)  [unwired: 10 in]
                n1806 = local write "TCP掉线时间节点"(w2354) -> ()
                n1807 = call <vilib>:"Application Directory.vi"() -> ("Application Directory"=w2362:path)
                n1808 = Build Path(base path=w2362, name or relative path="data\\Set.ini" ("名称或相对路径")) -> (appended path=w2363:path)
                n1809 = call <vilib>:"Open Config Data.vi"("configuration file path"=w2363) -> ("error out"=w2359:errorcluster, "refnum"=w2360:T8)  [unwired: 8 in, 1 out]
                n1810 = call-poly <vilib>:"Write Key.vi"("section"="掉线时间存储", "error in (no error)"=w2359, "value"=w2354, "key"="掉线时间", "refnum"=w2360) -> ("error out"=w2357:errorcluster, "refnum out"=w2358:T8)  [unwired: 4 in, 1 out]
                n1811 = call <vilib>:"Close Config Data.vi"("error in (no error)"=w2357, "refnum"=w2358) -> ()  [unwired: 8 in, 2 out]
              }
            }
            n1812 = local read "数据发送通道"() -> (w2337:enum16{"TCP", "VISA"})
            n1813 = call "VISATCP组合选择发送.vi"("数据发送通道"=w2337, "命令"="close", "error in (no error)"=w2335) -> ("错误输出"=w2336:errorcluster)  [unwired: 9 in, 3 out]
            n1814 = call <vilib>:"Clear Errors.vi"("error in (no error)"=w2336) -> ("error out"=w2351:errorcluster)  [unwired: 5 in, 1 out]
            n1815 = global write "全局 数据发送重叠.vi" "掉线指示灯"(TRUE ("掉线指示灯")) -> ()
            n1816 = property on="TCP服务端掉线计数" class="DigNum (严格)"() -> ("Value"=w2350:i32)  [unwired: 2 in, 2 out]
            n1817 = Increment(x=w2350) -> (x+1=w2348:i32)
            n1818 = property on="TCP服务端掉线计数" class="DigNum (严格)"("Value"=w2348) -> ()  [unwired: 2 in, 2 out]
          }
          frame 54 {
            # "TCP服务器端口掉线"
            n1819 = local read "查询数据发送"() -> (w2376:bool)
            n1820 = Flush Queue(queue=w2379) -> (queue out=w2380:refnum<queue>)  [unwired: 1 in, 2 out]
            n1821 = property on="TCP服务端掉线计数" class="DigNum (严格)"() -> ("Value"=w2375:i32)  [unwired: 2 in, 2 out]
            n1822 = call <vilib>:"Boolean Crossing PtByPt.vi"("direction"=enum16{"either", "false-true", "true-false"}."false-true", "input"=w2376) -> ("crossing"=w2377:bool)  [unwired: 1 in]
            n1823 = Less Or Equal?(x=w2375, y=1) -> (x <= y?=w2373:bool)
            n1824 = Enqueue Element(queue=w2380, element=T6."初始化" ("元素"), timeout in ms (-1)=1000 ("超时毫秒(-1)")) -> ()  [unwired: 1 in, 3 out]
            n1825 = case shown="真" w2377 {
              frame False {
              }
              frame True {
                n1826 = disable-structure shown="禁用" {
                  frame Disabled {
                    # "判定数据为空时不写入临时表格"
                    n1827 = call "每个元素都写入临时表格 (子VI).vi"("组合框"="小时数据存储") -> ()  [unwired: 10 in, 1 out]
                  }
                  frame Enabled {
                  }
                }
              }
            }
            n1828 = case shown="真" w2373 {
              frame False {
                n1829 = local read "TCP掉线时间节点"() -> (w2386:string)
                n1830 = global write "全局 数据发送重叠.vi" "TCP掉线时间节点"(w2386) -> ()
                n1831 = local write "TCP掉线时间节点"(w2386) -> ()
              }
              frame True {
                n1832 = Get Date/Time In Seconds() -> (seconds since 1Jan1904=w2388:timestamp)
                n1833 = Format Date/Time String(time format string (%c)="%Y%m%d%H%M%S%3u" ("时间格式字符串(%c)"), seconds (now)=w2388) -> (date/time string=w2390:string)  [unwired: 1 in]
                n1834 = call "格式时间字符串.vi"("字符串"=w2390) -> ("连接的字符串"=w2387:string)  [unwired: 10 in]
                n1835 = local write "TCP掉线时间节点"(w2387) -> ()
              }
            }
            n1836 = local read "数据发送通道"() -> (w2370:enum16{"TCP", "VISA"})
            n1837 = property on="TCP服务端掉线计数" class="DigNum (严格)"() -> ("Value"=w2383:i32)  [unwired: 2 in, 2 out]
            n1838 = call "VISATCP组合选择发送.vi"("数据发送通道"=w2370, "命令"="close", "error in (no error)"=w2368) -> ("错误输出"=w2369:errorcluster)  [unwired: 9 in, 3 out]
            n1839 = Increment(x=w2383) -> (x+1=w2381:i32)
            n1840 = property on="TCP服务端掉线计数" class="DigNum (严格)"("Value"=w2381) -> ()  [unwired: 2 in, 2 out]
            n1841 = call <vilib>:"Clear Errors.vi"("error in (no error)"=w2369) -> ("error out"=w2384:errorcluster)  [unwired: 5 in, 1 out]
            n1842 = global write "全局 数据发送重叠.vi" "掉线指示灯"(TRUE ("掉线指示灯")) -> ()
          }
          frame 56 {
            n1843 = Flush Queue(queue=w2393) -> (queue out=w2394:refnum<queue>)  [unwired: 1 in, 2 out]
            n1844 = Enqueue Element(queue=w2394, element=T6."读取数据" ("元素"), timeout in ms (-1)=1000 ("超时毫秒(-1)")) -> ()  [unwired: 1 in, 3 out]
          }
        }
        n1845 = call <vilib>:"Clear Errors.vi"("error in (no error)"=w2324) -> ("error out"=w2323:errorcluster)  [unwired: 5 in, 1 out]
      }
    }
  }
  n1846 = register-events(error in=w17, w18) -> (reference out=w6:refnum<event-registration>, error out=w5:errorcluster)  [unwired: 1 in]
  n1847 = while {
    shift-right: [w2400] -> w9
    shift-left: w5 -> [w2399]
    shift-right: [w2401] -> w12
    shift-left: w7 -> [w2402]
    shift-right: [w2398] -> w11
    shift-left: w6 -> [w2403]
    tunnel: [w2397] -> _
    stop <- w2397 stop-if-true
    n1848 = case shown="无错误" w2399 {
      selector: w2399 -> [w2405 w2439]
      tunnel: w2403 -> [w2410 w2434]
      tunnel: w2402 -> [w2409 w2435]
      tunnel: [w2408 w2435] -> w2401
      tunnel: [w2407 w2437] -> w2400
      tunnel: [w2406 FALSE ("Discard?")] -> w2397
      tunnel: [w2404 w2434] -> w2398
      frame No Error {
        n1849 = event shown="[0] <Public:SelectedItemEvent>: 用户事件" {
          selector: w2410 -> [_ _ _]
          dyn-events: [_ _ _] -> w2404
          timeout: _ -> [_ _ _]
          tunnel: w2405 -> [w2413 w2423 w2432]
          tunnel: [w2413 w2423 w2431] -> w2407
          tunnel: [w2412 TRUE FALSE ("Discard?")] -> w2406
          tunnel: w2409 -> [w2411 w2421 w2433]
          tunnel: [w2411 w2421 w2430] -> w2408
          event User Event {
            # "5."
            n1850 = event-data() -> ("ItemTag"=w2414:string)  [unwired: 1 in]
            n1851 = case shown="\"EXIT线程一\"" w2414 {
              tunnel: [FALSE TRUE] -> w2412
              frame Default {
                n1852 = Current VI's Path() -> (path=w2415:path)
                n1853 = Open VI Reference(vi path=w2415) -> (vi reference=w2416:refnum<vi>)  [unwired: 5 in, 1 out]
                n1854 = invoke class="VI" method="FP.Open"(reference=w2416, "Activate"=TRUE ("激活？")) -> ()  [unwired: 3 in, 5 out]
              }
              frame "EXIT线程一" {
              }
            }
          }
          event "停止 2": Value Change {
            # "5."
            n1855 = event-data() -> ()  [unwired: 1 in, 2 out]
            n1856 = Stop(stop? (T)=TRUE ("可见")) -> ()
          }
          event Panel Close? {
            # "4."
            n1857 = event-data() -> ("VIRef"=w2426:refnum<vi>)  [unwired: 1 in, 3 out]
            n1858 = invoke class="VI" method="FP.Open"(reference=w2426, "State"=T15."Hidden" ("状态")) -> ()  [unwired: 3 in, 5 out]
            n1859 = call <vilib>:"ShowBalloonTip.vi"("Balloon Icon"=BalloonIcon."Information", "error in"=w2432, "Text"="欢迎使用平台发送系统", "NotifyIcon in"=w2433) -> ("error out"=w2431:errorcluster, "NotifyIcon out"=w2430:refnum<class "NotifyIcon.lvclass">)  [unwired: 6 in]
            n1860 = event-data("Discard?"=TRUE ("放弃？")) -> ()  [unwired: 1 in, 1 out]
          }
        }
      }
      frame Error {
        n1861 = call <vilib>:"Simple Error Handler.vi"("error in (no error)"=w2439) -> ("error out"=w2438:errorcluster)  [unwired: 4 in, 4 out]
        n1862 = call <vilib>:"Clear Errors.vi"("error in (no error)"=w2438) -> ("error out"=w2437:errorcluster)  [unwired: 5 in, 1 out]
      }
    }
  }
  n1863 = Unregister For Events(event registration refnum=w11, error in=w9) -> (error out=w8:errorcluster)
  n1864 = property class="App"() -> ("App.Kind"=w13:T14)  [unwired: 2 in, 2 out]
  n1865 = call <vilib>:"Destructor.vi"("error in"=w8, "NotifyIcon"=w12) -> ("error out"=w14:errorcluster)  [unwired: 9 in]
  n1866 = case shown="\"Development System\"" w13 {
    tunnel: w14 -> [_ _ _ _ _ _ _]
    frame "invalid app kind", Default {
    }
    frame "Development System" {
      n1867 = Stop(stop? (T)=TRUE ("可见")) -> ()
    }
    frame "Run Time System" {
      n1868 = Quit LabVIEW(quit? (T)=TRUE ("退出？(T)")) -> ()
    }
    frame "Student Edition" {
    }
    frame "Embedded LabVIEW" {
    }
    frame "Evaluation" {
    }
    frame "Custom" {
    }
  }
  n1869 = call <vilib>:"Simple Error Handler.vi"("error in (no error)"=w14) -> ("error out"=→"error out":errorcluster)  [unwired: 4 in, 4 out]
